vi "Beampointing_Multi_Pico.vi"() -> ()   [LabVIEW 2011]
uses:
  GUI_Template/GUI_master/tcp_new_data_event.ctl
  GUI_Template/GUI_master/tcp new data cluster.ctl
  Ctrs/beam detection.ctl
  GUI_Beampointing_single_TRA/Ctrs/move.ctl
  <vilib>/Utility/file.llb/Read From Spreadsheet File (string).vi
  <userlib>/_OpenG.lib/array/array.llb/Filter 1D Array with Scalar (String)__ogtk.vi
  <vilib>/Utility/file.llb/Write To Spreadsheet File (string).vi
  <vilib>/Analysis/NI_AALBase.lvlib
panel:
  out "millisecond timer value":u32
  out "appended path":path
  out "millisecond timer 2":u32
  in  "GUIdevice 98":string="PicoPad4"
  in  "Position.Axis 111::98":dbl=77.0 caption="Motor Axis 1" min=-20000.0 max=20000.0 format="%#_6f"
  in  "Position.Axis 112::98":dbl=77.0 caption="Motor Axis 1" min=-20000.0 max=20000.0 format="%#_6f"
  in  "Position.Axis 113::98":dbl=77.0 caption="Motor Axis 1" min=-20000.0 max=20000.0 format="%#_6f"
  in  "Position.Axis 121::98":dbl=77.0 caption="Motor Axis 1" min=-999999.0 max=999999.0 format="%#_6f"
  in  "Position.Axis 122::98":dbl=77.0 caption="Motor Axis 1" min=-999999.0 max=999999.0 format="%#_6f"
  in  "Position.Axis 123::98":dbl=77.0 caption="Motor Axis 1" min=-999999.0 max=999999.0 format="%#_6f"
  in  "Position.Axis 131::98":dbl=77.0 caption="Motor Axis 1" min=-999999.0 max=999999.0 format="%#_6f"
  in  "Position.Axis 132::98":dbl=77.0 caption="Motor Axis 1" min=-999999.0 max=999999.0 format="%#_6f"
  in  "Position.Axis 133::98":dbl=77.0 caption="Motor Axis 1" min=-999999.0 max=999999.0 format="%#_6f"
  in  "Position.Axis 141::98":dbl=77.0 caption="Motor Axis 1" min=-999999.0 max=999999.0 format="%#_6f"
  in  "Position.Axis 142::98":dbl=77.0 caption="Motor Axis 1" min=-999999.0 max=999999.0 format="%#_6f"
  in  "Position.Axis 143::98":dbl=77.0 caption="Motor Axis 1" min=-999999.0 max=999999.0 format="%#_6f"
  in  "Position.Axis 211::98":dbl=77.0 caption="Motor Axis 1" min=-999999.0 max=999999.0 format="%#_6f"
  in  "Position.Axis 212::98":dbl=77.0 caption="Motor Axis 1" min=-999999.0 max=999999.0 format="%#_6f"
  in  "Position.Axis 213::98":dbl=77.0 caption="Motor Axis 1" min=-999999.0 max=999999.0 format="%#_6f"
  in  "Position.Axis 221::98":dbl=77.0 caption="Motor Axis 1" min=-999999.0 max=999999.0 format="%#_6f"
  in  "Position.Axis 222::98":dbl=77.0 caption="Motor Axis 1" min=-999999.0 max=999999.0 format="%#_6f"
  in  "Position.Axis 223::98":dbl=77.0 caption="Motor Axis 1" min=-999999.0 max=999999.0 format="%#_6f"
  in  "Position.Axis 231::98":dbl=77.0 caption="Motor Axis 1" min=-999999.0 max=999999.0 format="%#_6f"
  in  "Position.Axis 232::98":dbl=77.0 caption="Motor Axis 1" min=-999999.0 max=999999.0 format="%#_6f"
  in  "Position.Axis 233::98":dbl=77.0 caption="Motor Axis 1" min=-999999.0 max=999999.0 format="%#_6f"
  in  "Position.Axis 241::98":dbl=77.0 caption="Motor Axis 1" min=-999999.0 max=999999.0 format="%#_6f"
  in  "Position.Axis 242::98":dbl=77.0 caption="Motor Axis 1" min=-999999.0 max=999999.0 format="%#_6f"
  in  "Position.Axis 243::98":dbl=77.0 caption="Motor Axis 1" min=-999999.0 max=999999.0 format="%#_6f"
  in  "Position.Axis 311::98":dbl=77.0 caption="Motor Axis 1" min=-999999.0 max=999999.0 format="%#_6f"
  in  "Position.Axis 312::98":dbl=77.0 caption="Motor Axis 1" min=-999999.0 max=999999.0 format="%#_6f"
  in  "Position.Axis 313::98":dbl=77.0 caption="Motor Axis 1" min=-999999.0 max=999999.0 format="%#_6f"
  in  "Position.Axis 321::98":dbl=77.0 caption="Motor Axis 1" min=-999999.0 max=999999.0 format="%#_6f"
  in  "Position.Axis 322::98":dbl=77.0 caption="Motor Axis 1" min=-999999.0 max=999999.0 format="%#_6f"
  in  "Position.Axis 323::98":dbl=77.0 caption="Motor Axis 1" min=-999999.0 max=999999.0 format="%#_6f"
  in  "Position.Axis 331::98":dbl=77.0 caption="Motor Axis 1" min=-999999.0 max=999999.0 format="%#_6f"
  in  "Position.Axis 332::98":dbl=77.0 caption="Motor Axis 1" min=-999999.0 max=999999.0 format="%#_6f"
  in  "Position.Axis 333::98":dbl=77.0 caption="Motor Axis 1" min=-999999.0 max=999999.0 format="%#_6f"
  in  "Position.Axis 341::98":dbl=77.0 caption="Motor Axis 1" min=-999999.0 max=999999.0 format="%#_6f"
  in  "Position.Axis 342::98":dbl=77.0 caption="Motor Axis 1" min=-999999.0 max=999999.0 format="%#_6f"
  in  "Position.Axis 343::98":dbl=77.0 caption="Motor Axis 1" min=-999999.0 max=999999.0 format="%#_6f"
  in  "Position.Axis 411::98":dbl=77.0 caption="Motor Axis 1" min=-999999.0 max=999999.0 format="%#_6f"
  in  "Position.Axis 412::98":dbl=77.0 caption="Motor Axis 1" min=-999999.0 max=999999.0 format="%#_6f"
  in  "Position.Axis 413::98":dbl=77.0 caption="Motor Axis 1" min=-999999.0 max=999999.0 format="%#_6f"
  in  "Position.Axis 421::98":dbl=77.0 caption="Motor Axis 1" min=-999999.0 max=999999.0 format="%#_6f"
  in  "Position.Axis 422::98":dbl=77.0 caption="Motor Axis 1" min=-999999.0 max=999999.0 format="%#_6f"
  in  "Position.Axis 423::98":dbl=77.0 caption="Motor Axis 1" min=-999999.0 max=999999.0 format="%#_6f"
  in  "Position.Axis 431::98":dbl=77.0 caption="Motor Axis 1" min=-999999.0 max=999999.0 format="%#_6f"
  in  "Position.Axis 432::98":dbl=77.0 caption="Motor Axis 1" min=-999999.0 max=999999.0 format="%#_6f"
  in  "Position.Axis 433::98":dbl=77.0 caption="Motor Axis 1" min=-999999.0 max=999999.0 format="%#_6f"
  in  "Position.Axis 441::98":dbl=77.0 caption="Motor Axis 1" min=-999999.0 max=999999.0 format="%#_6f"
  in  "Position.Axis 442::98":dbl=77.0 caption="Motor Axis 1" min=-999999.0 max=999999.0 format="%#_6f"
  in  "Position.Axis 443::98":dbl=77.0 caption="Motor Axis 1" min=-999999.0 max=999999.0 format="%#_6f"
  in  "Position.Axis 511::98":dbl=77.0 caption="Motor Axis 1" min=-999999.0 max=999999.0 format="%#_6f"
  in  "Position.Axis 512::98":dbl=77.0 caption="Motor Axis 1" min=-999999.0 max=999999.0 format="%#_6f"
  in  "Position.Axis 513::98":dbl=77.0 caption="Motor Axis 1" min=-999999.0 max=999999.0 format="%#_6f"
  in  "Position.Axis 521::98":dbl=77.0 caption="Motor Axis 1" min=-999999.0 max=999999.0 format="%#_6f"
  in  "Position.Axis 522::98":dbl=77.0 caption="Motor Axis 1" min=-999999.0 max=999999.0 format="%#_6f"
  in  "Position.Axis 523::98":dbl=77.0 caption="Motor Axis 1" min=-999999.0 max=999999.0 format="%#_6f"
  in  "Position.Axis 531::98":dbl=77.0 caption="Motor Axis 1" min=-999999.0 max=999999.0 format="%#_6f"
  in  "Position.Axis 532::98":dbl=77.0 caption="Motor Axis 1" min=-999999.0 max=999999.0 format="%#_6f"
  in  "Position.Axis 533::98":dbl=77.0 caption="Motor Axis 1" min=-999999.0 max=999999.0 format="%#_6f"
  in  "Position.Axis 541::98":dbl=77.0 caption="Motor Axis 1" min=-999999.0 max=999999.0 format="%#_6f"
  in  "Position.Axis 542::98":dbl=77.0 caption="Motor Axis 1" min=-999999.0 max=999999.0 format="%#_6f"
  in  "Position.Axis 543::98":dbl=77.0 caption="Motor Axis 1" min=-999999.0 max=999999.0 format="%#_6f"
  in  "Numeric":dbl
  out "Current State":string
  in  "output cluster 2":T4 {"detection para"."smal para"."Measurement Parameter" items=["Center of Mass X", "Center of Mass Y", "First Pixel X", "First Pixel Y", "Bounding Rect Left", "Bounding Rect Top", "Bounding Rect Right", "Bounding Rect Bottom", "Max Feret Diameter Start X", "Max Feret Diameter Start Y", "Max Feret Diameter End X", "Max Feret Diameter End Y", "Max Horiz. Segment Length Left", "Max Horiz. Segment Length Right", "Max Horiz. Segment Length Row", "-", "Bounding Rect Width", "Bounding Rect Height", "Bounding Rect Diagonal", "Perimeter", "Convex Hull Perimeter", "Holes' Perimeter", "Max Feret Diameter", "Equivalent Ellipse Major Axis", "Equivalent Ellipse Minor Axis", "Equivalent Ellipse Minor Axis (Feret)", "Equivalent Rect Long Side", "Equivalent Rect Short Side", "Equivalent Rect Diagonal", "Equivalent Rect Short Side (Feret)", "Average Horiz. Segment Length", "Average Vert. Segment Length", "Hydraulic Radius", "Waddel Disk Diameter", "-", "Area", "Holes' Area", "Particle & Holes' Area", "Convex Hull Area", "Image Area", "-", "Number of Holes", "Number of Horiz. Segments", "Number of Vert. Segments", "-", "Orientation", "Max Feret Diameter Orientation", "-", "% Area/Image Area", "% Area/(Particle & Holes' Area)", "Ratio of Equivalent Ellipse Axes", "Ratio of Equivalent Rect Sides", "-", "Elongation Factor", "Compactness Factor", "Heywood Circularity Factor", "Type Factor", "-", "Sum X", "Sum Y", "Sum XX", "Sum XY", "Sum YY", "Sum XXX", "Sum XXY", "Sum XYY", "Sum YYY", "-", "Moment of Inertia XX", "Moment of Inertia XY", "Moment of Inertia YY", "Moment of Inertia XXX", "Moment of Inertia XXY", "Moment of Inertia XYY", "Moment of Inertia YYY", "Norm. Moment of Inertia XX", "Norm. Moment of Inertia XY", "Norm. Moment of Inertia YY", "Norm. Moment of Inertia XXX", "Norm. Moment of Inertia XXY", "Norm. Moment of Inertia XYY", "Norm. Moment of Inertia YYY", "Hu Moment 1", "Hu Moment 2", "Hu Moment 3", "Hu Moment 4", "Hu Moment 5", "Hu Moment 6", "Hu Moment 7"]; "detection para"."smal para"."Range Lower Value" format="%.2f"; "detection para"."smal para"."Range Upper Value" format="%.2f"; "detection para"."detection method" items=["clustering", "entropy", "metric", "moments", "inter-class variance"]; "detection para"."Filter" items=["No Filter", "Median Filter", "Low Pass Filter"]}
  out "CCDs":string[](array[string])
  in  "GUIdevice 12":string
  in  "GUIdevice 11":string
  in  "GUIdevice 10":string
  in  "GUIdevice 9":string
  out "detected 2":string[](array[string])
  out "error out 2":errorcluster
  in  "active cams":string[](array[string])
  in  "Motor Y":dbl[][](array[numeric])
  in  "Motor X":dbl[][](array[numeric])
  out "Names":string[](array[string])
  in  "Offset X stats":dbl[][](array[numeric])
  in  "Offset Y stats":dbl[][](array[numeric])
  out "Box":T5(array[cluster])
  in  "Tab Control 2":enum32{"Config ", "Main", "History"}(tab)=enum."Main"
  out "Waveform Chart":u32(graph)
  in  "associated motors":T6
  out "Cameras":T7
  out "Status":cluster{i32, i32, "Centroid X":dbl[][]}(graph)
  in  "Exposure:12":dbl=0.095 min=0.0001 max=1.0 format="%#_6f"
  in  "Triggerdelay::12":dbl=0.003 min=0.0 max=0.09 format="%#_6f"
  in  "Exposure::11":dbl=0.095 min=0.0001 max=1.0 format="%#_6f"
  in  "Triggerdelay::11":dbl=0.003 min=0.0 max=0.09 format="%#_6f"
  in  "Exposure::10":dbl=0.095 min=0.0001 max=1.0 format="%#_6f"
  in  "Triggerdelay::10":dbl=0.003 min=0.0 max=0.09 format="%#_6f"
  in  "Exposure::9":dbl=0.095 min=0.0001 max=1.0 format="%#_6f"
  in  "Triggerdelay::9":dbl=0.003 min=0.0 max=0.09 format="%#_6f"
  in  "Trigger::9":bool
  in  "Trigger::10":bool caption="Trigger:10"
  in  "Trigger::11":bool
  in  "Trigger::12":bool
  in  "Target.Y::9":dbl=45.0 caption="T9y" min=0.0 max=2000.0 format="%#_6f"
  in  "Target.X::9":dbl=47.0 caption="Tx9" min=0.0 max=2000.0 format="%#_6f"
  in  "Target.Y::10":dbl=45.0 caption="T10y" min=0.0 max=2000.0 format="%#_6f"
  in  "Target.X::10":dbl=47.0 caption="T10x" min=0.0 max=2000.0 format="%#_6f"
  in  "Target.Y::11":dbl=45.0 caption="T11y" min=0.0 max=2000.0 format="%#_6f"
  in  "Target.X::11":dbl=47.0 caption="T11x" min=0.0 max=2000.0 format="%#_6f"
  in  "Target.Y::12":dbl=45.0 caption="T12y" min=0.0 max=2000.0 format="%#_6f"
  in  "Target.X::12":dbl=47.0 caption="T12x" min=0.0 max=2000.0 format="%#_6f"
  in  "Exposure::8":dbl=0.095 min=0.01 max=1.0 format="%#_6f"
  in  "Triggerdelay::8":dbl=0.003 min=0.0 max=0.09 format="%#_6f"
  in  "Trigger::8":bool
  in  "Target.Y::8":dbl=45.0 caption="T8y" min=0.0 max=2000.0 format="%#_6f"
  in  "Target.X::8":dbl=47.0 caption="T8x" min=0.0 max=2000.0 format="%#_6f"
  in  "Target.Y::7":dbl=45.0 caption="T7x" min=0.0 max=2000.0 format="%#_6f"
  in  "Target.X::7":dbl=47.0 caption="T7y" min=0.0 max=2000.0 format="%#_6f"
  in  "Target.Y::6":dbl=45.0 caption="T6y" min=0.0 max=2000.0 format="%#_6f"
  in  "Target.X::6":dbl=47.0 caption="T6x" min=0.0 max=2000.0 format="%#_6f"
  in  "Target.Y::5":dbl=45.0 caption="T5y" min=0.0 max=2000.0 format="%#_6f"
  in  "Target.X::5":dbl=47.0 caption="T5x" min=0.0 max=2000.0 format="%#_6f"
  in  "Target.Y::4":dbl=45.0 caption="T4y" min=0.0 max=2000.0 format="%#_6f"
  in  "Target.X::4":dbl=47.0 caption="T4x" min=0.0 max=2000.0 format="%#_6f"
  in  "Target.Y::3":dbl=163.0 caption="T3y" min=0.0 max=2000.0 format="%#_6f"
  in  "Target.X::3":dbl=152.0 caption="T3x" min=0.0 max=2000.0 format="%#_6f"
  in  "Target.Y::2":dbl=74.0 caption="T2y" min=1.0 max=600.0 format="%#_6f"
  in  "Target.X::2":dbl=75.0 caption="T2x" min=1.0 max=800.0 format="%#_6f"
  in  "Target.Y::1":dbl=61.0 caption="T1y" min=1.0 max=600.0 format="%#_6f"
  in  "Target.X::1":dbl=77.0 caption="T1x" min=1.0 max=800.0 format="%#_6f"
  in  "Exposure::7":dbl=0.095 min=0.0001 max=1.0 format="%#_6f"
  in  "Triggerdelay::7":dbl=0.003 min=0.0 max=0.09 format="%#_6f"
  in  "Trigger::7":bool
  in  "Exposure::6":dbl=0.095 min=0.0001 max=1.0 format="%#_6f"
  in  "Triggerdelay::6":dbl=0.003 min=0.0 max=0.09 format="%#_6f"
  in  "Trigger::6":bool
  in  "Exposure::5":dbl=0.095 min=0.0001 max=1.0 format="%#_6f"
  in  "Triggerdelay::5":dbl=0.003 min=0.0 max=0.09 format="%#_6f"
  in  "Trigger::5":bool
  in  "Exposure::4":dbl=0.095 min=0.0001 max=1.0 format="%#_6f"
  in  "Triggerdelay::4":dbl=0.003 min=0.0 max=0.09 format="%#_6f"
  in  "Trigger::4":bool
  in  "Exposure::3":dbl=0.095 min=0.0001 max=1.0 format="%#_6f"
  in  "Triggerdelay::3":dbl=0.003 min=0.0 max=0.09 format="%#_6f"
  in  "Trigger::3":bool
  in  "Exposure::2":dbl=0.095 min=0.0001 max=1.0 format="%#_6f"
  in  "Triggerdelay::2":dbl=0.003 min=0.0 max=0.09 format="%#_6f"
  in  "Trigger::2":bool
  out "image::1":T8(plugin-control) caption="PA2_Input1"
  out "image::2":T8(plugin-control) caption="PA2_Input2"
  out "image::3":T8(plugin-control) caption="L1_TelInpNear"
  out "image::4":T8(plugin-control) caption="L2_TelInpFar"
  out "image::5":T8(plugin-control) caption="L4_TREXpass1"
  out "image::6":T8(plugin-control) caption="L5_TREXPass2"
  out "image::7":T8(plugin-control) caption="L6_TREXpass3"
  out "image::8":T8(plugin-control) caption="L7_TREXPass4"
  in  "Exposure::1":dbl=0.095 min=0.0001 max=1.0 format="%#_6f"
  in  "Triggerdelay::1":dbl=0.003 min=0.0 max=0.09 format="%#_6f"
  in  "Trigger::1":bool
  in  "UDP error message":string
  out "required Y":bool[](array[boolean])
  out "required X":bool[](array[boolean])
  out "detected":bool[](array[boolean])
  out "name array":string[](array[string])
  out "image::9":T8(plugin-control) caption="L8_M10Leak"
  out "image::10":T8(plugin-control) caption="B1_TelInput"
  out "image::11":T8(plugin-control) caption="B2_TelLens1"
  out "image::12":T8(plugin-control) caption="B5_CompressorOut"
  out "CCD 9":cluster{timestamp[], dbl[]}[](graph)
  out "CCD 10":cluster{timestamp[], dbl[]}[](graph)
  out "CCD 11":cluster{timestamp[], dbl[]}[](graph)
  out "CCD 12":cluster{timestamp[], dbl[]}[](graph)
  out "CCD 5":cluster{timestamp[], dbl[]}[](graph)
  out "CCD 6":cluster{timestamp[], dbl[]}[](graph)
  out "CCD 7":cluster{timestamp[], dbl[]}[](graph)
  out "CCD 8":cluster{timestamp[], dbl[]}[](graph)
  out "CCD 2":cluster{timestamp[], dbl[]}[](graph)
  out "CCD 1":cluster{timestamp[], dbl[]}[](graph)
  out "CCD 3":cluster{timestamp[], dbl[]}[](graph)
  out "CCD 4":cluster{timestamp[], dbl[]}[](graph)
  out "History index":i32
  in  "History Size":i32=500
  out "Particle Reports (Pixels)":T9(array[cluster])
  in  "Feedback Global":bool
  in  "detection para":T2[](array[typedef])=[{"Filter"=1, "Filter Para"={"X Size"=5, "Y Size"=5, "% Tolerance"=1}, "detection method"=4, "smal para"=[{"Measurement Parameter"=35, "Range Lower Value"=0.0, "Range Upper Value"=0.0, "Range"=TRUE, "Measurement Type"=FALSE}], "Remove small Objects"=TRUE, "Restrict to round Objects"=FALSE}, {"Filter"=1, "Filter Para"={"X Size"=5, "Y Size"=5, "% Tolerance"=1}, "detection method"=4, "smal para"=[{"Measurement Parameter"=35, "Range Lower Value"=0.0, "Range Upper Value"=500.0, "Range"=FALSE, "Measurement Type"=FALSE}], "Remove small Objects"=TRUE, "Restrict to round Objects"=FALSE}, {"Filter"=1, "Filter Para"={"X Size"=5, "Y Size"=5, "% Tolerance"=1}, "detection method"=4, "smal para"=[{"Measurement Parameter"=35, "Range Lower Value"=0.0, "Range Upper Value"=500.0, "Range"=TRUE, "Measurement Type"=FALSE}], "Remove small Objects"=TRUE, "Restrict to round Objects"=FALSE}, {"Filter"=1, "Filter Para"={"X Size"=5, "Y Size"=5, "% Tolerance"=1}, "detection method"=4, "smal para"=[{"Measurement Parameter"=35, "Range Lower Value"=0.0, "Range Upper Value"=500.0, "Range"=TRUE, "Measurement Type"=FALSE}], "Remove small Objects"=TRUE, "Restrict to round Objects"=FALSE}, {"Filter"=1, "Filter Para"={"X Size"=5, "Y Size"=5, "% Tolerance"=1}, "detection method"=4, "smal para"=[{"Measurement Parameter"=35, "Range Lower Value"=0.0, "Range Upper Value"=500.0, "Range"=TRUE, "Measurement Type"=FALSE}], "Remove small Objects"=TRUE, "Restrict to round Objects"=FALSE}, {"Filter"=1, "Filter Para"={"X Size"=5, "Y Size"=5, "% Tolerance"=1}, "detection method"=4, "smal para"=[{"Measurement Parameter"=35, "Range Lower Value"=0.0, "Range Upper Value"=500.0, "Range"=TRUE, "Measurement Type"=FALSE}], "Remove small Objects"=TRUE, "Restrict to round Objects"=FALSE}, {"Filter"=1, "Filter Para"={"X Size"=5, "Y Size"=5, "% Tolerance"=1}, "detection method"=4, "smal para"=[{"Measurement Parameter"=35, "Range Lower Value"=0.0, "Range Upper Value"=500.0, "Range"=TRUE, "Measurement Type"=FALSE}], "Remove small Objects"=TRUE, "Restrict to round Objects"=FALSE}, {"Filter"=1, "Filter Para"={"X Size"=5, "Y Size"=5, "% Tolerance"=1}, "detection method"=3, "smal para"=[{"Measurement Parameter"=35, "Range Lower Value"=0.0, "Range Upper Value"=0.0, "Range"=FALSE, "Measurement Type"=FALSE}], "Remove small Objects"=TRUE, "Restrict to round Objects"=FALSE}, {"Filter"=1, "Filter Para"={"X Size"=5, "Y Size"=5, "% Tolerance"=1}, "detection method"=4, "smal para"=[{"Measurement Parameter"=35, "Range Lower Value"=0.0, "Range Upper Value"=0.0, "Range"=FALSE, "Measurement Type"=FALSE}], "Remove small Objects"=TRUE, "Restrict to round Objects"=FALSE}, {"Filter"=1, "Filter Para"={"X Size"=5, "Y Size"=5, "% Tolerance"=1}, "detection method"=4, "smal para"=[{"Measurement Parameter"=35, "Range Lower Value"=0.0, "Range Upper Value"=500.0, "Range"=TRUE, "Measurement Type"=FALSE}], "Remove small Objects"=TRUE, "Restrict to round Objects"=FALSE}, {"Filter"=1, "Filter Para"={"X Size"=5, "Y Size"=5, "% Tolerance"=1}, "detection method"=4, "smal para"=[{"Measurement Parameter"=35, "Range Lower Value"=0.0, "Range Upper Value"=500.0, "Range"=TRUE, "Measurement Type"=FALSE}], "Remove small Objects"=TRUE, "Restrict to round Objects"=FALSE}, {"Filter"=1, "Filter Para"={"X Size"=5, "Y Size"=5, "% Tolerance"=1}, "detection method"=4, "smal para"=[{"Measurement Parameter"=35, "Range Lower Value"=0.0, "Range Upper Value"=500.0, "Range"=TRUE, "Measurement Type"=FALSE}], "Remove small Objects"=TRUE, "Restrict to round Objects"=FALSE}] {"smal para"."Measurement Parameter" items=["Center of Mass X", "Center of Mass Y", "First Pixel X", "First Pixel Y", "Bounding Rect Left", "Bounding Rect Top", "Bounding Rect Right", "Bounding Rect Bottom", "Max Feret Diameter Start X", "Max Feret Diameter Start Y", "Max Feret Diameter End X", "Max Feret Diameter End Y", "Max Horiz. Segment Length Left", "Max Horiz. Segment Length Right", "Max Horiz. Segment Length Row", "-", "Bounding Rect Width", "Bounding Rect Height", "Bounding Rect Diagonal", "Perimeter", "Convex Hull Perimeter", "Holes' Perimeter", "Max Feret Diameter", "Equivalent Ellipse Major Axis", "Equivalent Ellipse Minor Axis", "Equivalent Ellipse Minor Axis (Feret)", "Equivalent Rect Long Side", "Equivalent Rect Short Side", "Equivalent Rect Diagonal", "Equivalent Rect Short Side (Feret)", "Average Horiz. Segment Length", "Average Vert. Segment Length", "Hydraulic Radius", "Waddel Disk Diameter", "-", "Area", "Holes' Area", "Particle & Holes' Area", "Convex Hull Area", "Image Area", "-", "Number of Holes", "Number of Horiz. Segments", "Number of Vert. Segments", "-", "Orientation", "Max Feret Diameter Orientation", "-", "% Area/Image Area", "% Area/(Particle & Holes' Area)", "Ratio of Equivalent Ellipse Axes", "Ratio of Equivalent Rect Sides", "-", "Elongation Factor", "Compactness Factor", "Heywood Circularity Factor", "Type Factor", "-", "Sum X", "Sum Y", "Sum XX", "Sum XY", "Sum YY", "Sum XXX", "Sum XXY", "Sum XYY", "Sum YYY", "-", "Moment of Inertia XX", "Moment of Inertia XY", "Moment of Inertia YY", "Moment of Inertia XXX", "Moment of Inertia XXY", "Moment of Inertia XYY", "Moment of Inertia YYY", "Norm. Moment of Inertia XX", "Norm. Moment of Inertia XY", "Norm. Moment of Inertia YY", "Norm. Moment of Inertia XXX", "Norm. Moment of Inertia XXY", "Norm. Moment of Inertia XYY", "Norm. Moment of Inertia YYY", "Hu Moment 1", "Hu Moment 2", "Hu Moment 3", "Hu Moment 4", "Hu Moment 5", "Hu Moment 6", "Hu Moment 7"]; "smal para"."Range Lower Value" format="%.2f"; "smal para"."Range Upper Value" format="%.2f"; "detection method" items=["clustering", "entropy", "metric", "moments", "inter-class variance"]; "Filter" items=["No Filter", "Median Filter", "Low Pass Filter"]}
  in  "GUIdevice 8":string="B5_CompressorOut"
  in  "Tab Control":T10(tab)=enum."Detection"
  in  "Center":bool
  in  "Save Stats":bool
  in  "Save Config":bool
  in  "Load Config":bool
  in  "update speed [ms]":i32=200
  in  "img to avg":i32=20
  in  "Reset History":bool
  in  "save path":path=path "W:/BP_DATA"
  in  "autodetect":bool
  in  "Detection Rate":dbl=0.9 min=0.001 max=1.0
  in  "new tdms":bool
  in  "beam detection para":T2={"Filter"=1, "Filter Para"={"X Size"=5, "Y Size"=5, "% Tolerance"=1}, "detection method"=4, "smal para"=[{"Measurement Parameter"=35, "Range Lower Value"=0.0, "Range Upper Value"=500.0, "Range"=FALSE, "Measurement Type"=FALSE}], "Remove small Objects"=TRUE, "Restrict to round Objects"=FALSE} {"smal para"."Measurement Parameter" items=["Center of Mass X", "Center of Mass Y", "First Pixel X", "First Pixel Y", "Bounding Rect Left", "Bounding Rect Top", "Bounding Rect Right", "Bounding Rect Bottom", "Max Feret Diameter Start X", "Max Feret Diameter Start Y", "Max Feret Diameter End X", "Max Feret Diameter End Y", "Max Horiz. Segment Length Left", "Max Horiz. Segment Length Right", "Max Horiz. Segment Length Row", "-", "Bounding Rect Width", "Bounding Rect Height", "Bounding Rect Diagonal", "Perimeter", "Convex Hull Perimeter", "Holes' Perimeter", "Max Feret Diameter", "Equivalent Ellipse Major Axis", "Equivalent Ellipse Minor Axis", "Equivalent Ellipse Minor Axis (Feret)", "Equivalent Rect Long Side", "Equivalent Rect Short Side", "Equivalent Rect Diagonal", "Equivalent Rect Short Side (Feret)", "Average Horiz. Segment Length", "Average Vert. Segment Length", "Hydraulic Radius", "Waddel Disk Diameter", "-", "Area", "Holes' Area", "Particle & Holes' Area", "Convex Hull Area", "Image Area", "-", "Number of Holes", "Number of Horiz. Segments", "Number of Vert. Segments", "-", "Orientation", "Max Feret Diameter Orientation", "-", "% Area/Image Area", "% Area/(Particle & Holes' Area)", "Ratio of Equivalent Ellipse Axes", "Ratio of Equivalent Rect Sides", "-", "Elongation Factor", "Compactness Factor", "Heywood Circularity Factor", "Type Factor", "-", "Sum X", "Sum Y", "Sum XX", "Sum XY", "Sum YY", "Sum XXX", "Sum XXY", "Sum XYY", "Sum YYY", "-", "Moment of Inertia XX", "Moment of Inertia XY", "Moment of Inertia YY", "Moment of Inertia XXX", "Moment of Inertia XXY", "Moment of Inertia XYY", "Moment of Inertia YYY", "Norm. Moment of Inertia XX", "Norm. Moment of Inertia XY", "Norm. Moment of Inertia YY", "Norm. Moment of Inertia XXX", "Norm. Moment of Inertia XXY", "Norm. Moment of Inertia XYY", "Norm. Moment of Inertia YYY", "Hu Moment 1", "Hu Moment 2", "Hu Moment 3", "Hu Moment 4", "Hu Moment 5", "Hu Moment 6", "Hu Moment 7"]; "smal para"."Range Lower Value" format="%.2f"; "smal para"."Range Upper Value" format="%.2f"; "detection method" items=["clustering", "entropy", "metric", "moments", "inter-class variance"]; "Filter" items=["No Filter", "Median Filter", "Low Pass Filter"]}
  in  "move config":T1={"Tolerance [%]"=0.1, "Stepsize"=0.0001, "Invert Axis"=TRUE, "Invert Direction X"=FALSE, "Invert Direction Y"=TRUE, "enable feedback"=FALSE, "Set Centriod Target"=FALSE}
  out "Moving X":string
  out "Moving Y":string
  in  "ActiveMotor":u16(ring)=7 items=["PA2_Input1", "PA2_Input2", "L2_TelInpFar", "L1_TelInpNear", "L4_TREXPASS1", "L5_TREXPass2", "L6_TREXPass3", "L7_TREXPass4", "L8_M10Leak", "B1_TelInput", "B2_TelLens1", "NoName", "NoName", "NoName", "MBeamSplitterL", "Mdiode", "NoName", "NoName", "NoName", "NoName"]
  in  "ActiveMotorName::99":string
  in  "RelativeMove.Axis 1.CCW::99":bool caption="RelativeMove.Axis 1.CCW::1"
  in  "RelativeMove.Axis 1.CW::99":bool caption="RelativeMove.Axis 1.CW::1"
  in  "RelativeMove.Axis 2.CCW::99":bool caption="RelativeMove.Axis. 2.CCW::1"
  in  "RelativeMove.Axis 2.CW::99":bool caption="RelativeMove.Axis 2.CW::1"
  in  "RelativeSettings.Axis 1.Position::99":dbl caption="Axis 1 Position" min=-999999.0 max=999999.0 format="%_4p"
  in  "RelativeSettings.Axis 2.Position::99":dbl caption="Axis 2 Position" min=-999999.0 max=999999.0 format="%_4p"
  in  "RelativeSettings.Axis 2.StepSize::99":dbl=50.0 caption="Axis 2 StepSize" min=0.0 max=999999.0 format="%_4p"
  in  "RelativeSettings.Axis 1.StepSize::99":dbl=50.0 caption="Axis 1 Stepsize" min=0.0 max=999999.0 format="%_4p"
  in  "RelativeSettings.Axis 1.StepSize::98":dbl=50.0 caption="Axis 1 Stepsize" min=0.0 max=999999.0 format="%_4p"
  in  "RelativeSettings.Axis 2.StepSize::98":dbl=50.0 caption="Axis 2 StepSize" min=0.0 max=999999.0 format="%_4p"
  in  "RelativeSettings.Axis 2.Position::98":dbl caption="Axis 2 Position" min=-999999.0 max=999999.0 format="%_4p"
  in  "RelativeSettings.Axis 1.Position::98":dbl caption="Axis 1 Position" min=-999999.0 max=999999.0 format="%_4p"
  in  "RelativeMove.Axis 2.CW::98":bool caption="RelativeMove.Axis 2.CW::1"
  in  "RelativeMove.Axis 2.CCW::98":bool caption="RelativeMove.Axis. 2.CCW::1"
  in  "RelativeMove.Axis 1.CW::98":bool caption="RelativeMove.Axis 1.CW::1"
  in  "RelativeMove.Axis 1.CCW::98":bool caption="RelativeMove.Axis 1.CCW::1"
  in  "ActiveMotorName::98":string
  in  "ActiveMotor 2":u16(ring)=7
  out "Arguments Y":string
  in  "active axis refs 2":T11(array[cluster])
  in  "active Axis ref":cluster{"Ref X":refnum<vi>, "Ref Y":refnum<vi>}
  in  "CCDs":u16(ring) items=["PA2_Input1", "PA2_Input2", "L1_TelInpNear", "L2_TelInpFar", "L4_TREXpass1", "L5_TREXPass2", "L6_TREXpass3", "L7_TREXPass4", "L8_M10Leak", "B1_TelInput", "B2_TelLens1", "B5_CompressorOut"]
  out "motor refs":refnum<vi>[](array[refnum])
  in  "Position.Axis 511::99":dbl=77.0 caption="Motor Axis 1" min=-20000.0 max=20000.0 format="%#_6f"
  in  "Position.Axis 512::99":dbl=77.0 caption="Motor Axis 1" min=-20000.0 max=20000.0 format="%#_6f"
  in  "Position.Axis 513::99":dbl=77.0 caption="Motor Axis 1" min=-20000.0 max=20000.0 format="%#_6f"
  in  "Position.Axis 521::99":dbl=77.0 caption="Motor Axis 1" min=-20000.0 max=20000.0 format="%#_6f"
  in  "Position.Axis 522::99":dbl=77.0 caption="Motor Axis 1" min=-20000.0 max=20000.0 format="%#_6f"
  in  "Position.Axis 523::99":dbl=77.0 caption="Motor Axis 1" min=-20000.0 max=20000.0 format="%#_6f"
  in  "Position.Axis 531::99":dbl=77.0 caption="Motor Axis 1" min=-20000.0 max=20000.0 format="%#_6f"
  in  "Position.Axis 532::99":dbl=77.0 caption="Motor Axis 1" min=-20000.0 max=20000.0 format="%#_6f"
  in  "Position.Axis 533::99":dbl=77.0 caption="Motor Axis 1" min=-20000.0 max=20000.0 format="%#_6f"
  in  "Position.Axis 541::99":dbl=77.0 caption="Motor Axis 1" min=-20000.0 max=20000.0 format="%#_6f"
  in  "Position.Axis 542::99":dbl=77.0 caption="Motor Axis 1" min=-20000.0 max=20000.0 format="%#_6f"
  in  "Position.Axis 543::99":dbl=77.0 caption="Motor Axis 1" min=-20000.0 max=20000.0 format="%#_6f"
  in  "Position.Axis 411::99":dbl=77.0 caption="Motor Axis 1" min=-20000.0 max=20000.0 format="%#_6f"
  in  "Position.Axis 412::99":dbl=77.0 caption="Motor Axis 1" min=-20000.0 max=20000.0 format="%#_6f"
  in  "Position.Axis 413::99":dbl=77.0 caption="Motor Axis 1" min=-20000.0 max=20000.0 format="%#_6f"
  in  "Position.Axis 421::99":dbl=77.0 caption="Motor Axis 1" min=-20000.0 max=20000.0 format="%#_6f"
  in  "Position.Axis 422::99":dbl=77.0 caption="Motor Axis 1" min=-20000.0 max=20000.0 format="%#_6f"
  in  "Position.Axis 423::99":dbl=77.0 caption="Motor Axis 1" min=-20000.0 max=20000.0 format="%#_6f"
  in  "Position.Axis 431::99":dbl=77.0 caption="Motor Axis 1" min=-20000.0 max=20000.0 format="%#_6f"
  in  "Position.Axis 432::99":dbl=77.0 caption="Motor Axis 1" min=-20000.0 max=20000.0 format="%#_6f"
  in  "Position.Axis 433::99":dbl=77.0 caption="Motor Axis 1" min=-20000.0 max=20000.0 format="%#_6f"
  in  "Position.Axis 441::99":dbl=77.0 caption="Motor Axis 1" min=-20000.0 max=20000.0 format="%#_6f"
  in  "Position.Axis 442::99":dbl=77.0 caption="Motor Axis 1" min=-20000.0 max=20000.0 format="%#_6f"
  in  "Position.Axis 443::99":dbl=77.0 caption="Motor Axis 1" min=-20000.0 max=20000.0 format="%#_6f"
  in  "Position.Axis 311::99":dbl=77.0 caption="Motor Axis 1" min=-20000.0 max=20000.0 format="%#_6f"
  in  "Position.Axis 312::99":dbl=77.0 caption="Motor Axis 1" min=-20000.0 max=20000.0 format="%#_6f"
  in  "Position.Axis 313::99":dbl=77.0 caption="Motor Axis 1" min=-999999.0 max=999999.0 format="%#_6f"
  in  "Position.Axis 321::99":dbl=77.0 caption="Motor Axis 1" min=-20000.0 max=20000.0 format="%#_6f"
  in  "Position.Axis 322::99":dbl=77.0 caption="Motor Axis 1" min=-20000.0 max=20000.0 format="%#_6f"
  in  "Position.Axis 323::99":dbl=77.0 caption="Motor Axis 1" min=-20000.0 max=20000.0 format="%#_6f"
  in  "Position.Axis 331::99":dbl=77.0 caption="Motor Axis 1" min=-20000.0 max=20000.0 format="%#_6f"
  in  "Position.Axis 332::99":dbl=77.0 caption="Motor Axis 1" min=-20000.0 max=20000.0 format="%#_6f"
  in  "Position.Axis 333::99":dbl=77.0 caption="Motor Axis 1" min=-20000.0 max=20000.0 format="%#_6f"
  in  "Position.Axis 341::99":dbl=77.0 caption="Motor Axis 1" min=-20000.0 max=20000.0 format="%#_6f"
  in  "Position.Axis 342::99":dbl=77.0 caption="Motor Axis 1" min=-20000.0 max=20000.0 format="%#_6f"
  in  "Position.Axis 343::99":dbl=77.0 caption="Motor Axis 1" min=-20000.0 max=20000.0 format="%#_6f"
  in  "Position.Axis 241::99":dbl=77.0 caption="Motor Axis 1" min=-20000.0 max=20000.0 format="%#_6f"
  in  "Position.Axis 242::99":dbl=77.0 caption="Motor Axis 1" min=-20000.0 max=20000.0 format="%#_6f"
  in  "Position.Axis 243::99":dbl=77.0 caption="Motor Axis 1" min=-20000.0 max=20000.0 format="%#_6f"
  in  "Position.Axis 231::99":dbl=77.0 caption="Motor Axis 1" min=-20000.0 max=20000.0 format="%#_6f"
  in  "Position.Axis 232::99":dbl=77.0 caption="Motor Axis 1" min=-20000.0 max=20000.0 format="%#_6f"
  in  "Position.Axis 233::99":dbl=77.0 caption="Motor Axis 1" min=-20000.0 max=20000.0 format="%#_6f"
  in  "Position.Axis 221::99":dbl=77.0 caption="Motor Axis 1" min=-20000.0 max=20000.0 format="%#_6f"
  in  "Position.Axis 222::99":dbl=77.0 caption="Motor Axis 1" min=-20000.0 max=200000.0 format="%#_6f"
  in  "Position.Axis 223::99":dbl=77.0 caption="Motor Axis 1" min=-20000.0 max=20000.0 format="%#_6f"
  in  "Position.Axis 211::99":dbl=77.0 caption="Motor Axis 1" min=-20000.0 max=200000.0 format="%#_6f"
  in  "Position.Axis 212::99":dbl=77.0 caption="Motor Axis 1" min=-20000.0 max=20000.0 format="%#_6f"
  in  "Position.Axis 213::99":dbl=77.0 caption="Motor Axis 1" min=-20000.0 max=20000.0 format="%#_6f"
  in  "Position.Axis 141::99":dbl=77.0 caption="Motor Axis 1" min=-20000.0 max=20000.0 format="%#_6f"
  in  "Position.Axis 142::99":dbl=77.0 caption="Motor Axis 1" min=-20000.0 max=20000.0 format="%#_6f"
  in  "Position.Axis 143::99":dbl=77.0 caption="Motor Axis 1" min=-20000.0 max=20000.0 format="%#_6f"
  in  "Position.Axis 131::99":dbl=77.0 caption="Motor Axis 1" min=-20000.0 max=20000.0 format="%#_6f"
  in  "Position.Axis 132::99":dbl=77.0 caption="Motor Axis 1" min=-20000.0 max=20000.0 format="%#_6f"
  in  "Position.Axis 133::99":dbl=77.0 caption="Motor Axis 1" min=-20000.0 max=20000.0 format="%#_6f"
  in  "Position.Axis 121::99":dbl=77.0 caption="Motor Axis 1" min=-20000.0 max=20000.0 format="%#_6f"
  in  "Position.Axis 122::99":dbl=77.0 caption="Motor Axis 1" min=-20000.0 max=20000.0 format="%#_6f"
  in  "Position.Axis 123::99":dbl=77.0 caption="Motor Axis 1" min=-20000.0 max=20000.0 format="%#_6f"
  in  "Position.Axis 113::99":dbl=77.0 caption="Motor Axis 1" min=-20000.0 max=20000.0 format="%#_6f"
  in  "Position.Axis 112::99":dbl=77.0 caption="Motor Axis 1" min=-20000.0 max=20000.0 format="%#_6f"
  in  "Position.Axis 111::99":dbl=77.0 caption="Motor Axis 1" min=-20000.0 max=20000.0 format="%#_6f"
  out "Arguments X":string
  in  "GUIdevice 99":string="PicoPad3"
  in  "move properties":T1[](array[typedef])=[{"Tolerance [%]"=0.1, "Stepsize"=0.0001, "Invert Axis"=TRUE, "Invert Direction X"=FALSE, "Invert Direction Y"=TRUE, "enable feedback"=FALSE, "Set Centriod Target"=FALSE}, {"Tolerance [%]"=0.1, "Stepsize"=0.0001, "Invert Axis"=TRUE, "Invert Direction X"=FALSE, "Invert Direction Y"=TRUE, "enable feedback"=FALSE, "Set Centriod Target"=FALSE}, {"Tolerance [%]"=0.1, "Stepsize"=0.0001, "Invert Axis"=TRUE, "Invert Direction X"=FALSE, "Invert Direction Y"=TRUE, "enable feedback"=FALSE, "Set Centriod Target"=FALSE}, {"Tolerance [%]"=0.1, "Stepsize"=0.0001, "Invert Axis"=TRUE, "Invert Direction X"=FALSE, "Invert Direction Y"=TRUE, "enable feedback"=FALSE, "Set Centriod Target"=FALSE}, {"Tolerance [%]"=0.1, "Stepsize"=0.0001, "Invert Axis"=TRUE, "Invert Direction X"=FALSE, "Invert Direction Y"=TRUE, "enable feedback"=FALSE, "Set Centriod Target"=FALSE}, {"Tolerance [%]"=0.1, "Stepsize"=0.0001, "Invert Axis"=TRUE, "Invert Direction X"=FALSE, "Invert Direction Y"=TRUE, "enable feedback"=FALSE, "Set Centriod Target"=FALSE}, {"Tolerance [%]"=0.1, "Stepsize"=0.0001, "Invert Axis"=TRUE, "Invert Direction X"=FALSE, "Invert Direction Y"=TRUE, "enable feedback"=FALSE, "Set Centriod Target"=FALSE}, {"Tolerance [%]"=0.1, "Stepsize"=0.0001, "Invert Axis"=TRUE, "Invert Direction X"=FALSE, "Invert Direction Y"=TRUE, "enable feedback"=FALSE, "Set Centriod Target"=FALSE}, {"Tolerance [%]"=0.1, "Stepsize"=0.0001, "Invert Axis"=TRUE, "Invert Direction X"=FALSE, "Invert Direction Y"=TRUE, "enable feedback"=FALSE, "Set Centriod Target"=FALSE}, {"Tolerance [%]"=0.1, "Stepsize"=0.0001, "Invert Axis"=TRUE, "Invert Direction X"=FALSE, "Invert Direction Y"=TRUE, "enable feedback"=FALSE, "Set Centriod Target"=FALSE}, {"Tolerance [%]"=0.1, "Stepsize"=0.0001, "Invert Axis"=TRUE, "Invert Direction X"=FALSE, "Invert Direction Y"=TRUE, "enable feedback"=FALSE, "Set Centriod Target"=FALSE}, {"Tolerance [%]"=0.1, "Stepsize"=0.0001, "Invert Axis"=TRUE, "Invert Direction X"=FALSE, "Invert Direction Y"=TRUE, "enable feedback"=FALSE, "Set Centriod Target"=FALSE}, {"Tolerance [%]"=0.1, "Stepsize"=0.0001, "Invert Axis"=TRUE, "Invert Direction X"=FALSE, "Invert Direction Y"=TRUE, "enable feedback"=FALSE, "Set Centriod Target"=FALSE}]
  in  "Time":timestamp[][](array[timestamp])
  in  "Mean Size":dbl[][](array[numeric])
  in  "Size":dbl[][](array[numeric])
  in  "active CCDs":i32(listbox)=1
  in  "Offset Y":dbl[][](array[numeric])
  in  "Offset X":dbl[][](array[numeric])
  in  "Mean Centroid X":dbl[][](array[numeric])
  in  "Mean Centroid Y":dbl[][](array[numeric])
  in  "Centroid Y":dbl[][](array[numeric])
  in  "Centroid X":dbl[][](array[numeric])
  in  "GUIdevice 7":string="B2_TelLens1"
  in  "GUIdevice 6":string="B1_TelInput"
  in  "GUIdevice 5":string="L8_M10Leak"
  in  "GUIdevice 4":string="L7_TREXPass4"
  in  "GUIdevice 3":string="L6_TREXpass3"
  in  "GUIdevice 2":string="L5_TREXPass2"
  in  "insert tag":bool=TRUE
  in  "stop":bool
  in  "GUIdevice 1":string="L4_TREXpass1"
  out "tcp data event":T12
  out "error IO 2":errorcluster
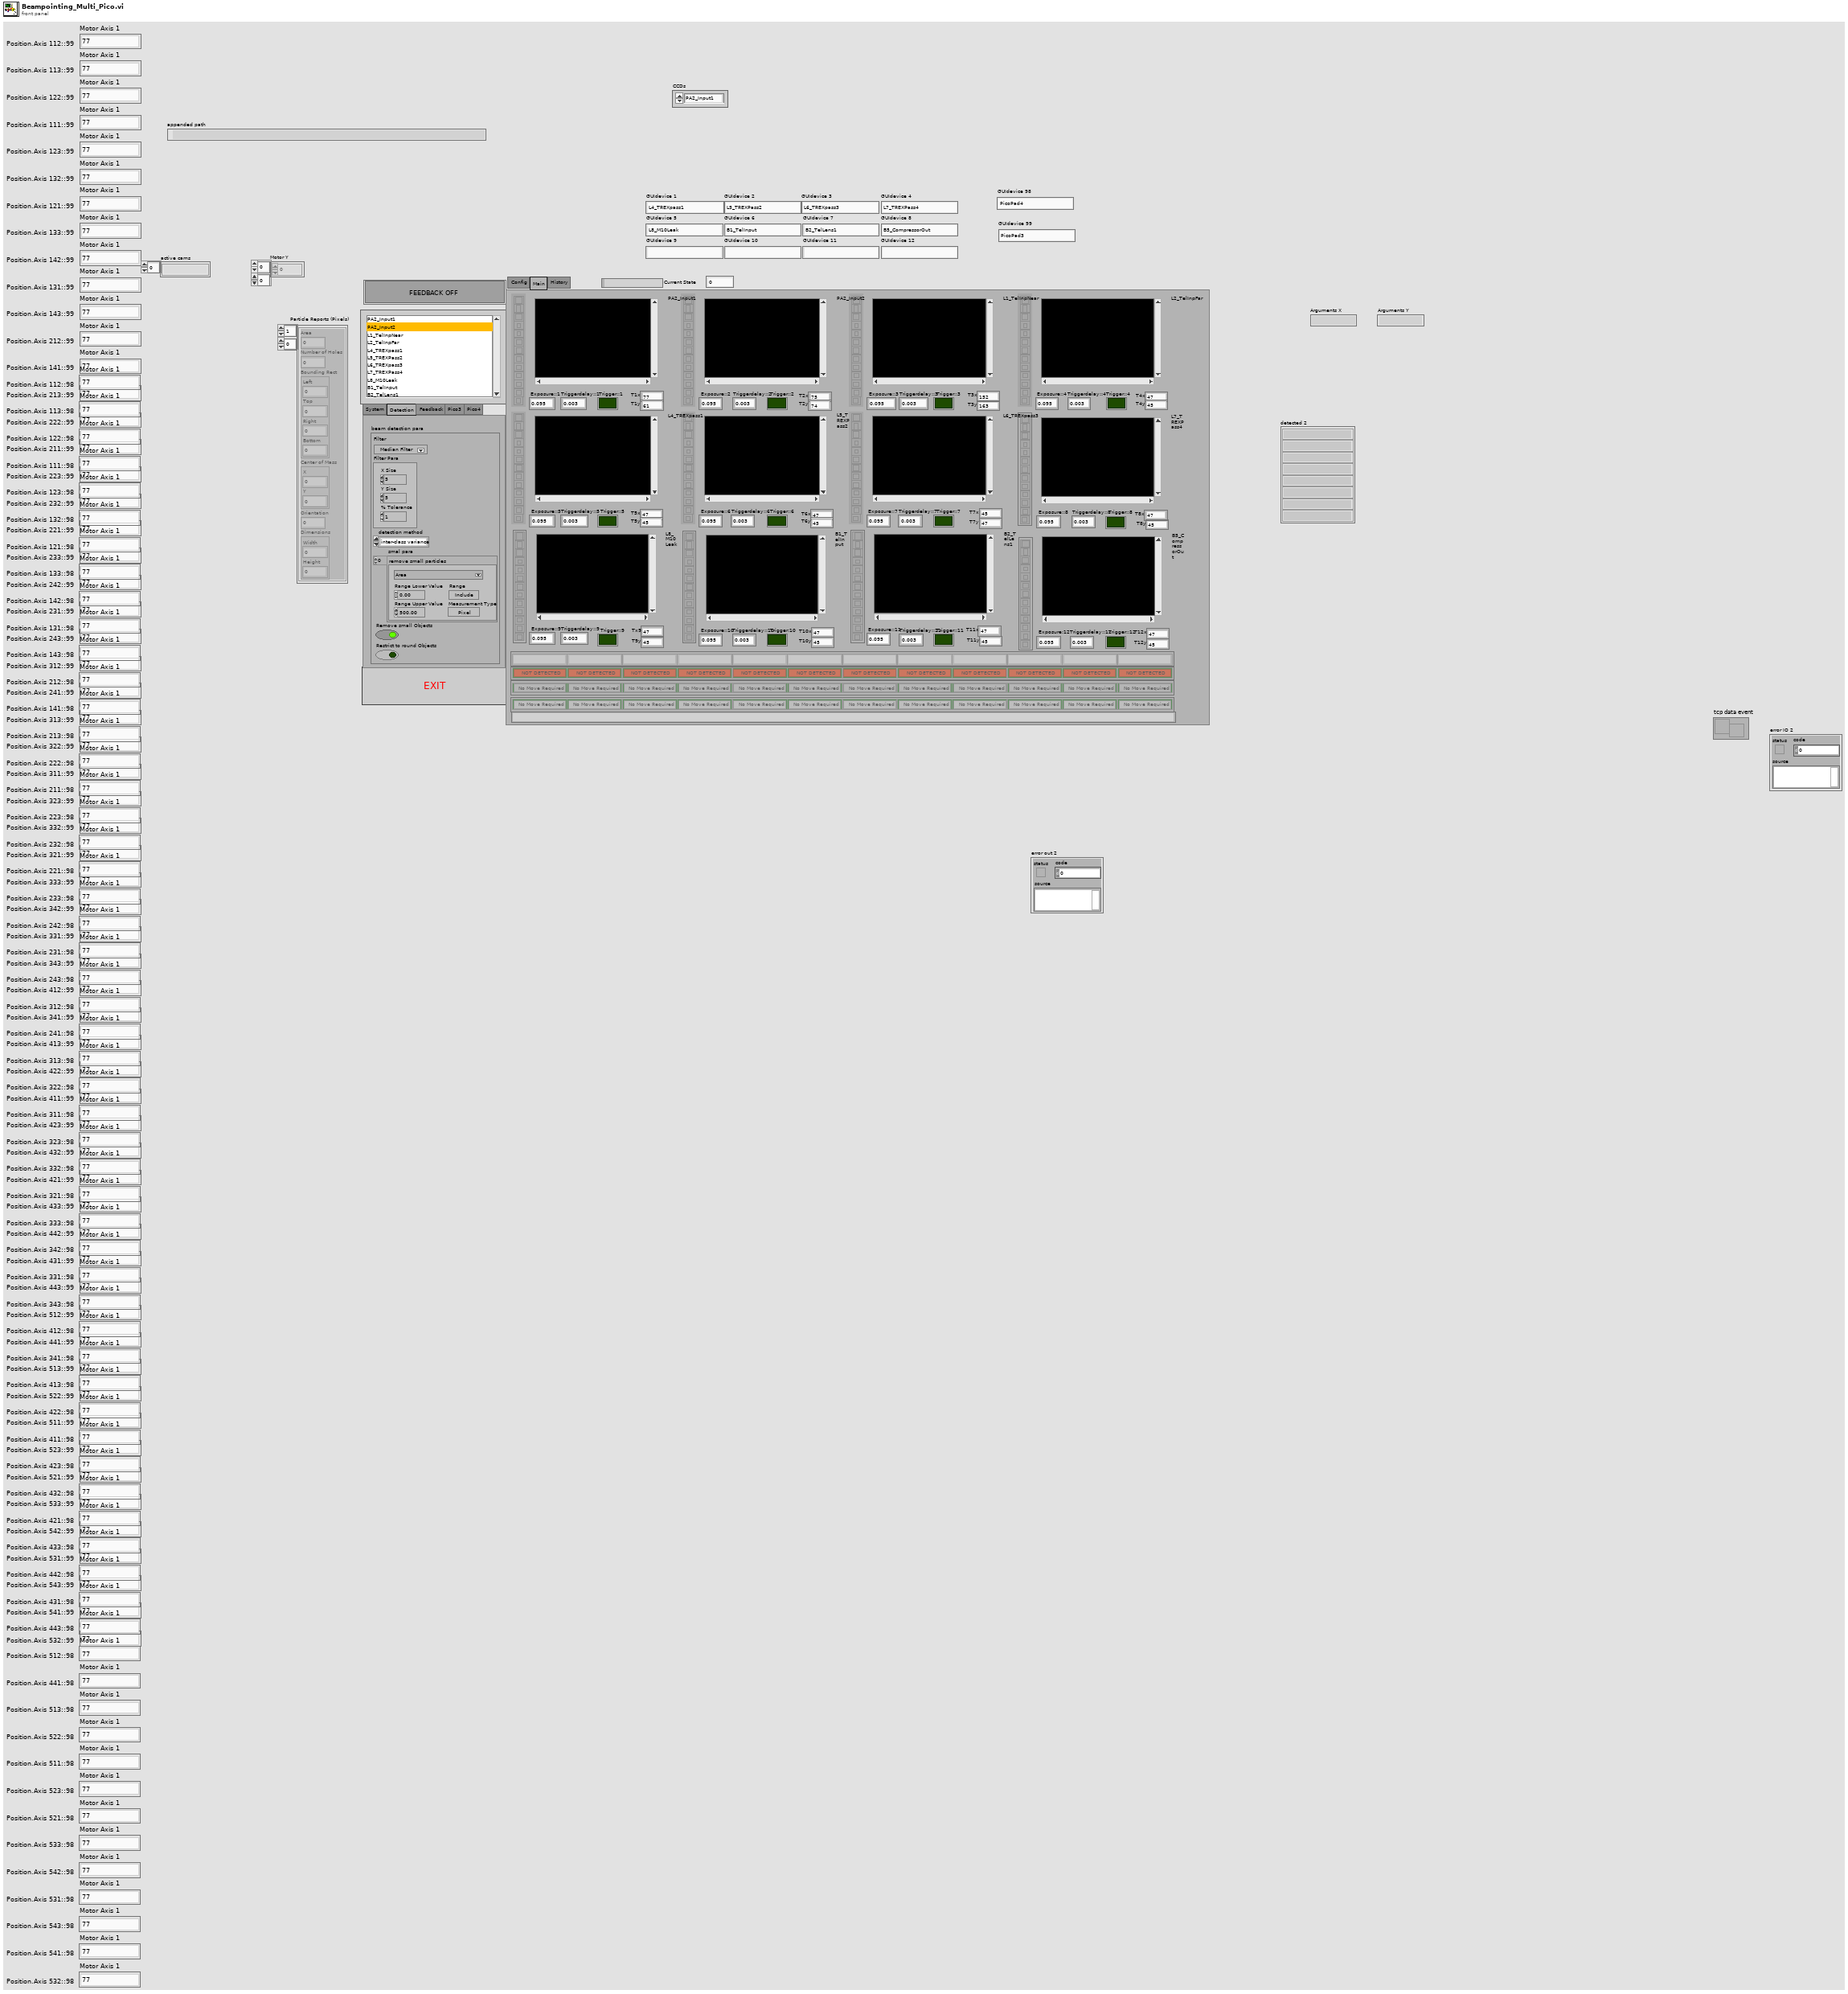
[diagram p1: front panel]
types:
  T1 = typedef "move.ctl" = cluster{"Tolerance [%]":dbl, "Stepsize":dbl, "Invert Axis":bool, "Invert Direction X":bool, "Invert Direction Y":bool, "enable feedback":bool, "Set Centriod Target":bool}
  T2 = typedef "beam detection.ctl" = cluster{"Filter":u16, "Filter Para":cluster{"X Size":i32, "Y Size":i32, "% Tolerance":i32}, "detection method":i32, "smal para":cluster{"Measurement Parameter":T3, "Range Lower Value":dbl, "Range Upper Value":dbl, "Range":bool, "Measurement Type":bool}[], "Remove small Objects":bool, "Restrict to round Objects":bool}
  T3 = typedef "Particle Parameters" = i32
  T4 = cluster{"CCDs":string[], "move properties":T1[], "detection para":T2[], "thresholds":cluster{"Lower value":sgl, "Upper value":sgl}[], "Value":cluster{"Motor CCD 1":u16, "Motor CCD 2":u16, "Motor CCD 3":u16, "Motor CCD 4":u16, "Motor CCD 5":u16, "Motor CCD 6":u16, "Motor CCD 7":u16, "Motor CCD 8":u16, "Motor CCD 9":u16, "Motor CCD 10":u16, "Motor CCD 11":u16, "Motor CCD 12":u16}}
  T5 = cluster{"Left":dbl, "Top":dbl, "Right":dbl, "Bottom":dbl}[]
  T6 = cluster{"Motor CCD 1":u16, "Motor CCD 2":u16, "Motor CCD 3":u16, "Motor CCD 4":u16, "Motor CCD 5":u16, "Motor CCD 6":u16, "Motor CCD 7":u16, "Motor CCD 8":u16, "Motor CCD 9":u16, "Motor CCD 10":u16, "Motor CCD 11":u16, "Motor CCD 12":u16}
  T7 = cluster{"[0]":string, "[1]":string, "[2]":string, "[3]":string, "[4]":string, "[5]":string, "[6]":string, "[7]":string, "[8]":string, "[8] 2":string, "[8] 3":string, "[8] 4":string}
  T8 = typedef "IMAQ Image.ctl" = refnum<image>
  T9 = cluster{"Area":dbl, "Number of Holes":dbl, "Bounding Rect":cluster{"Left":dbl, "Top":dbl, "Right":dbl, "Bottom":dbl}, "Center of Mass":cluster{"X":dbl, "Y":dbl}, "Orientation":dbl, "Dimensions":cluster{"Width":dbl, "Height":dbl}}[][]
  T10 = enum32{"System", "Detection", "Feedback", "Pico3", "Pico4"}
  T11 = cluster{"Ref X":refnum<vi>, "Ref Y":refnum<vi>}[]
  T12 = typedef "tcp_new_data_event.ctl" = refnum<user-event>
  T13 = typedef "tcp new data cluster.ctl" = cluster{"EventEnum":enum16{"new data", "connection status update"}, "Device name":string}
  T14 = cluster{"Left":i32, "Top":i32, "Right":i32, "Bottom":i32}
  T15 = enum32{"invalid app kind", "Development System", "Run Time System", "Student Edition", "Embedded LabVIEW", "Evaluation", "Custom"}
  T16 = enum16{"open", "open or create", "create or replace", "create", "open (read-only)"}
  T17 = enum32{"Invalid", "Standard", "Closed", "Hidden", "Minimized", "Maximized"}
  T18 = enum16{"open", "replace", "create", "open or create", "replace or create", "replace or create with confirmation"}
  T19 = typedef "Image Type" = u32
  T20 = cluster{"[0]":string, "[1]":string, "[2]":string, "[3]":string, "[4]":string, "[5]":string, "[6]":string, "[7]":string, "[8]":string, "[9]":string, "[10]":string, "[11]":string}
  T21 = cluster{"Target.X::1":refnum<vi>, "Target.Y::1":refnum<vi>}
  T22 = cluster{"Target.X::2":refnum<vi>, "Target.Y::2":refnum<vi>}
  T23 = cluster{"Target.X::3":refnum<vi>, "Target.Y::3":refnum<vi>}
  T24 = cluster{"Target.X::4":refnum<vi>, "Target.Y::4":refnum<vi>}
  T25 = cluster{"Target.X::5":refnum<vi>, "Target.Y::5":refnum<vi>}
  T26 = cluster{"Target.X::6":refnum<vi>, "Target.Y::6":refnum<vi>}
  T27 = cluster{"Target.X::7":refnum<vi>, "Target.Y::7":refnum<vi>}
  T28 = cluster{"Target.X::8":refnum<vi>, "Target.Y::8":refnum<vi>}
  T29 = cluster{"Target.X::12":refnum<vi>, "Target.Y::12":refnum<vi>}
  T30 = cluster{"Target.X::9":refnum<vi>, "Target.Y::9":refnum<vi>}
  T31 = cluster{"Target.X::10":refnum<vi>, "Target.Y::10":refnum<vi>}
  T32 = cluster{"Target.X::11":refnum<vi>, "Target.Y::11":refnum<vi>}
  T33 = cluster{"Target.X::12":refnum<vi>, "Target.Y::12":refnum<vi>}[]
  T34 = cluster{"Left":dbl, "Top":dbl, "Right":dbl, "Bottom":dbl}
  T35 = cluster{"Area":dbl, "Number of Holes":dbl, "Bounding Rect":cluster{"Left":dbl, "Top":dbl, "Right":dbl, "Bottom":dbl}, "Center of Mass":cluster{"X":dbl, "Y":dbl}, "Orientation":dbl, "Dimensions":cluster{"Width":dbl, "Height":dbl}}[]
  T36 = cluster{"Core":cluster{"Current VI Reference":refnum<vi>, "Close Panel on Exit?":bool}, "detection para":T2[], "thresholds":cluster{"Lower value":sgl, "Upper value":sgl}[], "Centroid X":dbl[][], "Centroid Y":dbl[][], "img to avg":i32, "Mean Centroid X":dbl[][], "Mean Centroid Y":dbl[][], "Offset X":dbl[][], "Offset Y":dbl[][], "Offset X stats ":dbl[][], "Offset Y stats ":dbl[][], "Size":dbl[][], "Mean Size":dbl[][], "Time":timestamp[][], "move properties":T1[], "active axis refs 2":cluster{"Ref X":refnum<vi>, "Ref Y":refnum<vi>}[], "active ccd":i32, "Feedback global":bool, "Motor X":dbl[][], "Motor Y":dbl[][], "active cams":string[], "tdms file out":refnum<k34>}
  T37 = cluster{"Current VI Reference":refnum<vi>, "Close Panel on Exit?":bool}
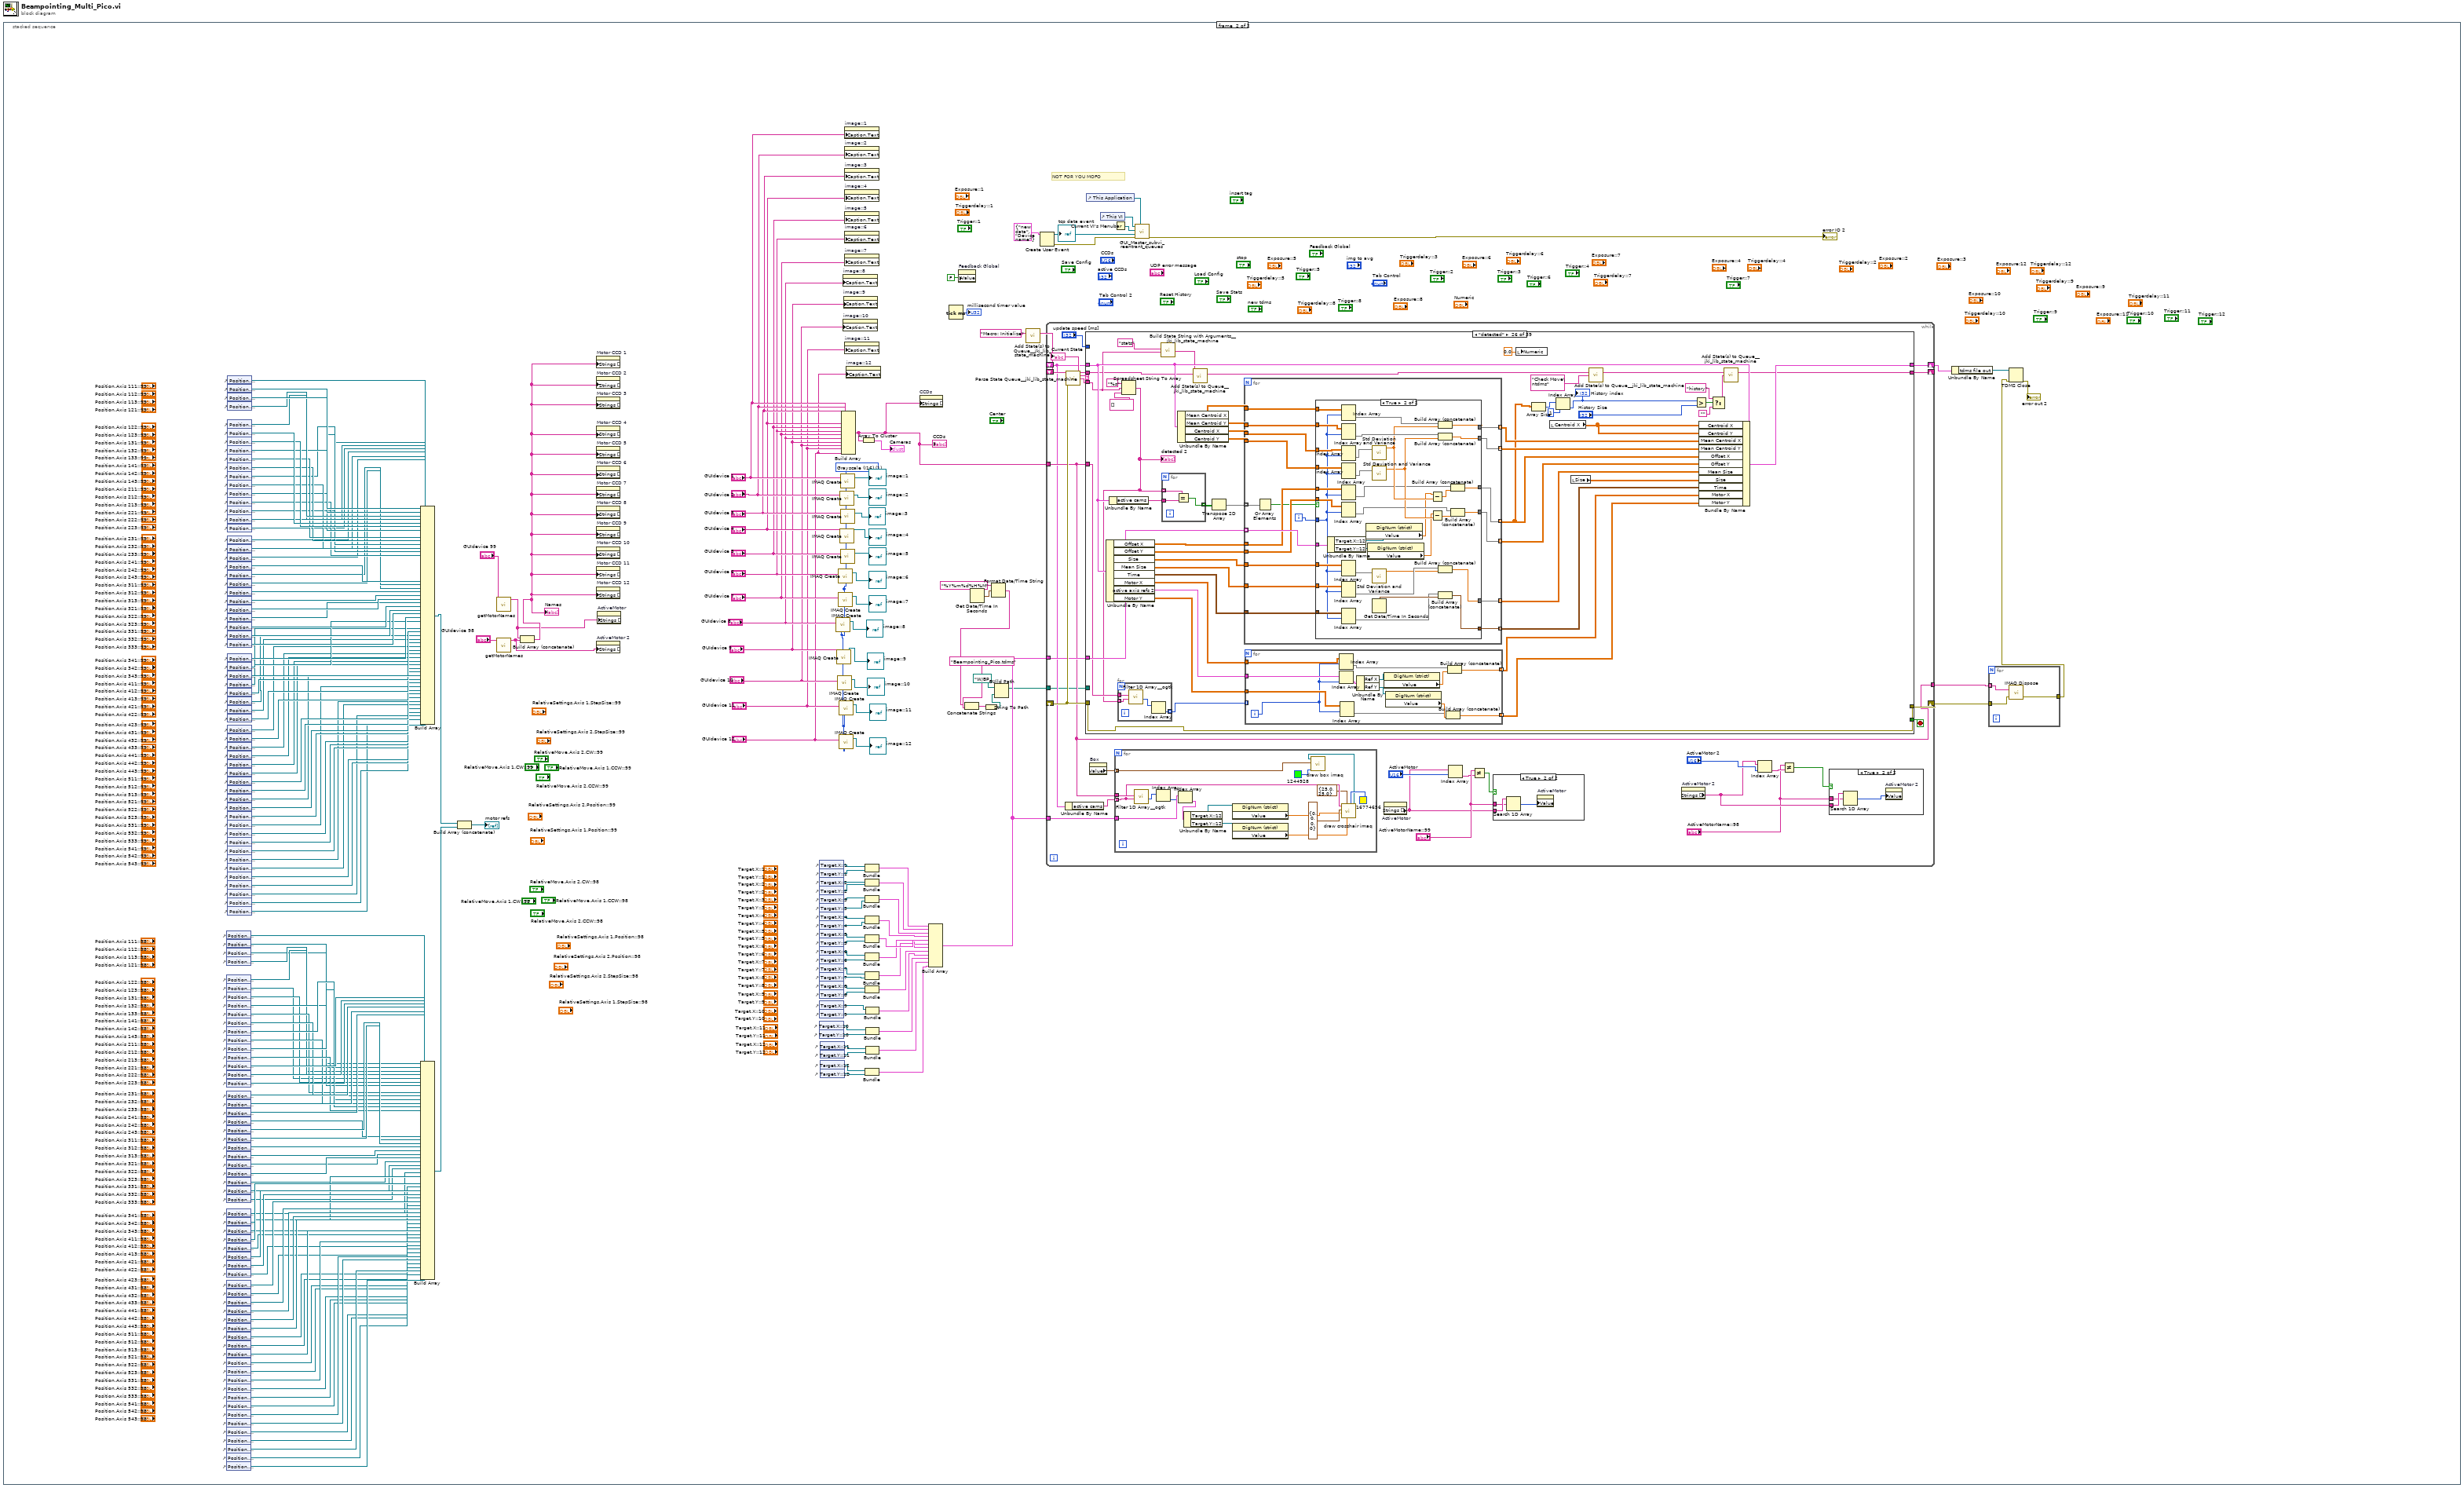
[diagram p0: block diagram]
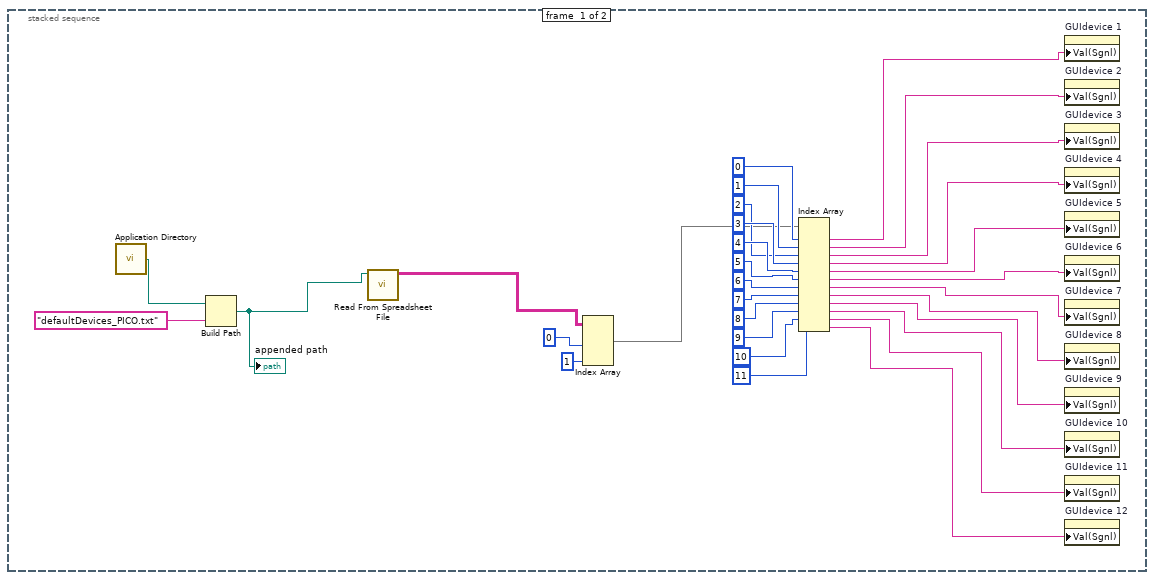
[diagram p2: hidden frame]
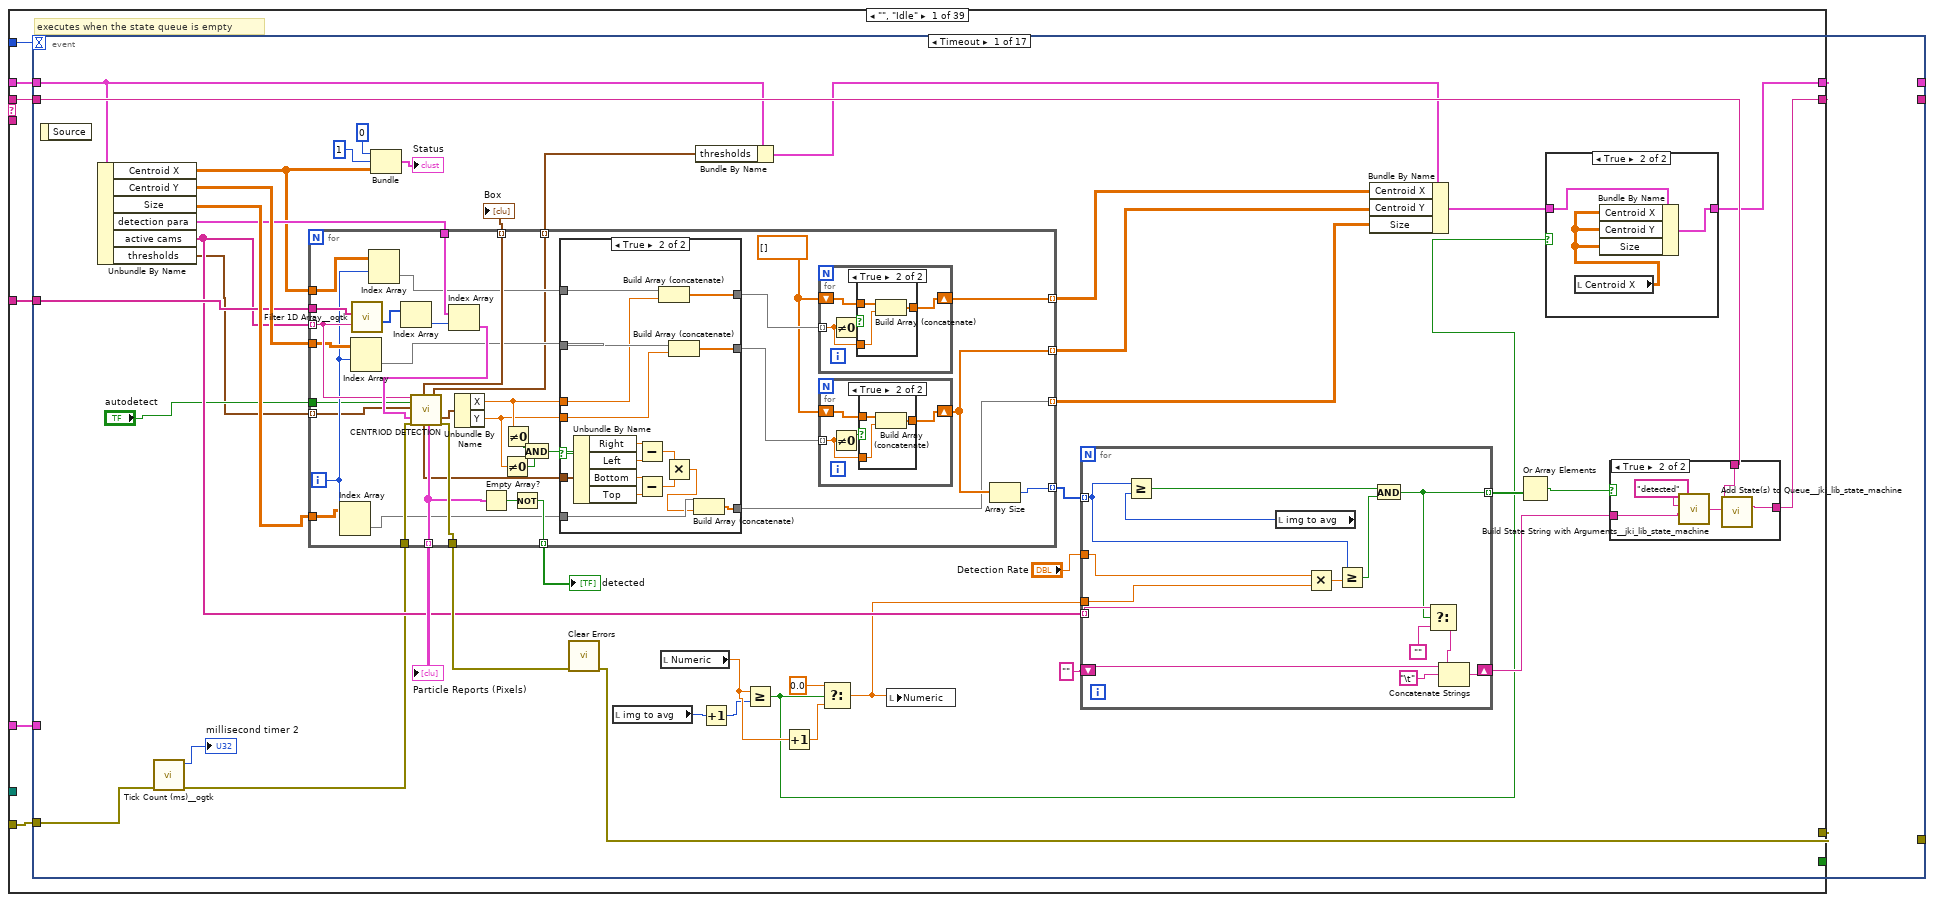
[diagram p5: hidden frame]
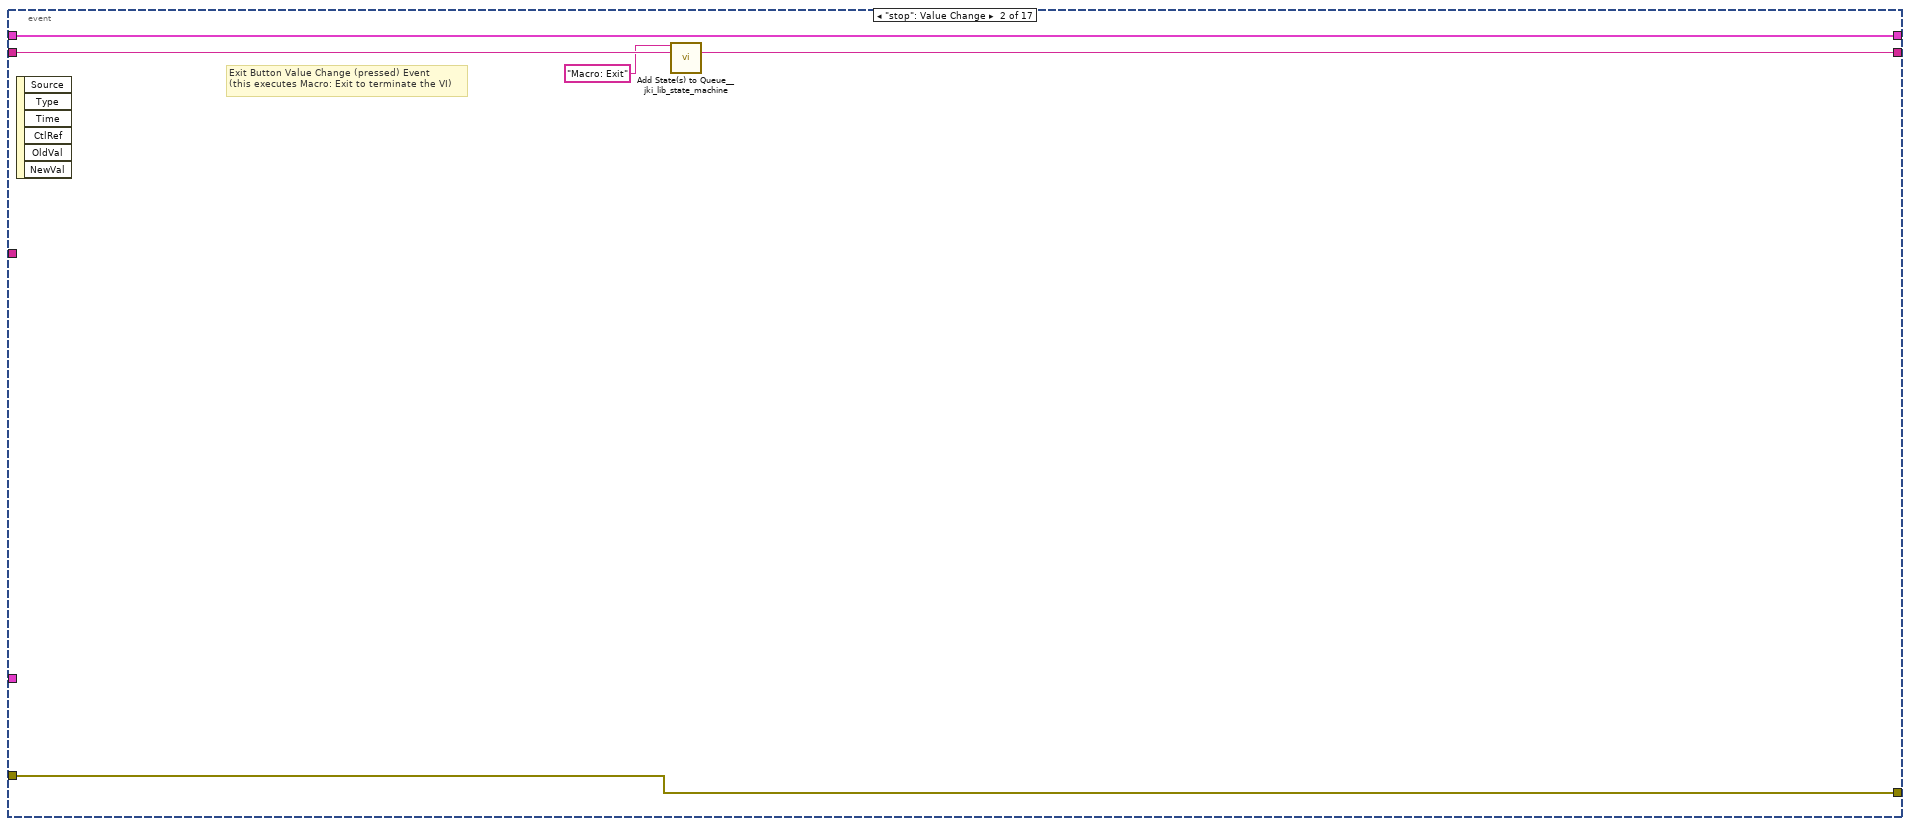
[diagram p11: hidden frame]
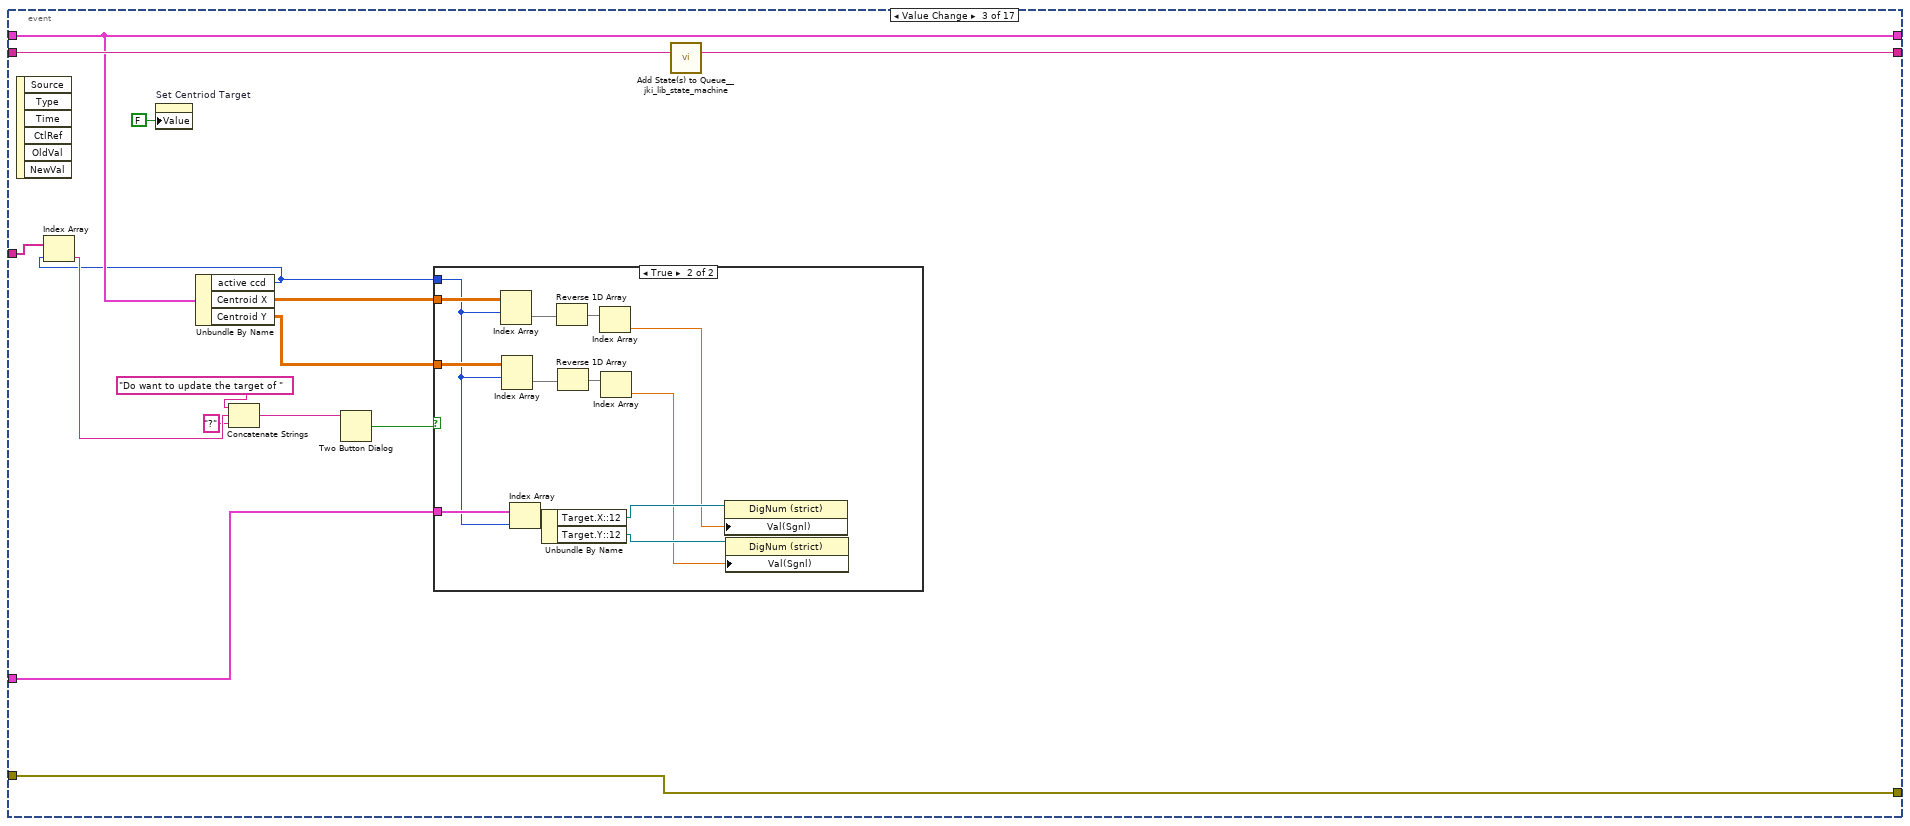
[diagram p12: hidden frame]
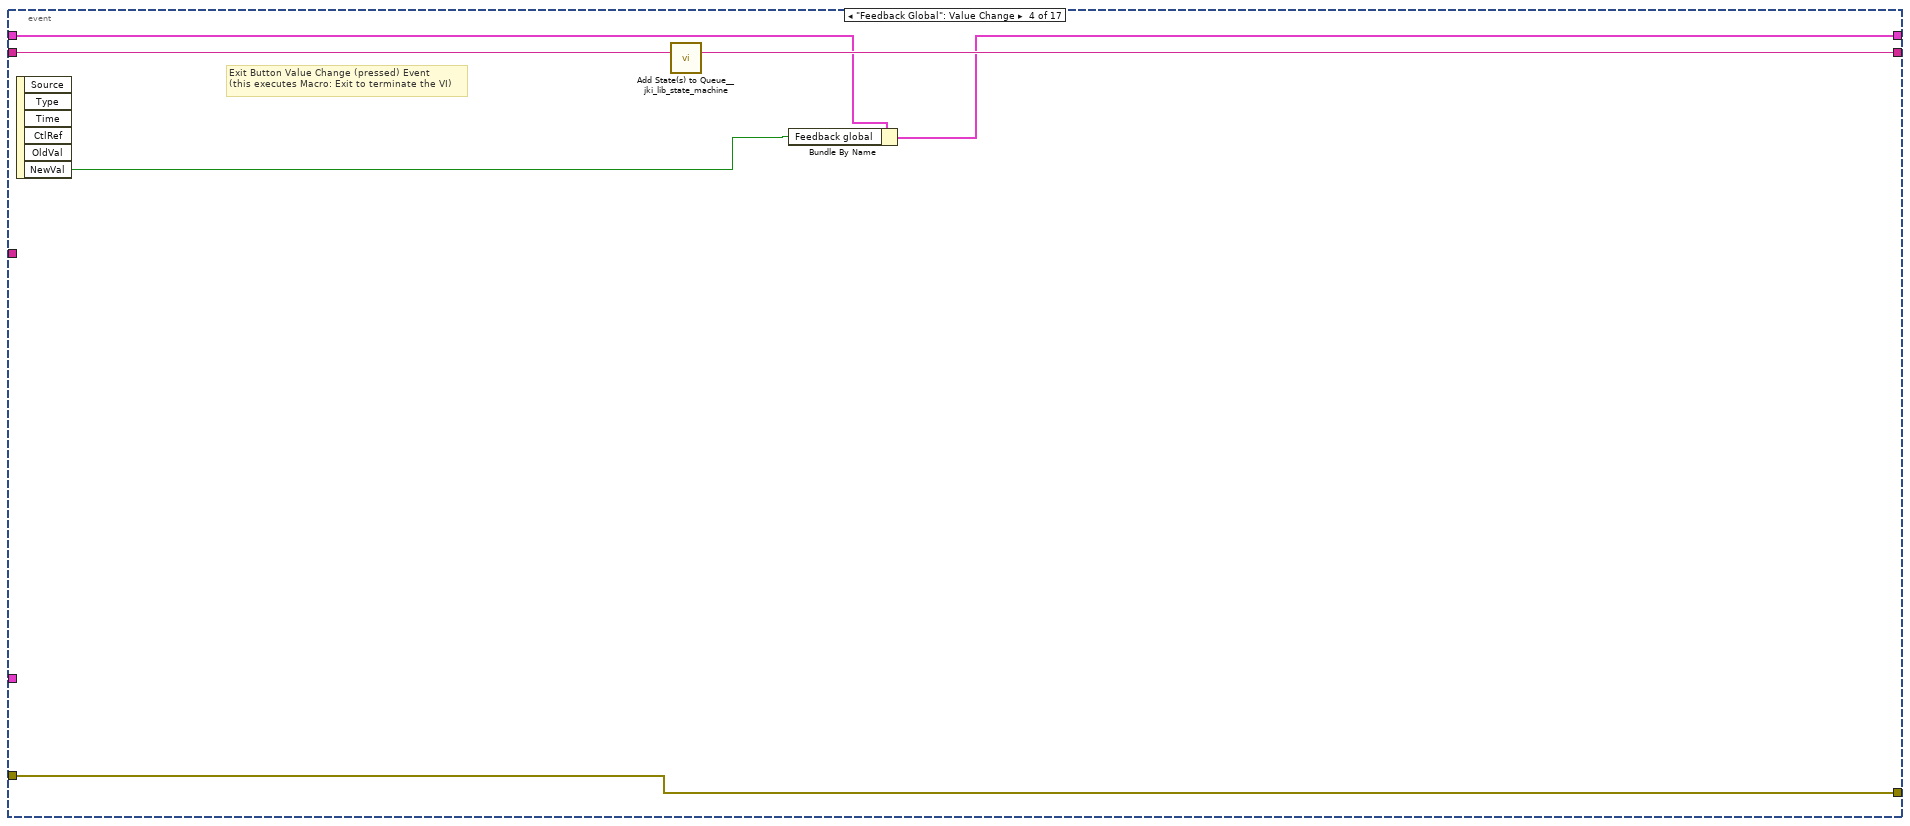
[diagram p14: hidden frame]
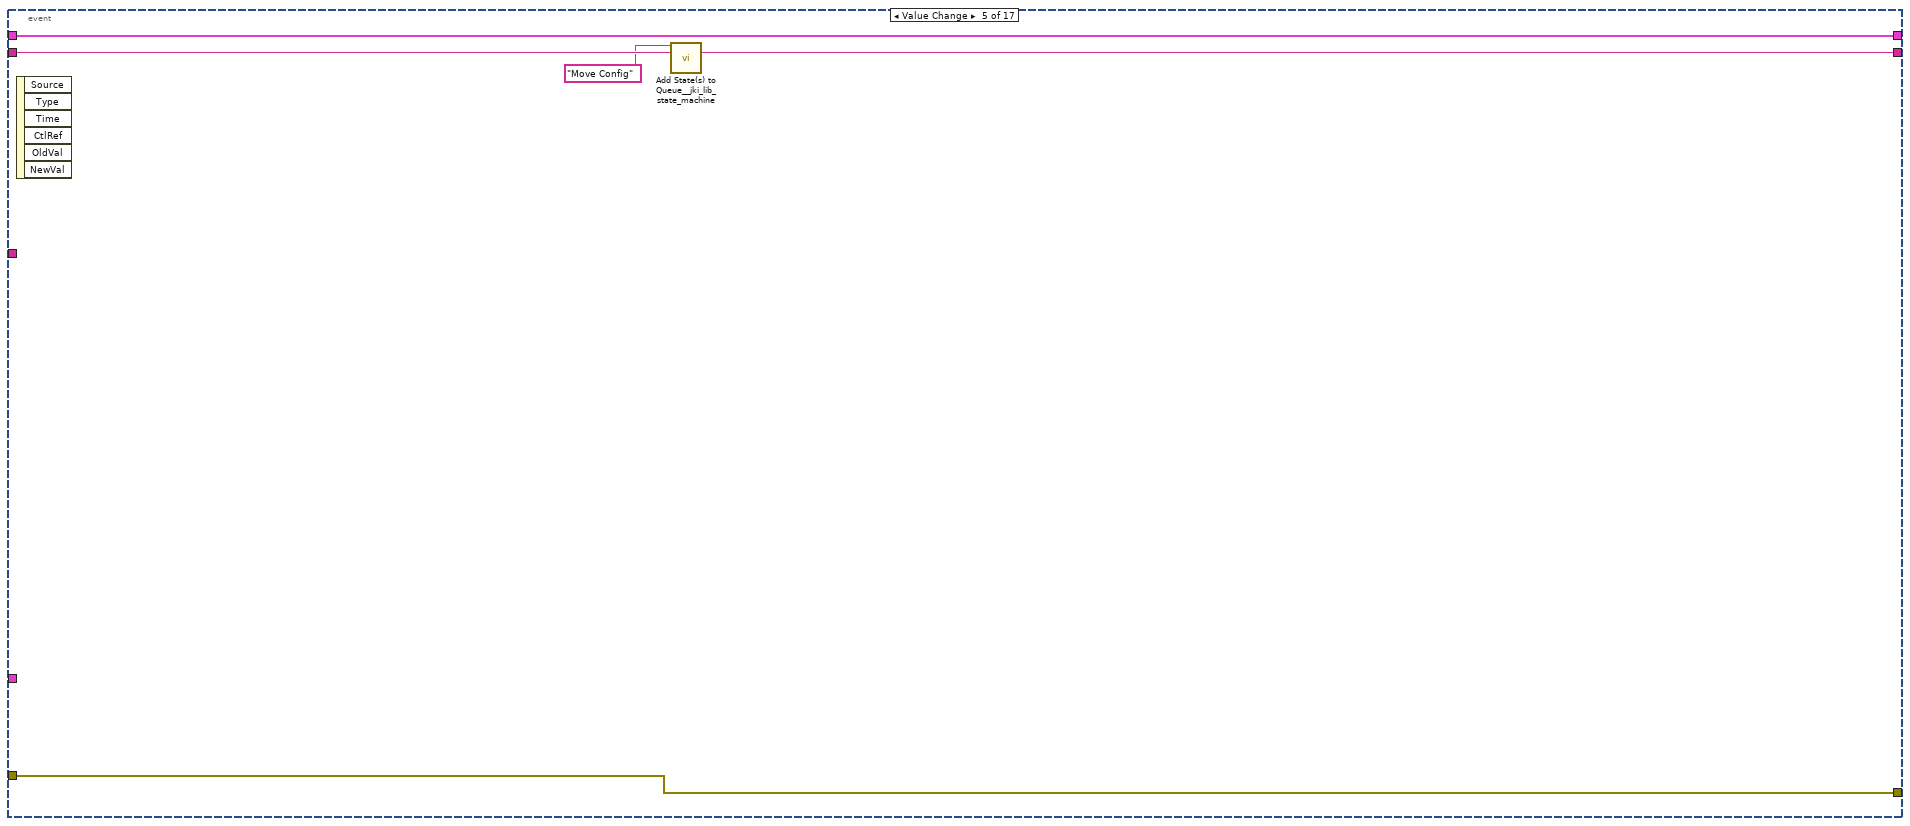
[diagram p15: hidden frame]
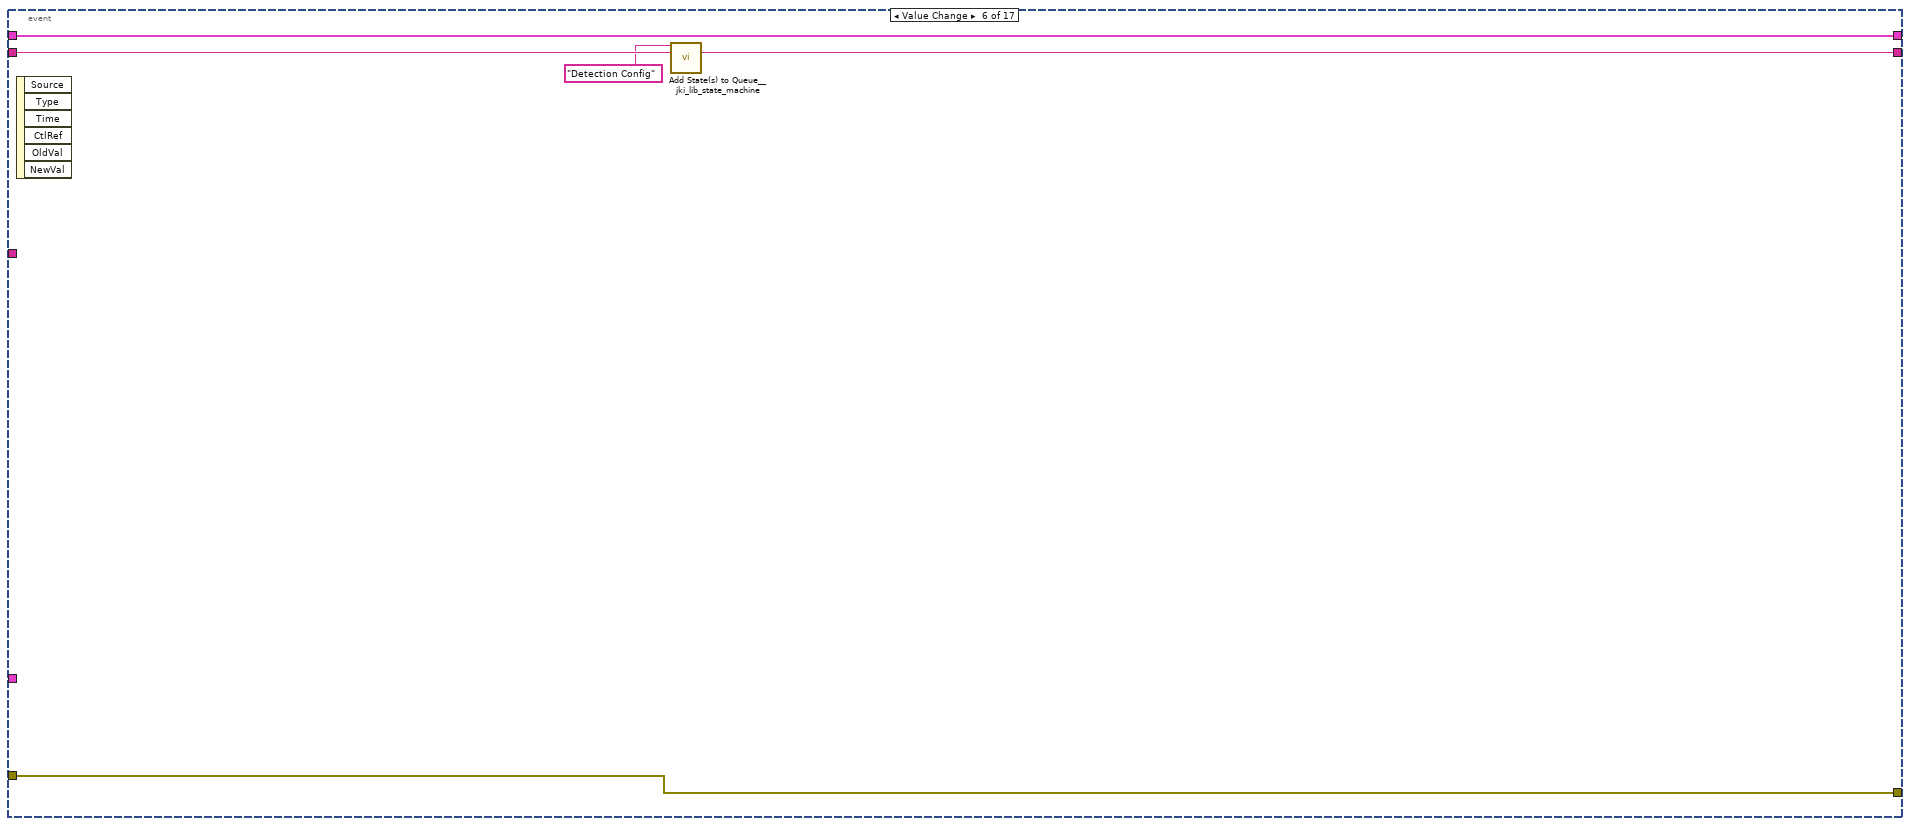
[diagram p16: hidden frame]
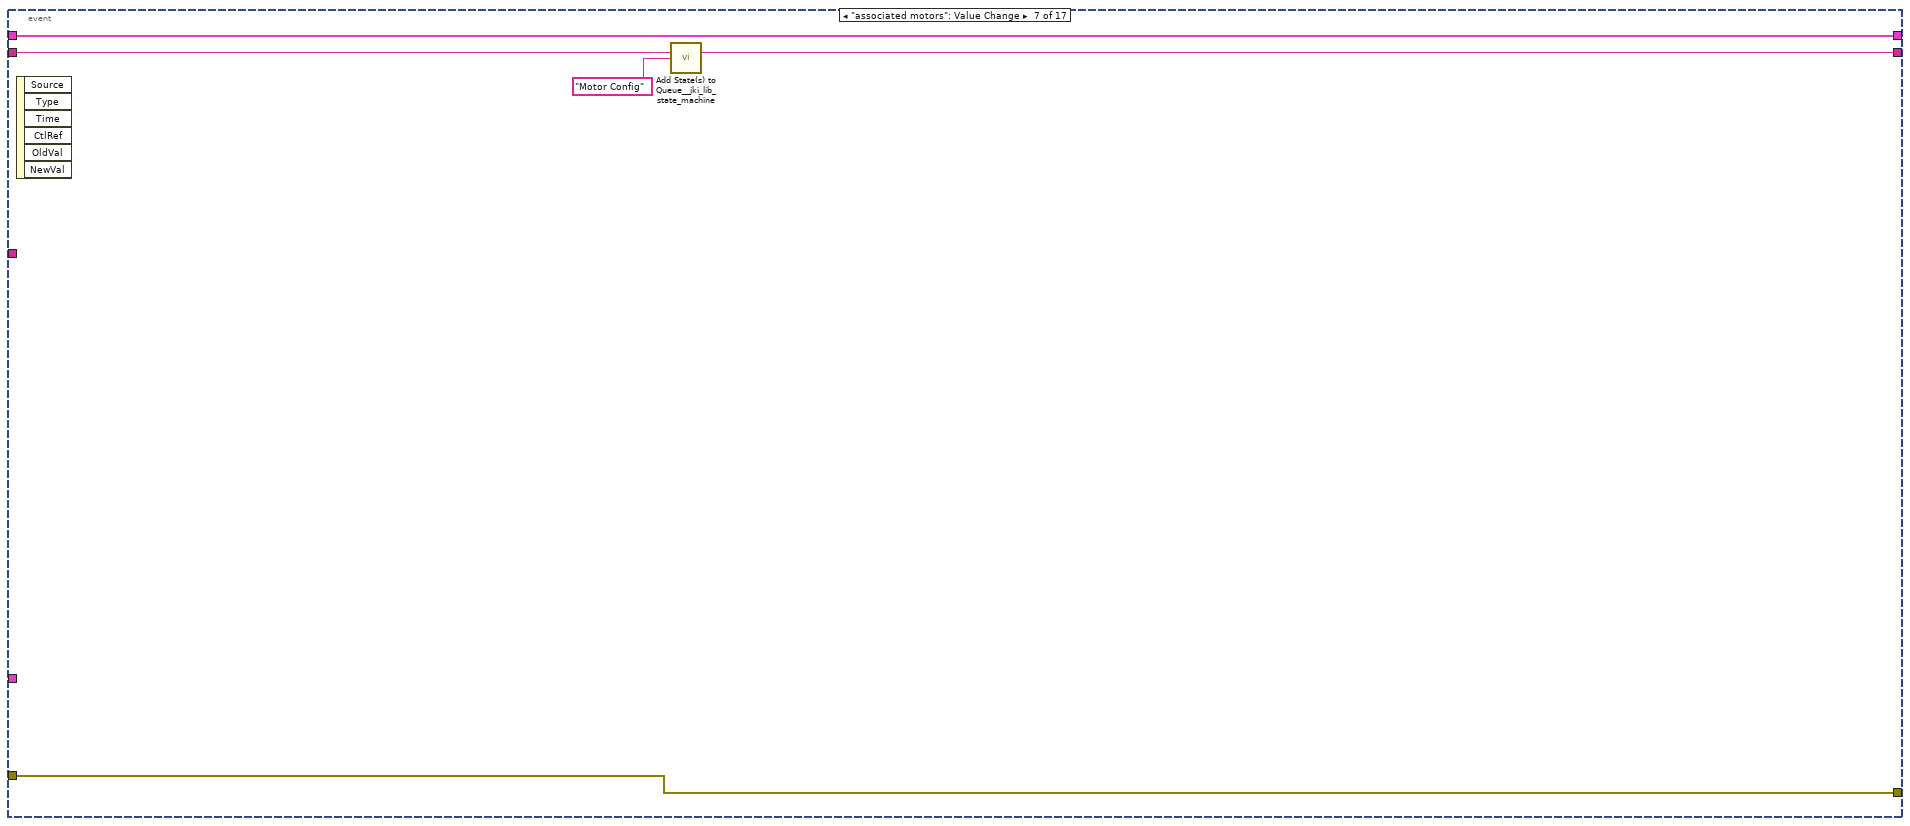
[diagram p17: hidden frame]
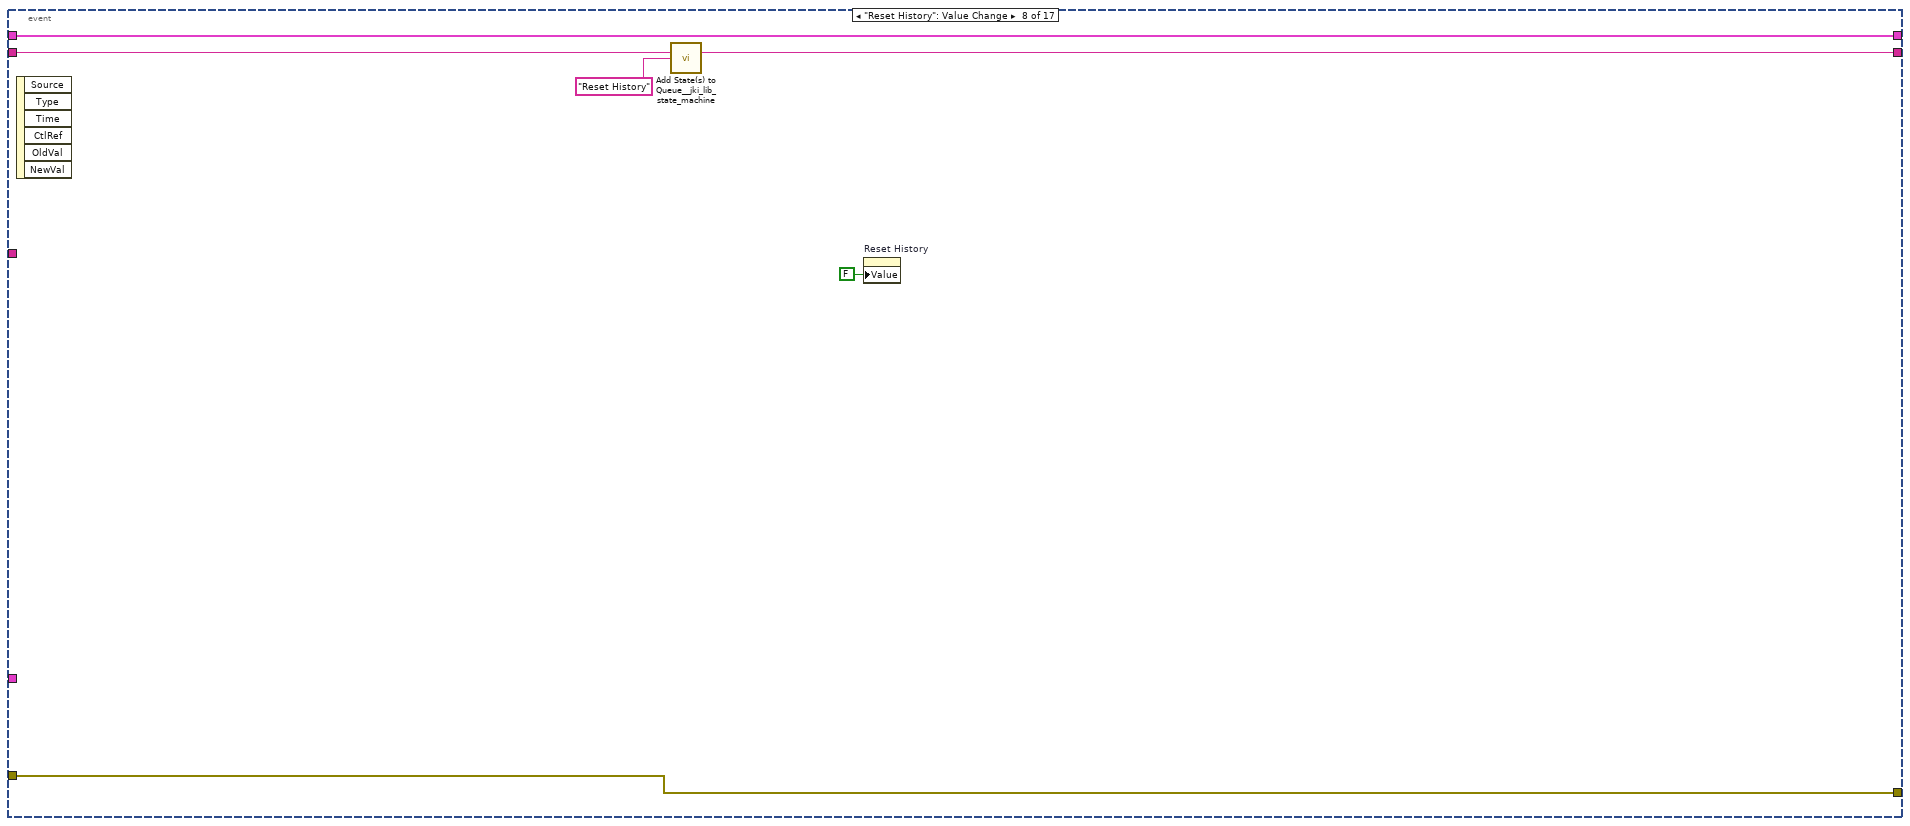
[diagram p18: hidden frame]
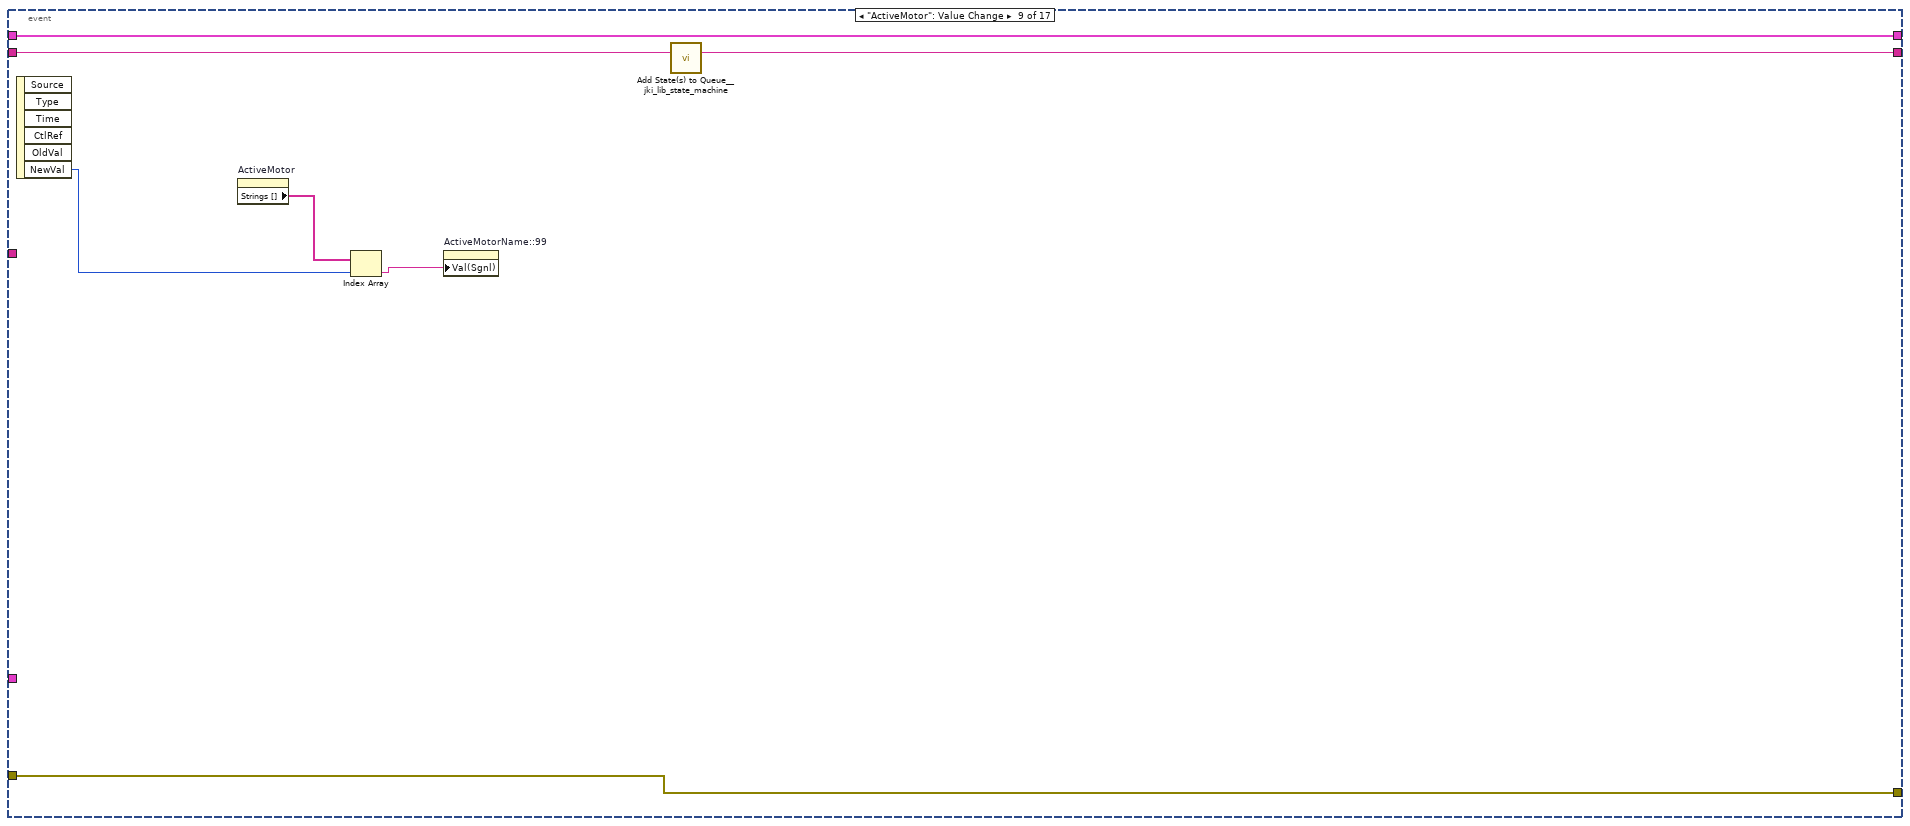
[diagram p19: hidden frame]
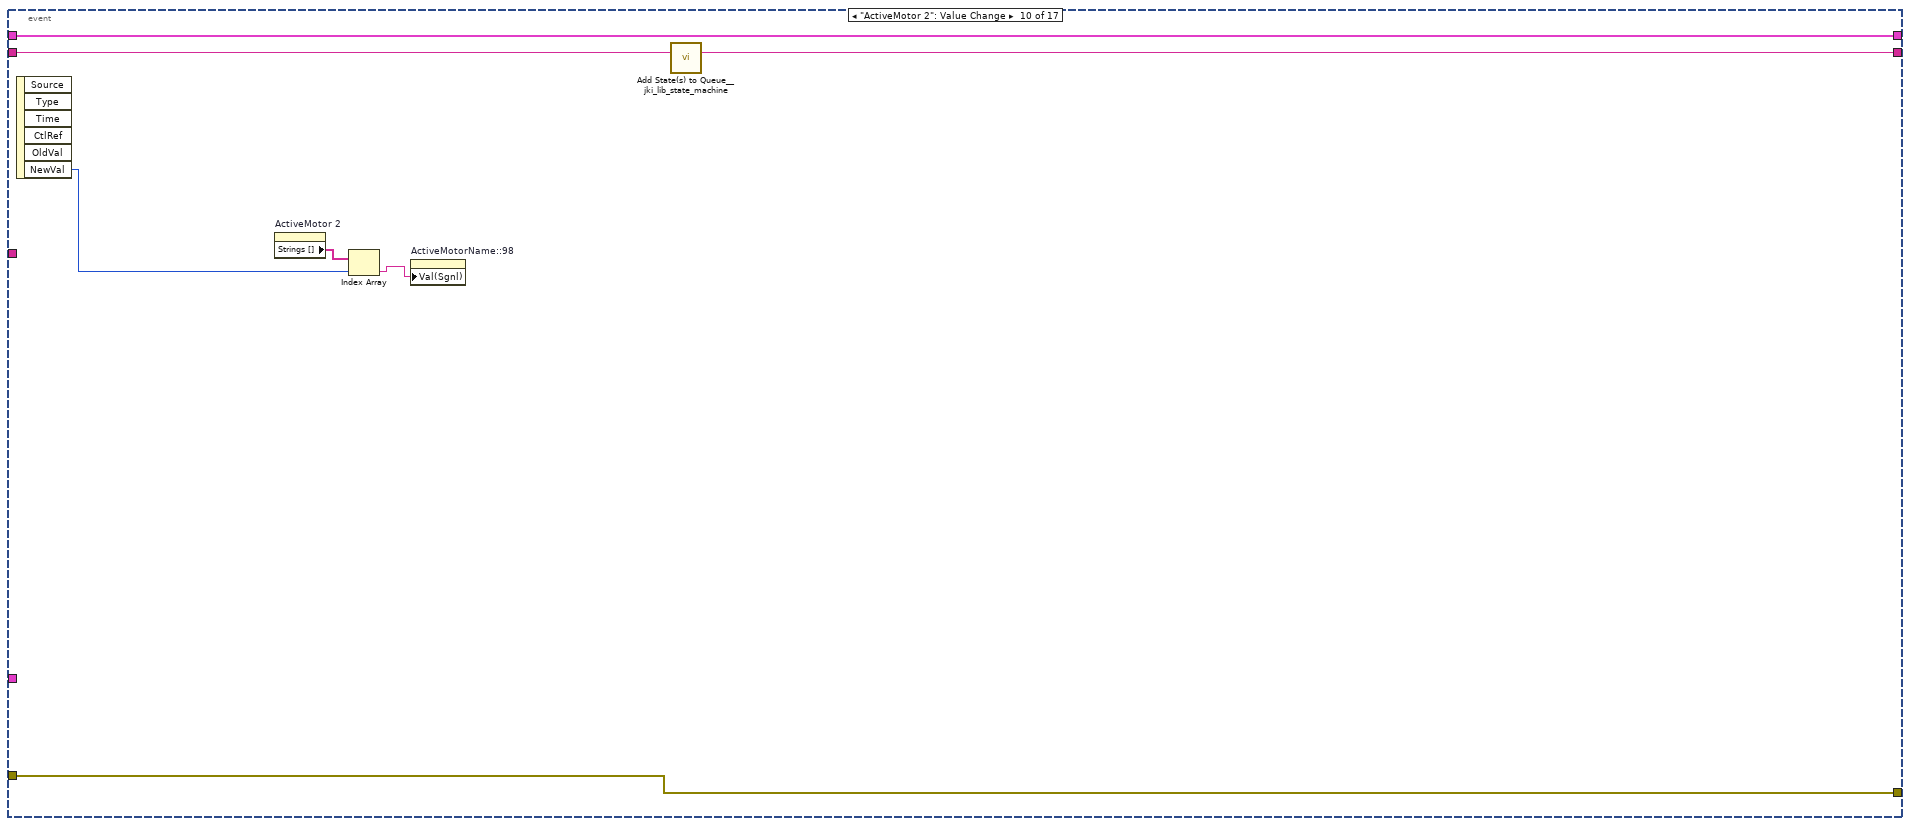
[diagram p20: hidden frame]
diagram:
  n1 = stacked-sequence {
    frame #0 {
      n2 = call <vilib>:"Application Directory.vi"() -> ("Application Directory"=w13:path)
      n3 = Build Path(base path=w13, name or relative path="defaultDevices_PICO.txt") -> (appended path=w15:path)
      "appended path" <- w15
      n4 = call-poly <vilib>:"Read From Spreadsheet File.vi"("file path (dialog if empty)"=w15) -> ("all rows"=w16:string[][])  [unwired: 6 in, 4 out]
      n5 = Index Array(array=w16, index (col) #1=0 ("disabled index (col)"), index (col) #2=1 ("index (col)")) -> (element #1=w19:string[])  [unwired: 2 in, 1 out]
      n6 = Index Array(array=w19, index #1=0 ("index"), index #2=1 ("index"), index #3=2 ("index"), index #4=3 ("index"), index #5=4 ("index"), index #6=5 ("index"), index #7=6 ("index"), index #8=7 ("index"), index #9=8 ("index"), index #10=9 ("index"), index #11=10 ("index"), index #12=11 ("index")) -> (element #1=w12:string, element #2=w11:string, element #3=w10:string, element #4=w9:string, element #5=w8:string, element #6=w7:string, element #7=w6:string, element #8=w5:string, element #9=w4:string, element #10=w3:string, element #11=w2:string, element #12=w1:string)
      n7 = property on="GUIdevice 1" class="Str"("Val(Sgnl)"=w12) -> ()  [unwired: 2 in, 2 out]
      n8 = property on="GUIdevice 2" class="Str"("Val(Sgnl)"=w11) -> ()  [unwired: 2 in, 2 out]
      n9 = property on="GUIdevice 3" class="Str"("Val(Sgnl)"=w10) -> ()  [unwired: 2 in, 2 out]
      n10 = property on="GUIdevice 4" class="Str"("Val(Sgnl)"=w9) -> ()  [unwired: 2 in, 2 out]
      n11 = property on="GUIdevice 5" class="Str"("Val(Sgnl)"=w8) -> ()  [unwired: 2 in, 2 out]
      n12 = property on="GUIdevice 6" class="Str"("Val(Sgnl)"=w7) -> ()  [unwired: 2 in, 2 out]
      n13 = property on="GUIdevice 7" class="Str"("Val(Sgnl)"=w6) -> ()  [unwired: 2 in, 2 out]
      n14 = property on="GUIdevice 8" class="Str"("Val(Sgnl)"=w5) -> ()  [unwired: 2 in, 2 out]
      n15 = property on="GUIdevice 9" class="Str"("Val(Sgnl)"=w4) -> ()  [unwired: 2 in, 2 out]
      n16 = property on="GUIdevice 10" class="Str"("Val(Sgnl)"=w3) -> ()  [unwired: 2 in, 2 out]
      n17 = property on="GUIdevice 11" class="Str"("Val(Sgnl)"=w2) -> ()  [unwired: 2 in, 2 out]
      n18 = property on="GUIdevice 12" class="Str"("Val(Sgnl)"=w1) -> ()  [unwired: 2 in, 2 out]
    }
    frame #1 {
      w104 = T19 1 items=["Grayscale (U8)", "Grayscale (I16)", "Grayscale (SGL)", "Complex (CSG)", "RGB (U32)", "HSL (U32)", "RGB (U64)", "Grayscale (U16)"] ("Image Type")
      # "NOT FOR YOU MOFO"
      n19 = control-ref of="Position.Axis 111::98"() -> (w41:refnum<vi>)
      n20 = control-ref of="Position.Axis 112::98"() -> (w42:refnum<vi>)
      n21 = control-ref of="Position.Axis 113::98"() -> (w43:refnum<vi>)
      n22 = control-ref of="Position.Axis 121::98"() -> (w44:refnum<vi>)
      n23 = control-ref of="Position.Axis 122::98"() -> (w45:refnum<vi>)
      n24 = control-ref of="Position.Axis 123::98"() -> (w46:refnum<vi>)
      n25 = control-ref of="Position.Axis 131::98"() -> (w47:refnum<vi>)
      n26 = control-ref of="Position.Axis 132::98"() -> (w48:refnum<vi>)
      n27 = control-ref of="Position.Axis 133::98"() -> (w49:refnum<vi>)
      n28 = control-ref of="Position.Axis 141::98"() -> (w50:refnum<vi>)
      n29 = control-ref of="Position.Axis 142::98"() -> (w51:refnum<vi>)
      n30 = control-ref of="Position.Axis 143::98"() -> (w52:refnum<vi>)
      n31 = control-ref of="Position.Axis 211::98"() -> (w53:refnum<vi>)
      n32 = control-ref of="Position.Axis 212::98"() -> (w54:refnum<vi>)
      n33 = control-ref of="Position.Axis 213::98"() -> (w55:refnum<vi>)
      n34 = control-ref of="Position.Axis 221::98"() -> (w56:refnum<vi>)
      n35 = control-ref of="Position.Axis 222::98"() -> (w57:refnum<vi>)
      n36 = control-ref of="Position.Axis 223::98"() -> (w58:refnum<vi>)
      n37 = control-ref of="Position.Axis 231::98"() -> (w59:refnum<vi>)
      n38 = control-ref of="Position.Axis 232::98"() -> (w60:refnum<vi>)
      n39 = control-ref of="Position.Axis 233::98"() -> (w61:refnum<vi>)
      n40 = control-ref of="Position.Axis 241::98"() -> (w62:refnum<vi>)
      n41 = control-ref of="Position.Axis 242::98"() -> (w63:refnum<vi>)
      n42 = control-ref of="Position.Axis 243::98"() -> (w64:refnum<vi>)
      n43 = control-ref of="Position.Axis 311::98"() -> (w65:refnum<vi>)
      n44 = control-ref of="Position.Axis 312::98"() -> (w66:refnum<vi>)
      n45 = control-ref of="Position.Axis 313::98"() -> (w67:refnum<vi>)
      n46 = control-ref of="Position.Axis 321::98"() -> (w68:refnum<vi>)
      n47 = control-ref of="Position.Axis 322::98"() -> (w69:refnum<vi>)
      n48 = control-ref of="Position.Axis 323::98"() -> (w70:refnum<vi>)
      n49 = control-ref of="Position.Axis 331::98"() -> (w71:refnum<vi>)
      n50 = control-ref of="Position.Axis 332::98"() -> (w72:refnum<vi>)
      n51 = control-ref of="Position.Axis 333::98"() -> (w73:refnum<vi>)
      n52 = control-ref of="Position.Axis 341::98"() -> (w74:refnum<vi>)
      n53 = control-ref of="Position.Axis 342::98"() -> (w75:refnum<vi>)
      n54 = control-ref of="Position.Axis 343::98"() -> (w76:refnum<vi>)
      n55 = control-ref of="Position.Axis 411::98"() -> (w77:refnum<vi>)
      n56 = control-ref of="Position.Axis 412::98"() -> (w78:refnum<vi>)
      n57 = control-ref of="Position.Axis 413::98"() -> (w79:refnum<vi>)
      n58 = control-ref of="Position.Axis 421::98"() -> (w80:refnum<vi>)
      n59 = control-ref of="Position.Axis 422::98"() -> (w81:refnum<vi>)
      n60 = control-ref of="Position.Axis 423::98"() -> (w82:refnum<vi>)
      n61 = control-ref of="Position.Axis 431::98"() -> (w83:refnum<vi>)
      n62 = control-ref of="Position.Axis 432::98"() -> (w84:refnum<vi>)
      n63 = control-ref of="Position.Axis 433::98"() -> (w85:refnum<vi>)
      n64 = control-ref of="Position.Axis 441::98"() -> (w86:refnum<vi>)
      n65 = control-ref of="Position.Axis 442::98"() -> (w87:refnum<vi>)
      n66 = control-ref of="Position.Axis 443::98"() -> (w88:refnum<vi>)
      n67 = control-ref of="Position.Axis 511::98"() -> (w89:refnum<vi>)
      n68 = control-ref of="Position.Axis 512::98"() -> (w90:refnum<vi>)
      n69 = control-ref of="Position.Axis 513::98"() -> (w91:refnum<vi>)
      n70 = control-ref of="Position.Axis 521::98"() -> (w92:refnum<vi>)
      n71 = control-ref of="Position.Axis 522::98"() -> (w93:refnum<vi>)
      n72 = control-ref of="Position.Axis 523::98"() -> (w94:refnum<vi>)
      n73 = control-ref of="Position.Axis 531::98"() -> (w95:refnum<vi>)
      n74 = control-ref of="Position.Axis 532::98"() -> (w96:refnum<vi>)
      n75 = control-ref of="Position.Axis 533::98"() -> (w97:refnum<vi>)
      n76 = control-ref of="Position.Axis 541::98"() -> (w98:refnum<vi>)
      n77 = control-ref of="Position.Axis 542::98"() -> (w99:refnum<vi>)
      n78 = control-ref of="Position.Axis 543::98"() -> (w100:refnum<vi>)
      n79 = control-ref of="Position.Axis 111::99"() -> (w232:refnum<vi>)
      n80 = control-ref of="Position.Axis 112::99"() -> (w231:refnum<vi>)
      n81 = control-ref of="Position.Axis 113::99"() -> (w230:refnum<vi>)
      n82 = control-ref of="Position.Axis 121::99"() -> (w229:refnum<vi>)
      n83 = control-ref of="Position.Axis 122::99"() -> (w228:refnum<vi>)
      n84 = control-ref of="Position.Axis 123::99"() -> (w227:refnum<vi>)
      n85 = control-ref of="Position.Axis 131::99"() -> (w226:refnum<vi>)
      n86 = control-ref of="Position.Axis 132::99"() -> (w225:refnum<vi>)
      n87 = control-ref of="Position.Axis 133::99"() -> (w224:refnum<vi>)
      n88 = control-ref of="Position.Axis 141::99"() -> (w223:refnum<vi>)
      n89 = control-ref of="Position.Axis 142::99"() -> (w222:refnum<vi>)
      n90 = control-ref of="Position.Axis 143::99"() -> (w221:refnum<vi>)
      n91 = control-ref of="Position.Axis 211::99"() -> (w220:refnum<vi>)
      n92 = control-ref of="Position.Axis 212::99"() -> (w219:refnum<vi>)
      n93 = control-ref of="Position.Axis 213::99"() -> (w218:refnum<vi>)
      n94 = control-ref of="Position.Axis 221::99"() -> (w217:refnum<vi>)
      n95 = control-ref of="Position.Axis 222::99"() -> (w216:refnum<vi>)
      n96 = control-ref of="Position.Axis 223::99"() -> (w215:refnum<vi>)
      n97 = control-ref of="Position.Axis 231::99"() -> (w214:refnum<vi>)
      n98 = control-ref of="Position.Axis 232::99"() -> (w213:refnum<vi>)
      n99 = control-ref of="Position.Axis 233::99"() -> (w212:refnum<vi>)
      n100 = control-ref of="Position.Axis 241::99"() -> (w211:refnum<vi>)
      n101 = control-ref of="Position.Axis 242::99"() -> (w210:refnum<vi>)
      n102 = control-ref of="Position.Axis 243::99"() -> (w209:refnum<vi>)
      n103 = control-ref of="Position.Axis 311::99"() -> (w208:refnum<vi>)
      n104 = control-ref of="Position.Axis 312::99"() -> (w207:refnum<vi>)
      n105 = control-ref of="Position.Axis 313::99"() -> (w206:refnum<vi>)
      n106 = control-ref of="Position.Axis 321::99"() -> (w205:refnum<vi>)
      n107 = control-ref of="Position.Axis 322::99"() -> (w204:refnum<vi>)
      n108 = control-ref of="Position.Axis 323::99"() -> (w203:refnum<vi>)
      n109 = control-ref of="Position.Axis 331::99"() -> (w202:refnum<vi>)
      n110 = control-ref of="Position.Axis 332::99"() -> (w201:refnum<vi>)
      n111 = control-ref of="Position.Axis 333::99"() -> (w200:refnum<vi>)
      n112 = control-ref of="Position.Axis 341::99"() -> (w199:refnum<vi>)
      n113 = control-ref of="Position.Axis 342::99"() -> (w198:refnum<vi>)
      n114 = control-ref of="Position.Axis 343::99"() -> (w197:refnum<vi>)
      n115 = control-ref of="Position.Axis 411::99"() -> (w196:refnum<vi>)
      n116 = control-ref of="Position.Axis 412::99"() -> (w195:refnum<vi>)
      n117 = control-ref of="Position.Axis 413::99"() -> (w194:refnum<vi>)
      n118 = control-ref of="Position.Axis 421::99"() -> (w193:refnum<vi>)
      n119 = control-ref of="Position.Axis 422::99"() -> (w192:refnum<vi>)
      n120 = control-ref of="Position.Axis 423::99"() -> (w191:refnum<vi>)
      n121 = control-ref of="Position.Axis 431::99"() -> (w190:refnum<vi>)
      n122 = control-ref of="Position.Axis 432::99"() -> (w189:refnum<vi>)
      n123 = control-ref of="Position.Axis 433::99"() -> (w188:refnum<vi>)
      n124 = control-ref of="Position.Axis 441::99"() -> (w187:refnum<vi>)
      n125 = control-ref of="Position.Axis 442::99"() -> (w186:refnum<vi>)
      n126 = control-ref of="Position.Axis 443::99"() -> (w185:refnum<vi>)
      n127 = control-ref of="Position.Axis 511::99"() -> (w184:refnum<vi>)
      n128 = control-ref of="Position.Axis 512::99"() -> (w183:refnum<vi>)
      n129 = control-ref of="Position.Axis 513::99"() -> (w182:refnum<vi>)
      n130 = control-ref of="Position.Axis 521::99"() -> (w181:refnum<vi>)
      n131 = control-ref of="Position.Axis 522::99"() -> (w180:refnum<vi>)
      n132 = control-ref of="Position.Axis 523::99"() -> (w179:refnum<vi>)
      n133 = control-ref of="Position.Axis 531::99"() -> (w178:refnum<vi>)
      n134 = control-ref of="Position.Axis 532::99"() -> (w177:refnum<vi>)
      n135 = control-ref of="Position.Axis 533::99"() -> (w176:refnum<vi>)
      n136 = control-ref of="Position.Axis 541::99"() -> (w175:refnum<vi>)
      n137 = control-ref of="Position.Axis 542::99"() -> (w174:refnum<vi>)
      n138 = control-ref of="Position.Axis 543::99"() -> (w173:refnum<vi>)
      n139 = Build Array(w41, w42, w43, w44, w45, w46, w47, w48, w49, w50, w51, w52, w53, w54, w55, w56, w57, w58, w59, w60, w61, w62, w63, w64, w65, w66, w67, w68, w69, w70, w71, w72, w73, w74, w75, w76, w77, w78, w79, w80, w81, w82, w83, w84, w85, w86, w87, w88, w89, w90, w91, w92, w93, w94, w95, w96, w97, w98, w99, w100) -> (w38:refnum<vi>[])
      n140 = Build Array(w232, w231, w230, w229, w228, w227, w226, w225, w224, w223, w222, w221, w220, w219, w218, w217, w216, w215, w214, w213, w212, w211, w210, w209, w208, w207, w206, w205, w204, w203, w202, w201, w200, w199, w198, w197, w196, w195, w194, w193, w192, w191, w190, w189, w188, w187, w186, w185, w184, w183, w182, w181, w180, w179, w178, w177, w176, w175, w174, w173) -> (w37:refnum<vi>[])
      n141 = Build Array (concatenate)(w37, w38) -> (→"motor refs":refnum<vi>[])
      n142 = call "getMotorNames.vi"("DeviceName"="GUIdevice 99") -> ("elements"=w35:string[])  [unwired: 10 in]
      n143 = call "getMotorNames.vi"("DeviceName"="GUIdevice 98") -> ("elements"=w34:string[])  [unwired: 10 in]
      n144 = Build Array (concatenate)(w35, w34) -> (w39:string[])
      "Names" <- w39
      n145 = property on="Motor CCD 1" class="Ring (strict)"("Strings []"=w39) -> ()  [unwired: 2 in, 2 out]
      n146 = property on="Motor CCD 2" class="Ring (strict)"("Strings []"=w39) -> ()  [unwired: 2 in, 2 out]
      n147 = property on="Motor CCD 3" class="Ring (strict)"("Strings []"=w39) -> ()  [unwired: 2 in, 2 out]
      n148 = property on="Motor CCD 4" class="Ring (strict)"("Strings []"=w39) -> ()  [unwired: 2 in, 2 out]
      n149 = property on="Motor CCD 5" class="Ring (strict)"("Strings []"=w39) -> ()  [unwired: 2 in, 2 out]
      n150 = property on="Motor CCD 6" class="Ring (strict)"("Strings []"=w39) -> ()  [unwired: 2 in, 2 out]
      n151 = property on="Motor CCD 7" class="Ring (strict)"("Strings []"=w39) -> ()  [unwired: 2 in, 2 out]
      n152 = property on="Motor CCD 8" class="Ring (strict)"("Strings []"=w39) -> ()  [unwired: 2 in, 2 out]
      n153 = property on="Motor CCD 9" class="Ring (strict)"("Strings []"=w39) -> ()  [unwired: 2 in, 2 out]
      n154 = property on="Motor CCD 10" class="Ring (strict)"("Strings []"=w39) -> ()  [unwired: 2 in, 2 out]
      n155 = property on="Motor CCD 11" class="Ring (strict)"("Strings []"=w39) -> ()  [unwired: 2 in, 2 out]
      n156 = property on="Motor CCD 12" class="Ring (strict)"("Strings []"=w39) -> ()  [unwired: 2 in, 2 out]
      n157 = property on="ActiveMotor 2" class="Ring (strict)"("Strings []"=w34) -> ()  [unwired: 2 in, 2 out]
      n158 = property on="ActiveMotor" class="Ring (strict)"("Strings []"=w35) -> ()  [unwired: 2 in, 2 out]
      n159 = control-ref of="Target.X::1"() -> (w159:refnum<vi>)
      n160 = control-ref of="Target.Y::1"() -> (w158:refnum<vi>)
      n161 = control-ref of="Target.X::2"() -> (w157:refnum<vi>)
      n162 = control-ref of="Target.Y::2"() -> (w156:refnum<vi>)
      n163 = control-ref of="Target.X::3"() -> (w155:refnum<vi>)
      n164 = control-ref of="Target.Y::3"() -> (w154:refnum<vi>)
      n165 = control-ref of="Target.X::4"() -> (w153:refnum<vi>)
      n166 = control-ref of="Target.Y::4"() -> (w152:refnum<vi>)
      n167 = control-ref of="Target.X::5"() -> (w151:refnum<vi>)
      n168 = control-ref of="Target.Y::5"() -> (w150:refnum<vi>)
      n169 = control-ref of="Target.X::6"() -> (w149:refnum<vi>)
      n170 = control-ref of="Target.Y::6"() -> (w148:refnum<vi>)
      n171 = control-ref of="Target.X::7"() -> (w147:refnum<vi>)
      n172 = control-ref of="Target.Y::7"() -> (w146:refnum<vi>)
      n173 = control-ref of="Target.X::8"() -> (w145:refnum<vi>)
      n174 = control-ref of="Target.Y::8"() -> (w144:refnum<vi>)
      n175 = control-ref of="Target.X::9"() -> (w121:refnum<vi>)
      n176 = control-ref of="Target.Y::9"() -> (w120:refnum<vi>)
      n177 = control-ref of="Target.X::10"() -> (w119:refnum<vi>)
      n178 = control-ref of="Target.Y::10"() -> (w118:refnum<vi>)
      n179 = control-ref of="Target.X::11"() -> (w117:refnum<vi>)
      n180 = control-ref of="Target.Y::11"() -> (w116:refnum<vi>)
      n181 = control-ref of="Target.X::12"() -> (w115:refnum<vi>)
      n182 = control-ref of="Target.Y::12"() -> (w114:refnum<vi>)
      n183 = call "IMAQ Create"("Image Name"="GUIdevice 8", "Image Type"=w104) -> ("New Image"=→"image::8":T8)  [unwired: 3 in, 1 out]
      n184 = call "IMAQ Create"("Image Name"="GUIdevice 9", "Image Type"=w104) -> ("New Image"=→"image::9":T8)  [unwired: 3 in, 1 out]
      n185 = call "IMAQ Create"("Image Name"="GUIdevice 10", "Image Type"=w104) -> ("New Image"=→"image::10":T8)  [unwired: 3 in, 1 out]
      n186 = call "IMAQ Create"("Image Name"="GUIdevice 6", "Image Type"=w104) -> ("New Image"=→"image::6":T8)  [unwired: 3 in, 1 out]
      n187 = call "IMAQ Create"("Image Name"="GUIdevice 7", "Image Type"=w104) -> ("New Image"=→"image::7":T8)  [unwired: 3 in, 1 out]
      n188 = call "IMAQ Create"("Image Name"="GUIdevice 11", "Image Type"=w104) -> ("New Image"=→"image::11":T8)  [unwired: 3 in, 1 out]
      n189 = call "IMAQ Create"("Image Name"="GUIdevice 12", "Image Type"=w104) -> ("New Image"=→"image::12":T8)  [unwired: 3 in, 1 out]
      n190 = call "IMAQ Create"("Image Name"="GUIdevice 2") -> ("New Image"=→"image::2":T8)  [unwired: 4 in, 1 out]
      n191 = call "IMAQ Create"("Image Name"="GUIdevice 4", "Image Type"=w104) -> ("New Image"=→"image::4":T8)  [unwired: 3 in, 1 out]
      n192 = call "IMAQ Create"("Image Name"="GUIdevice 1", "Image Type"=w104) -> ("New Image"=→"image::1":T8)  [unwired: 3 in, 1 out]
      n193 = call "IMAQ Create"("Image Name"="GUIdevice 3", "Image Type"=w104) -> ("New Image"=→"image::3":T8)  [unwired: 3 in, 1 out]
      n194 = call "IMAQ Create"("Image Name"="GUIdevice 5", "Image Type"=w104) -> ("New Image"=→"image::5":T8)  [unwired: 3 in, 1 out]
      n195 = Build Array("GUIdevice 1", "GUIdevice 2", "GUIdevice 3", "GUIdevice 4", "GUIdevice 5", "GUIdevice 6", "GUIdevice 7", "GUIdevice 8", "GUIdevice 9", "GUIdevice 10", "GUIdevice 11", "GUIdevice 12") -> (w133:string[])
      "CCDs" <- w133
      n196 = property on="image::8" class="ImageControl"("Caption.Text"="GUIdevice 8") -> ()  [unwired: 2 in, 2 out]
      n197 = property on="image::10" class="ImageControl"("Caption.Text"="GUIdevice 10") -> ()  [unwired: 2 in, 2 out]
      n198 = property on="image::9" class="ImageControl"("Caption.Text"="GUIdevice 9") -> ()  [unwired: 2 in, 2 out]
      n199 = property on="image::1" class="ImageControl"("Caption.Text"="GUIdevice 1") -> ()  [unwired: 2 in, 2 out]
      n200 = property on="image::2" class="ImageControl"("Caption.Text"="GUIdevice 2") -> ()  [unwired: 2 in, 2 out]
      n201 = property on="image::3" class="ImageControl"("Caption.Text"="GUIdevice 3") -> ()  [unwired: 2 in, 2 out]
      n202 = property on="image::4" class="ImageControl"("Caption.Text"="GUIdevice 4") -> ()  [unwired: 2 in, 2 out]
      n203 = property on="image::5" class="ImageControl"("Caption.Text"="GUIdevice 5") -> ()  [unwired: 2 in, 2 out]
      n204 = property on="image::6" class="ImageControl"("Caption.Text"="GUIdevice 6") -> ()  [unwired: 2 in, 2 out]
      n205 = property on="image::7" class="ImageControl"("Caption.Text"="GUIdevice 7") -> ()  [unwired: 2 in, 2 out]
      n206 = property on="image::11" class="ImageControl"("Caption.Text"="GUIdevice 11") -> ()  [unwired: 2 in, 2 out]
      n207 = property on="image::12" class="ImageControl"("Caption.Text"="GUIdevice 12") -> ()  [unwired: 2 in, 2 out]
      n208 = Array To Cluster(array=w133) -> (cluster=→"Cameras":T20)
      n209 = Bundle("Target.X::1"=w159, "Target.Y::1"=w158) -> (w143:T21)  [unwired: 1 in]
      n210 = Bundle("Target.X::2"=w157, "Target.Y::2"=w156) -> (w142:T22)  [unwired: 1 in]
      n211 = Bundle("Target.X::3"=w155, "Target.Y::3"=w154) -> (w141:T23)  [unwired: 1 in]
      n212 = Bundle("Target.X::4"=w153, "Target.Y::4"=w152) -> (w134:T24)  [unwired: 1 in]
      n213 = Bundle("Target.X::5"=w151, "Target.Y::5"=w150) -> (w140:T25)  [unwired: 1 in]
      n214 = Bundle("Target.X::6"=w149, "Target.Y::6"=w148) -> (w139:T26)  [unwired: 1 in]
      n215 = Bundle("Target.X::7"=w147, "Target.Y::7"=w146) -> (w138:T27)  [unwired: 1 in]
      n216 = Bundle("Target.X::8"=w145, "Target.Y::8"=w144) -> (w137:T28)  [unwired: 1 in]
      n217 = Bundle("Target.X::12"=w115, "Target.Y::12"=w114) -> (w110:T29)  [unwired: 1 in]
      n218 = Bundle("Target.X::9"=w121, "Target.Y::9"=w120) -> (w113:T30)  [unwired: 1 in]
      n219 = Bundle("Target.X::10"=w119, "Target.Y::10"=w118) -> (w112:T31)  [unwired: 1 in]
      n220 = Bundle("Target.X::11"=w117, "Target.Y::11"=w116) -> (w111:T32)  [unwired: 1 in]
      n221 = property on="CCDs" class="Ring (strict)"("Strings []"=w133) -> ()  [unwired: 2 in, 2 out]
      n222 = Build Array(w143, w142, w141, w134, w140, w139, w138, w137, w113, w112, w111, w110) -> (w136:T33)
      n223 = Tick Count (ms)() -> (millisecond timer value=→"millisecond timer value":u32)
      n224 = property on="Feedback Global" class="Bool (strict)"("Value"=FALSE ("Feedback Global")) -> ()  [unwired: 2 in, 2 out]
      n225 = Get Date/Time In Seconds() -> (seconds since 1Jan1904=w123:timestamp)
      n226 = Format Date/Time String(time format string (%c)="%Y%m%d%H%M", seconds (now)=w123) -> (date/time string=w122:string)  [unwired: 1 in]
      n227 = Concatenate Strings(w122, "Beampointing_Pico.tdms" ("string")) -> (w126:string)
      n228 = String To Path(string=w126) -> (path=w125:path)
      n229 = Build Path(base path=path "W:/BP_DATA", name or relative path=w125) -> (appended path=w128:path)
      n230 = call <vilib>:"Add State(s) to Queue__jki_lib_state_machine.vi"("State(s) in (\"\")"="Macro: Initialize") -> ("States Out"=w234:string)  [unwired: 14 in]
      n231 = Create User Event(user event datatype=T13 {"EventEnum"=enum."new data", "Device name"="Device name"} ("New Event")) -> (user event=w242:refnum<user-event>, error out=w244:errorcluster)  [unwired: 1 in]
      "tcp data event" <- w242
      n232 = while "JKI - String-Based Queued State Machine (Basic) v1.0" {
        shift-right: [w271] -> w132
        shift-left: _ -> [w259]
        shift-right: [w274] -> w160
        shift-left: _ -> [w270]
        shift-right: [w273] -> _
        shift-left: w234 -> [w275]
        tunnel: w136 -> [w268]
        tunnel: w133 -> [w266]
        tunnel: [w266] -> w161
        tunnel: w136 -> [w267]
        tunnel: w128 -> [w257]
        stop <- w272 stop-if-true
        n233 = Unbundle By Name(w259) -> ("active cams"=w258:string[])
        n234 = call <vilib>:"Parse State Queue__jki_lib_state_machine.vi"("State Queue"=w275, "Error In (no error)"=w270) -> ("Remaining States"=w277:string, "Current State"=w278:string, "Arguments"=w276:string)  [unwired: 11 in]
        "Current State" <- w278
        n235 = case shown="\"detected\"" w278 {
          selector: w278 -> [_ _ w565 _ _ _ _ _ _ _ _ _ _ _ _ _ _ _ _ _ _ _ _ _ _ _ _ _ _ _ _ _ _ _ _ _ _ _ _]
          tunnel: w277 -> [w309 w564 w569 w587 w593 w598 w602 w634 w642 w646 w650 w656 w667 w691 w696 w706 w710 w726 w804 w843 w856 w865 w893 w914 w918 w920 w1063 w1173 w1259 w1325 w1363 w1383 w1398 w1472 w1524 w1534 w1554 w1574 w1601]
          tunnel: w276 -> [_ _ _ _ _ _ _ _ _ _ _ w651 w662 _ _ _ _ _ _ _ w853 _ _ _ _ w922 _ w1148 w1234 _ _ _ _ _ _ _ _ _ _]
          tunnel: w259 -> [w307 w561 w567 w577 w590 w596 w599 _ w638 w643 w648 w654 w661 w688 w693 w698 w707 w719 w785 w841 w848 w861 w885 w907 w915 w946 w1078 w1166 w1252 w1322 w1334 w1380 w1395 w1470 w1521 w1531 w1538 w1571 w1592]
          tunnel: [w306 w562 w571 w585 errorcluster {"status"=FALSE, "code"=0, "source"=""} ("error out") w595 w600 w606 w635 w644 w647 w652 w664 w689 w694 w704 w708 w711 w749 w832 w854 w863 w891 w912 w916 w925 w1090 w1171 w1257 w1323 w1361 w1381 w1396 w1460 w1522 w1532 w1542 w1572 w1599] -> w274
          tunnel: w270 -> [w305 w562 w570 w585 w589 w595 w600 w607 w640 w644 w647 w653 w665 w689 w694 w704 w708 w711 w748 w833 w854 w863 w891 w912 w916 w925 w1090 w1171 w1257 w1323 w1361 w1381 w1396 w1465 w1522 w1532 w1536 w1572 w1599]
          tunnel: [w308 w563 w568 w586 w592 w597 w601 w633 w641 w645 w649 w655 w666 w690 w695 w705 w709 w725 w803 w842 w855 w864 w892 w913 w917 w935 w1091 w1172 w1258 w1324 w1362 w1382 w1397 w1471 w1523 w1533 w1553 w1573 w1600] -> w273
          tunnel: [_ _ _ _ _ TRUE _ _ _ _ _ _ _ _ _ _ _ _ _ _ _ _ _ _ _ _ _ _ _ _ _ _ _ _ _ _ _ _ _] -> w272
          tunnel: [w302 w561 w567 w576 w590 w596 w599 w628 w638 w643 w648 w654 w661 w688 w693 w698 w707 w712 w784 w841 w847 w860 w884 w906 w915 w963 w1078 w1166 w1252 w1321 w1334 w1380 w1395 w1470 w1520 w1531 w1539 w1571 w1591] -> w271
          tunnel: "update speed [ms]" -> [w304 _ _ _ _ _ _ _ _ _ _ _ _ _ _ _ _ _ _ _ _ _ _ _ _ _ _ _ _ _ _ _ _ _ _ _ _ _ _]
          tunnel: w268 -> [w301 _ _ _ _ _ _ _ _ _ _ _ _ _ _ _ _ _ _ _ _ _ _ _ _ w959 _ _ _ _ _ _ _ _ _ _ _ w1555 _]
          tunnel: w266 -> [w303 _ _ _ _ _ _ _ _ _ _ _ _ _ _ _ _ w724 w783 _ w849 _ _ _ _ w929 _ w1170 w1256 _ w1335 _ w1384 w1468 _ _ _ _ _]
          tunnel: w257 -> [_ _ _ _ _ _ _ w603 _ _ _ _ _ _ _ _ _ _ _ _ _ _ _ _ _ _ _ _ _ _ _ _ _ _ _ _ _ _ _]
          frame "", "Idle" {
            # "executes when the state queue is empty"
            n236 = event shown="[0] Timeout" {
              selector: _ -> [_ _ _ _ _ _ _ _ _ _ _ _ _ _ _ _ _]
              dyn-events: _ -> [_ _ _ _ _ _ _ _ _ _ _ _ _ _ _ _ _]
              timeout: w304 -> [_ _ _ _ _ _ _ _ _ _ _ _ _ _ _ _ _]
              tunnel: w309 -> [w343 w450 w465 w484 w489 w494 w499 w505 w512 w519 w524 w529 w534 w543 w548 w554 w560]
              tunnel: [w318 w449 w464 w483 w488 w493 w498 w504 w511 w518 w523 w528 w533 w542 w547 w553 w559] -> w308
              tunnel: w307 -> [w328 w447 w461 w480 w486 w491 w496 w502 w509 w516 w521 w526 w531 w536 w545 w551 w557]
              tunnel: [w310 w448 w463 w482 w487 w492 w497 w503 w510 w517 w522 w527 w532 w541 w546 w552 w558] -> w306
              tunnel: w305 -> [w313 w448 w463 w482 w487 w492 w497 w503 w510 w517 w522 w527 w532 w541 w546 w552 w558]
              tunnel: [w316 w447 w461 w479 w486 w491 w496 w502 w509 w516 w521 w526 w531 w536 w545 w551 w557] -> w302
              tunnel: w303 -> [w339 _ w457 _ _ _ _ _ _ _ _ _ _ _ _ _ _]
              tunnel: w301 -> [_ _ w459 _ _ _ _ _ _ _ _ _ _ _ _ _ _]
              event Timeout {
                n237 = event-data() -> ()  [unwired: 1 in, 1 out]
                n238 = Unbundle By Name(w328) -> ("Centroid X"=w336:dbl[][], "Centroid Y"=w350:dbl[][], "Size"=w342:dbl[][], "detection para"=w338:T2[], "active cams"=w331:string[], "thresholds"=w326:cluster{"Lower value":sgl, "Upper value":sgl}[])
                n239 = call <userlib>:"Tick Count (ms)__ogtk.vi"("error in (no error)"=w313) -> ("error out"=w312:errorcluster, "millisecond timer value"=→"millisecond timer 2":u32)  [unwired: 9 in]
                n240 = for {
                  tunnel: w331 -> [w388] mode=indexing
                  tunnel: [w402] -> w349 mode=indexing
                  tunnel: [w399] -> w351 mode=indexing
                  tunnel: [w405] -> w348 mode=indexing
                  tunnel: w336 -> [w385]
                  tunnel: w350 -> [w383]
                  tunnel: w342 -> [w380]
                  tunnel: [w398] -> w341 mode=indexing
                  tunnel: w339 -> [w395]
                  tunnel: w338 -> [w393]
                  tunnel: [w391] -> w314 mode=indexing
                  tunnel: [w390] -> w337 mode=indexing
                  tunnel: [w387] -> w332 mode=indexing
                  tunnel: [w378] -> w329 mode=indexing
                  tunnel: "autodetect" -> [w377]
                  tunnel: w326 -> [w376] mode=indexing
                  tunnel: w312 -> [w396]
                  tunnel: [w397] -> w340
                  i -> [w381]
                  w401 = dbl[] [] ("Array 4")
                  n241 = Index Array(array=w380, index (row)=w381) -> (element=w379:dbl[])  [unwired: 1 in]
                  n242 = Index Array(array=w383, index (row)=w381) -> (element=w382:dbl[])  [unwired: 1 in]
                  n243 = call-poly <userlib>:"Filter 1D Array__ogtk.vi"("items to filter"=w388, "array"=w395) -> ("filtered item indices"=w394:i32[])  [unwired: 4 in, 1 out]
                  n244 = Index Array(array=w385, index (row)=w381) -> (element=w384:dbl[])  [unwired: 1 in]
                  n245 = Index Array(array=w394) -> (element=w386:i32)  [unwired: 1 in]
                  n246 = Index Array(array=w393, index=w386) -> (element=w389:T2)
                  n247 = call "CENTRIOD DETECTION.vi"("Refnum in"=w388, "auto threshold"=w377, "Threshold Range In"=w376, "beam detection para"=w389, "error in (no error)"=w396) -> ("Bounding Rect"=w387:T34, "Particle Reports (Pixels)"=w390:T35, "Threshold Range Out"=w378:cluster{"Lower value":sgl, "Upper value":sgl}, "Centriod"=w410:cluster{"X":dbl, "Y":dbl}, "error out"=w397:errorcluster)  [unwired: 7 in, 3 out]
                  n248 = Unbundle By Name(w410) -> ("X"=w407:dbl, "Y"=w406:dbl)
                  n249 = Empty Array?(array=w390) -> (empty?=w392:bool)
                  n250 = Not Equal To 0?(x=w406) -> (x != 0?=w408:bool)
                  n251 = Not Equal To 0?(x=w407) -> (x != 0?=w409:bool)
                  n252 = Not(x=w392) -> (.not. x?=w391:bool)
                  n253 = And(x=w409, y=w408) -> (x .and. y?=w404:bool)
                  n254 = case shown="True" w404 {
                    tunnel: w407 -> [_ w443]
                    tunnel: w406 -> [_ w442]
                    tunnel: w384 -> [w429 w445]
                    tunnel: w382 -> [w428 w444]
                    tunnel: [w429 w441] -> w403
                    tunnel: [w428 w440] -> w400
                    tunnel: w387 -> [_ w439]
                    tunnel: w379 -> [w427 w432]
                    tunnel: [w427 w430] -> w398
                    frame False {
                    }
                    frame True {
                      n255 = Unbundle By Name(w439) -> ("Right"=w438:dbl, "Left"=w437:dbl, "Bottom"=w436:dbl, "Top"=w435:dbl)
                      n256 = Subtract(x=w438, y=w437) -> (x-y=w433:dbl)
                      n257 = Subtract(x=w436, y=w435) -> (x-y=w434:dbl)
                      n258 = Build Array (concatenate)(w445, w443) -> (w441:dbl[])
                      n259 = Multiply(x=w433, y=w434) -> (x*y=w431:dbl)
                      n260 = Build Array (concatenate)(w444, w442) -> (w440:dbl[])
                      n261 = Build Array (concatenate)(w432, w431) -> (w430:dbl[])
                    }
                  }
                  n262 = for {
                    tunnel: w403 -> [w420] mode=indexing
                    shift-right: [w419] -> w402
                    shift-left: w401 -> [w421]
                    n263 = Not Equal To 0?(x=w420) -> (x != 0?=w422:bool)
                    n264 = case shown="True" w422 {
                      tunnel: w421 -> [w423 w426]
                      tunnel: w420 -> [_ w425]
                      tunnel: [w423 w424] -> w419
                      frame False {
                      }
                      frame True {
                        n265 = Build Array (concatenate)(w426, w425) -> (w424:dbl[])
                      }
                    }
                  }
                  n266 = for {
                    tunnel: w400 -> [w412] mode=indexing
                    shift-right: [w411] -> w399
                    shift-left: w401 -> [w413]
                    n267 = Not Equal To 0?(x=w412) -> (x != 0?=w414:bool)
                    n268 = case shown="True" w414 {
                      tunnel: w413 -> [w415 w418]
                      tunnel: w412 -> [_ w417]
                      tunnel: [w415 w416] -> w411
                      frame False {
                      }
                      frame True {
                        n269 = Build Array (concatenate)(w418, w417) -> (w416:dbl[])
                      }
                    }
                  }
                  n270 = Array Size(array=w399) -> (size(s)=w405:i32)
                }
                "detected" <- w314
                "Particle Reports (Pixels)" <- w337
                "Box" <- w332
                n271 = Bundle(0, 1, "Centroid X"=w336) -> (→"Status":cluster{i32, i32, "Centroid X":dbl[][]})  [unwired: 1 in]
                n272 = call <vilib>:"Clear Errors.vi"("error in (no error)"=w340) -> ("error out"=w310:errorcluster)  [unwired: 6 in]
                n273 = local read "img to avg"() -> (w320:i32)
                n274 = local read "Numeric"() -> (w323:dbl)
                n275 = Bundle By Name(cluster=w328, "thresholds"=w329) -> (w327:T36)
                n276 = Increment(x=w320) -> (x+1=w319:i32)
                n277 = Greater Or Equal?(x=w323, y=w319) -> (x >= y?=w315:bool)
                n278 = Increment(x=w323) -> (x+1=w322:dbl)
                n279 = Select(t=0.0, s=w315, f=w322) -> (s? t:f=w321:dbl)
                n280 = local write "Numeric"(w321) -> ()
                n281 = for {
                  tunnel: w348 -> [w368] mode=indexing
                  tunnel: w331 -> [w375] mode=indexing
                  shift-right: [w370] -> w344
                  shift-left: "" ("GUIdevice 7") -> [w373]
                  tunnel: [w363] -> w346 mode=indexing
                  tunnel: "Detection Rate" -> [w367]
                  tunnel: w321 -> [w365]
                  n282 = local read "img to avg"() -> (w369:i32)
                  n283 = Greater Or Equal?(x=w368, y=w369) -> (x >= y?=w364:bool)
                  n284 = Multiply(x=w367, y=w365) -> (x*y=w366:dbl)
                  n285 = Greater Or Equal?(x=w368, y=w366) -> (x >= y?=w362:bool)
                  n286 = And(x=w364, y=w362) -> (x .and. y?=w363:bool)
                  n287 = Select(t=w375, s=w363, f="") -> (s? t:f=w371:string)
                  n288 = Concatenate Strings(w373, "\t", w371) -> (w370:string)
                }
                n289 = Bundle By Name(cluster=w327, "Centroid X"=w349, "Centroid Y"=w351, "Size"=w341) -> (w317:T36)
                n290 = Or Array Elements(Boolean array=w346) -> (logical OR=w345:bool)
                n291 = case shown="True" w315 {
                  tunnel: w317 -> [w352 w355]
                  tunnel: [w352 w354] -> w316
                  frame False {
                  }
                  frame True {
                    n292 = local read "Centroid X"() -> (w353:dbl[][])
                    n293 = Bundle By Name(cluster=w355, "Centroid X"=w353, "Centroid Y"=w353, "Size"=w353) -> (w354:T36)
                  }
                }
                n294 = case shown="True" w345 {
                  tunnel: w344 -> [_ w360]
                  tunnel: w343 -> [w356 w358]
                  tunnel: [w356 w357] -> w318
                  frame False {
                  }
                  frame True {
                    n295 = call <vilib>:"Build State String with Arguments__jki_lib_state_machine.vi"("Arguments (\"\")"=w360, "State"="detected") -> ("State with Arguments"=w359:string)  [unwired: 4 in]
                    n296 = call <vilib>:"Add State(s) to Queue__jki_lib_state_machine.vi"("State(s) in (\"\")"=w358, "State(s) at Back (\"\")"=w359) -> ("States Out"=w357:string)  [unwired: 13 in]
                  }
                }
              }
              event "stop": Value Change {
                # "Exit Button Value Change (pressed) Event\n(this executes Macro: Exit to terminate the VI)"
                n297 = event-data() -> ()  [unwired: 1 in, 6 out]
                n298 = call <vilib>:"Add State(s) to Queue__jki_lib_state_machine.vi"("State(s) in Front (\"\")"="Macro: Exit", "State(s) in (\"\")"=w450) -> ("States Out"=w449:string)  [unwired: 13 in]
              }
              event Value Change {
                n299 = event-data() -> ()  [unwired: 1 in, 6 out]
                n300 = property on="Set Centriod Target" class="Bool (strict)"("Value"=FALSE) -> ()  [unwired: 2 in, 2 out]
                n301 = Unbundle By Name(w461) -> ("active ccd"=w453:i32, "Centroid X"=w452:dbl[][], "Centroid Y"=w451:dbl[][])
                n302 = Index Array(array=w457, index=w453) -> (element=w456:string)
                n303 = Concatenate Strings("Do want to update the target of " ("message"), w456, "?" ("string")) -> (w454:string)
                n304 = Two Button Dialog(message=w454) -> (T button?=w460:bool)  [unwired: 2 in]
                n305 = case shown="True" w460 {
                  tunnel: w459 -> [_ w472]
                  tunnel: w453 -> [_ w471]
                  tunnel: w452 -> [_ w478]
                  tunnel: w451 -> [_ w473]
                  frame False {
                  }
                  frame True {
                    n306 = Index Array(array=w478, index (row)=w471) -> (element=w477:dbl[])  [unwired: 1 in]
                    n307 = Index Array(array=w473, index (row)=w471) -> (element=w474:dbl[])  [unwired: 1 in]
                    n308 = Index Array(array=w472, index=w471) -> (element=w470:T29)
                    n309 = Unbundle By Name(w470) -> ("Target.X::12"=w469:refnum<vi>, "Target.Y::12"=w467:refnum<vi>)
                    n310 = Reverse 1D Array(array=w477) -> (reversed array=w476:dbl[])
                    n311 = Reverse 1D Array(array=w474) -> (reversed array=w475:dbl[])
                    n312 = Index Array(array=w476) -> (element=w468:dbl)  [unwired: 1 in]
                    n313 = Index Array(array=w475) -> (element=w466:dbl)  [unwired: 1 in]
                    n314 = property class="DigNum (strict)"(reference=w469, "Val(Sgnl)"=w468) -> ()  [unwired: 1 in, 2 out]
                    n315 = property class="DigNum (strict)"(reference=w467, "Val(Sgnl)"=w466) -> ()  [unwired: 1 in, 2 out]
                  }
                }
                n316 = call <vilib>:"Add State(s) to Queue__jki_lib_state_machine.vi"("State(s) in (\"\")"=w465) -> ("States Out"=w464:string)  [unwired: 14 in]
              }
              event "Feedback Global": Value Change {
                # "Exit Button Value Change (pressed) Event\n(this executes Macro: Exit to terminate the VI)"
                n317 = event-data() -> ("NewVal"=w481:bool)  [unwired: 1 in, 5 out]
                n318 = call <vilib>:"Add State(s) to Queue__jki_lib_state_machine.vi"("State(s) in (\"\")"=w484) -> ("States Out"=w483:string)  [unwired: 14 in]
                n319 = Bundle By Name(cluster=w480, "Feedback global"=w481) -> (w479:T36)
              }
              event Value Change {
                n320 = event-data() -> ()  [unwired: 1 in, 6 out]
                n321 = call <vilib>:"Add State(s) to Queue__jki_lib_state_machine.vi"("State(s) in Front (\"\")"="Move Config", "State(s) in (\"\")"=w489) -> ("States Out"=w488:string)  [unwired: 13 in]
              }
              event Value Change {
                n322 = event-data() -> ()  [unwired: 1 in, 6 out]
                n323 = call <vilib>:"Add State(s) to Queue__jki_lib_state_machine.vi"("State(s) in Front (\"\")"="Detection Config", "State(s) in (\"\")"=w494) -> ("States Out"=w493:string)  [unwired: 13 in]
              }
              event "associated motors": Value Change {
                n324 = event-data() -> ()  [unwired: 1 in, 6 out]
                n325 = call <vilib>:"Add State(s) to Queue__jki_lib_state_machine.vi"("State(s) in (\"\")"=w499, "State(s) at Back (\"\")"="Motor Config" ("State(s) at Back (\"\")")) -> ("States Out"=w498:string)  [unwired: 13 in]
              }
              event "Reset History": Value Change {
                n326 = event-data() -> ()  [unwired: 1 in, 6 out]
                n327 = call <vilib>:"Add State(s) to Queue__jki_lib_state_machine.vi"("State(s) in (\"\")"=w505, "State(s) at Back (\"\")"="Reset History" ("State(s) at Back (\"\")")) -> ("States Out"=w504:string)  [unwired: 13 in]
                n328 = property on="Reset History" class="Bool (strict)"("Value"=FALSE ("Reset History")) -> ()  [unwired: 2 in, 2 out]
              }
              event "ActiveMotor": Value Change {
                n329 = event-data() -> ("NewVal"=w507:u16)  [unwired: 1 in, 5 out]
                n330 = property on="ActiveMotor" class="Ring (strict)"() -> ("Strings []"=w508:string[])  [unwired: 2 in, 2 out]
                n331 = Index Array(array=w508, index=w507) -> (element=w506:string)
                n332 = property on="ActiveMotorName::99" class="Str"("Val(Sgnl)"=w506) -> ()  [unwired: 2 in, 2 out]
                n333 = call <vilib>:"Add State(s) to Queue__jki_lib_state_machine.vi"("State(s) in (\"\")"=w512) -> ("States Out"=w511:string)  [unwired: 14 in]
              }
              event "ActiveMotor 2": Value Change {
                n334 = event-data() -> ("NewVal"=w515:u16)  [unwired: 1 in, 5 out]
                n335 = property on="ActiveMotor 2" class="Ring (strict)"() -> ("Strings []"=w513:string[])  [unwired: 2 in, 2 out]
                n336 = Index Array(array=w513, index=w515) -> (element=w514:string)
                n337 = property on="ActiveMotorName::98" class="Str"("Val(Sgnl)"=w514) -> ()  [unwired: 2 in, 2 out]
                n338 = call <vilib>:"Add State(s) to Queue__jki_lib_state_machine.vi"("State(s) in (\"\")"=w519) -> ("States Out"=w518:string)  [unwired: 14 in]
              }
              event "Save Config": Value Change {
                n339 = event-data() -> ()  [unwired: 1 in, 6 out]
                n340 = call <vilib>:"Add State(s) to Queue__jki_lib_state_machine.vi"("State(s) in (\"\")"=w524, "State(s) at Back (\"\")"="Save Config" ("State(s) at Back (\"\")")) -> ("States Out"=w523:string)  [unwired: 13 in]
              }
              event "Load Config": Value Change {
                n341 = event-data() -> ()  [unwired: 1 in, 6 out]
                n342 = call <vilib>:"Add State(s) to Queue__jki_lib_state_machine.vi"("State(s) in (\"\")"=w529, "State(s) at Back (\"\")"="Load Config" ("State(s) at Back (\"\")")) -> ("States Out"=w528:string)  [unwired: 13 in]
              }
              event "Save Stats": Value Change {
                n343 = event-data() -> ()  [unwired: 1 in, 6 out]
                n344 = call <vilib>:"Add State(s) to Queue__jki_lib_state_machine.vi"("State(s) in (\"\")"=w534, "State(s) at Back (\"\")"="Save Stats" ("State(s) at Back (\"\")")) -> ("States Out"=w533:string)  [unwired: 13 in]
              }
              event "active CCDs": Value Change {
                n345 = event-data() -> ("NewVal"=w540:i32)  [unwired: 1 in, 5 out]
                n346 = Unbundle By Name(w536) -> ("active cams"=w535:string[])
                n347 = Index Array(array=w535, index=w540) -> (element=w538:string)
                n348 = call <vilib>:"Build State String with Arguments__jki_lib_state_machine.vi"("Arguments (\"\")"=w538, "State"="active" ("State(s) at Back (\"\")")) -> ("State with Arguments"=w537:string)  [unwired: 4 in]
                n349 = call <vilib>:"Add State(s) to Queue__jki_lib_state_machine.vi"("State(s) in (\"\")"=w543, "State(s) at Back (\"\")"=w537) -> ("States Out"=w542:string)  [unwired: 13 in]
              }
              event "Center": Value Change {
                n350 = event-data() -> ()  [unwired: 1 in, 6 out]
                n351 = call <vilib>:"Add State(s) to Queue__jki_lib_state_machine.vi"("State(s) in (\"\")"=w548, "State(s) at Back (\"\")"="Center" ("State(s) at Back (\"\")")) -> ("States Out"=w547:string)  [unwired: 13 in]
              }
              event "new tdms": Value Change {
                n352 = event-data() -> ()  [unwired: 1 in, 6 out]
                n353 = property on="new tdms" class="Bool (strict)"("Value"=FALSE ("new tdms")) -> ()  [unwired: 2 in, 2 out]
                n354 = call <vilib>:"Add State(s) to Queue__jki_lib_state_machine.vi"("State(s) in (\"\")"=w554, "State(s) at Back (\"\")"="newtdms" ("State(s) at Back (\"\")")) -> ("States Out"=w553:string)  [unwired: 13 in]
              }
              event Panel Close? {
                # "Discard the event because we'll close the front panel ourselves in Macro: Exit"
                # "Close Panel button (pressed) Event\n(this executes Macro: Exit to terminate the VI)"
                n355 = event-data() -> ()  [unwired: 1 in, 1 out]
                n356 = call <vilib>:"Add State(s) to Queue__jki_lib_state_machine.vi"("State(s) in Front (\"\")"="Macro: Exit", "State(s) in (\"\")"=w560) -> ("States Out"=w559:string)  [unwired: 13 in]
                n357 = event-data("Discard?"=TRUE) -> ()  [unwired: 1 in, 1 out]
              }
            }
          }
          frame "---------- Core ----------" {
            # "Do not put any code in this frame.\n(it is a separator no-op)"
            n358 = call <vilib>:"Add State(s) to Queue__jki_lib_state_machine.vi"("State(s) in (\"\")"=w564) -> ("States Out"=w563:string)  [unwired: 14 in]
          }
          frame Default {
            w574 = 42 items=["No error", "Argument error", "Memory is full", "Out of zone", "End of file", "File already open", "Generic file I/O error", "File not found", "File permission error", "Disk is full", "Duplicate path", "Too many files open", "System feature not enabled", "Resource file not found", "Cannot add resource", "Resource not found", "Image not found", "Image memory error", "Pen does not exist", "Config type invalid", "Config token not found", "Config parse error", "Config memory error", "Bad external code format", "Bad external code offset", "External code not present", "Null window", "Destroy window error", "Null menu", "Print aborted", "Bad print record", "Print driver error", "Windows error during printing", "Memory error during printing", "Print dialog error", "Generic print error", "Invalid device refnum", "Device not found", "Device parameter error", "Device unit error", "Cannot open device", "Device call aborted", "Generic error", "Cancelled by user", "Object ID too low", "Object ID too high", "Object not in heap", "Unknown heap", "Unknown object (invalid DefProc)", "Unknown object (DefProc not in table)", "Message out of range", "Invalid (null) method", "Unknown message", "Manager call not supported", "Bad address", "Network operation in progress", "Network operation timed out", "Connection is busy", "Network attribute not supported", "Network error", "Address in use", "System out of memory", "Connection aborted", "Connection refused", "Not connected", "Already connected", "Connection closed", "Initialization error (interapplication manager)", "Bad occurrence", "Wait on unbound occurrence handler", "Occurrence queue overflow", "Datalog type conflict", "Unused", "Unrecognized type (interapplication manager)", "Memory corrupt", "Failed to make temporary DLL", "Old CIN version", "Drag socket not found", "Failed to load drop-object", "Failed to register OLE object", "Failed to release OLE object", "Format specifier type mismatch", "Unknown format specifier", "Too few format specifiers", "Too many format specifiers", "Scan failed", "Newer CIN version", "Error converting to variant", "Runtime menu error", "Password tampered", "Variant attribute not found", "Incompatible variant data type", "Event data is not available", "Event Store is not present", "Occurrence is not found", "Event Queue is not created", "Event info is not available", "Refnum passed is NULL", "Error retrieving Class GUID", "Error retrieving CoClass GUID", "Error retrieving TypeLib GUID.", "Bad built application magic bytes.", "Specific driver is different from the specific driver associated with the Logical Name.", "There is no session opened to the class driver.", "Max Error", "MAX - Error with config objects", "MAX - Error loading configuration", "MAX - Group not supported"]
            # "Current State"
            # "Do not delete, rename, or modify this frame.\n(this is used to capture unhandled states and typos)"
            # "Handle mistyped state name (developer tool)"
            n359 = Format Into String(format string="Software Exception: Unhandled State \"%s\"." ("message"), error in=w570, w565) -> (resulting string=w573:string, error out=w572:errorcluster)  [unwired: 1 in]
            n360 = call <vilib>:"Error Cluster From Error Code.vi"("show call chain? (False)"=TRUE, "error in (no error)"=w572, "error message (\"\")"=w573, "error code (0)"=w574) -> ("error out"=w571:errorcluster)  [unwired: 5 in]
            n361 = call <vilib>:"Add State(s) to Queue__jki_lib_state_machine.vi"("State(s) in (\"\")"=w569) -> ("States Out"=w568:string)  [unwired: 14 in]
          }
          frame "Initialize Core Data" {
            # "Do not delete, rename, or modify this frame.\n(this is used to determine panel behavior on exit)"
            # "originally closed?"
            # "exe?"
            # "If panel starts closed or is an EXE, then close it when we exit"
            n362 = property class="VI"() -> ("Front Panel.Open"=w584:bool)  [unwired: 2 in, 2 out]
            n363 = property class="App"() -> ("App.Kind"=w583:T15)  [unwired: 2 in, 2 out]
            n364 = control-ref of="Current VI Reference"() -> (w578:refnum<vi>)
            n365 = Not(x=w584) -> (.not. x?=w581:bool)
            n366 = Equal?(x=w583, y=T15."Run Time System" ("Application:Kind")) -> (x = y?=w580:bool)
            n367 = Or(x=w581, y=w580) -> (x .or. y?=w579:bool)
            n368 = Bundle By Name(cluster=w577, "Core.Current VI Reference"=w578, "Core.Close Panel on Exit?"=w579) -> (w576:T36)
            n369 = call <vilib>:"Add State(s) to Queue__jki_lib_state_machine.vi"("State(s) in (\"\")"=w587) -> ("States Out"=w586:string)  [unwired: 14 in]
          }
          frame "Error Handler" {
            # "Unhandled Error -- Display it"
            # "Handle any errors here.\nYou can also output any states to clean-up after errors occur"
            # "Clear error"
            n370 = call <vilib>:"General Error Handler.vi"("error in (no error)"=w589) -> ()  [unwired: 10 in, 5 out]
            n371 = call <vilib>:"Add State(s) to Queue__jki_lib_state_machine.vi"("State(s) in Front (\"\")"="/* Post Error States", "State(s) in (\"\")"=w593) -> ("States Out"=w592:string)  [unwired: 13 in]
          }
          frame "Exit" {
            # "Do not put any code in this frame.\n(No errors that occur here will be handled.)"
            n372 = call <vilib>:"Add State(s) to Queue__jki_lib_state_machine.vi"("State(s) in (\"\")"=w598) -> ("States Out"=w597:string)  [unwired: 14 in]
          }
          frame "---------- Data ----------" {
            # "Do not put any code in this frame.\n(It is a separator no-op. You can make a copy of this frame to create a new Data frame)"
            n373 = call <vilib>:"Add State(s) to Queue__jki_lib_state_machine.vi"("State(s) in (\"\")"=w602) -> ("States Out"=w601:string)  [unwired: 14 in]
          }
          frame "Data: Initialize" {
            w604 = cluster{"Lower value":sgl, "Upper value":sgl}[] [{"Lower value"=93.0, "Upper value"=255.0}, {"Lower value"=105.0, "Upper value"=255.0}, {"Lower value"=0.0, "Upper value"=255.0}, {"Lower value"=127.0, "Upper value"=255.0}, {"Lower value"=0.0, "Upper value"=255.0}, {"Lower value"=0.0, "Upper value"=255.0}, {"Lower value"=0.0, "Upper value"=255.0}, {"Lower value"=0.0, "Upper value"=255.0}, {"Lower value"=0.0, "Upper value"=255.0}, {"Lower value"=0.0, "Upper value"=255.0}, {"Lower value"=0.0, "Upper value"=255.0}, {"Lower value"=0.0, "Upper value"=255.0}]  # thresholds
            w617 = FALSE  # Feedback global
            w619 = 0  # active ccd
            w631 = 20  # img to avg
            w632 = T37 {"Current VI Reference"=refnum, "Close Panel on Exit?"=FALSE}  # Core
            # "Initialize the shift-register data, here.\n(data names are defined by what you wire into the bundle function)"
            n374 = TDMS Open(6:FALSE ("disable buffering (T)"), 7:enum16{"1.0", "2.0"}."1.0" ("file format version (2.0)"), 8:w607, 10:T16."create or replace" ("operation"), 11:w603) -> (0:w606:errorcluster, 3:w605:refnum<k34>)  [unwired: 1 in]
            n375 = Bundle("Core"=w632, "detection para"="detection para", "thresholds"=w604, "Centroid X"="Centroid X", "Centroid Y"="Centroid Y", "img to avg"=w631, "Mean Centroid X"="Mean Centroid X", "Mean Centroid Y"="Mean Centroid Y", "Offset X"="Offset X", "Offset Y"="Offset Y", "Offset X stats"="Offset X stats", "Offset Y stats"="Offset Y stats", "Size"="Size", "Mean Size"="Mean Size", "Time"="Time", "move properties"="move properties", "active axis refs 2"="active axis refs 2", "active ccd"=w619, "Feedback global"=w617, "Motor X"="Motor X", "Motor Y"="Motor Y", "active cams"="active cams", "tdms file out"=w605) -> (w628:T36)  [unwired: 1 in]
            n376 = call <vilib>:"Add State(s) to Queue__jki_lib_state_machine.vi"("State(s) in (\"\")"=w634) -> ("States Out"=w633:string)  [unwired: 14 in]
          }
          frame "Data: Cleanup" {
            # "Cleanup any data and references, here.\n(this is called automatically, by the Macro: Exit)"
            n377 = Unbundle By Name(w638) -> ("Core.Current VI Reference"=w639:refnum<vi>)
            n378 = Close Reference(reference=w639, error in (no error)=w640) -> (error out=w636:errorcluster)
            n379 = Unbundle By Name(w638) -> ("tdms file out"=w637:refnum<k34>)
            n380 = TDMS Close(8:w636, 11:w637) -> (0:w635:errorcluster)  [unwired: 1 out]
            n381 = call <vilib>:"Add State(s) to Queue__jki_lib_state_machine.vi"("State(s) in (\"\")"=w642) -> ("States Out"=w641:string)  [unwired: 14 in]
          }
          frame "---------- UI ----------" {
            # "Do not put any code in this frame.\n(It is a separator no-op. You can make a copy of this frame to create a new UI frame)"
            n382 = call <vilib>:"Add State(s) to Queue__jki_lib_state_machine.vi"("State(s) in (\"\")"=w646) -> ("States Out"=w645:string)  [unwired: 14 in]
          }
          frame "UI: Initialize" {
            # "Initialize the User Interface, here.\n(this is called automatically, by the Macro: Init)"
            n383 = call <vilib>:"Add State(s) to Queue__jki_lib_state_machine.vi"("State(s) in (\"\")"=w650) -> ("States Out"=w649:string)  [unwired: 14 in]
          }
          frame "UI: Cursor Set" {
            # "Argument"
            # "Set and Unset Cursor Busy.\n(Usage: \"UI: Cursor Set >> Busy|Idle\")"
            n384 = case shown="\"Idle\", Default" w651 {
              tunnel: w653 -> [w658 w660]
              tunnel: [w657 w659] -> w652
              frame "Idle", Default {
                n385 = call <vilib>:"Unset Busy.vi"("error in (no error)"=w658) -> ("error out"=w657:errorcluster)  [unwired: 10 in]
              }
              frame "Busy" {
                n386 = call <vilib>:"Set Busy.vi"("error in (no error)"=w660) -> ("error out"=w659:errorcluster)  [unwired: 9 in, 1 out]
              }
            }
            n387 = call <vilib>:"Add State(s) to Queue__jki_lib_state_machine.vi"("State(s) in (\"\")"=w656) -> ("States Out"=w655:string)  [unwired: 14 in]
          }
          frame "UI: Front Panel State" {
            # "Argument"
            # "Set Front Panel Open or Closed\n(Usage: \"UI: Front Panel State >> Open|Close\")"
            n388 = Unbundle By Name(w661) -> ("Core.Current VI Reference"=w663:refnum<vi>)
            n389 = case shown="\"Open\", Default" w662 {
              tunnel: w665 -> [w671 w682]
              tunnel: [w672 w683] -> w664
              tunnel: w663 -> [_ _]
              frame "Open", Default {
                n390 = property class="VI"(error in=w671) -> (reference out=w669:refnum<vi>, error out=w670:errorcluster, "Front Panel.Open"=w668:bool)  [unwired: 1 in]
                n391 = case shown="False" w668 {
                  tunnel: [w675 w678] -> w672
                  tunnel: w670 -> [w674 w678]
                  tunnel: w669 -> [w673 _]
                  frame False {
                    n392 = invoke class="VI" method="FP.Open"(reference=w673, error in=w674, "Activate"=TRUE, "State"=T17."Standard") -> (error out=w675:errorcluster)  [unwired: 1 in, 4 out]
                  }
                  frame True {
                  }
                }
              }
              frame "Close" {
                n393 = property class="VI"(error in=w682) -> (reference out=w680:refnum<vi>, error out=w681:errorcluster, "Front Panel.Open"=w679:bool)  [unwired: 1 in]
                n394 = case shown="True" w679 {
                  tunnel: [w684 w687] -> w683
                  tunnel: w681 -> [w684 w686]
                  tunnel: w680 -> [_ w685]
                  frame False {
                  }
                  frame True {
                    n395 = invoke class="VI" method="FP.Close"(reference=w685, error in=w686) -> (error out=w687:errorcluster)  [unwired: 1 in, 2 out]
                  }
                }
              }
            }
            n396 = call <vilib>:"Add State(s) to Queue__jki_lib_state_machine.vi"("State(s) in (\"\")"=w667) -> ("States Out"=w666:string)  [unwired: 14 in]
          }
          frame "---------- Macro ----------" {
            # "Do not put any code in this frame.\n(It is a separator no-op. You can make a copy of this frame to create a new Macro frame)"
            n397 = call <vilib>:"Add State(s) to Queue__jki_lib_state_machine.vi"("State(s) in (\"\")"=w691) -> ("States Out"=w690:string)  [unwired: 14 in]
          }
          frame "Macro: Initialize" {
            w692 = "Data: Initialize\nInitialize Core Data\nUI: Initialize\nUI: Front Panel State >> Open\nDevice Ini\nMotor Config\nMove Config\nDetection Config\nCenter"  # Data: Initialize Initialize Core Data UI: Initialize UI: Front Panel State >> Open Device Ini Motor Config Move Config Detection Config Center
            # "Initialization Macro\n(This is called once, when the VI starts)"
            n398 = call <vilib>:"Add State(s) to Queue__jki_lib_state_machine.vi"("State(s) in Front (\"\")"=w692, "State(s) in (\"\")"=w696) -> ("States Out"=w695:string)  [unwired: 13 in]
          }
          frame "Macro: Exit" {
            # "Exit Macro\n(This is called once, when the VI exits)"
            n399 = Unbundle By Name(w698) -> ("Core.Close Panel on Exit?"=w697:bool)
            n400 = Select(t="UI: Front Panel State >> Close", s=w697, f="") -> (s? t:f=w701:string)
            n401 = call <vilib>:"Add State(s) to Queue__jki_lib_state_machine.vi"("State(s) in (\"\")"=w701, "State(s) at Back (\"\")"="Data: Cleanup\nExit") -> ("States Out"=w699:string)  [unwired: 13 in]
            n402 = call <vilib>:"Add State(s) to Queue__jki_lib_state_machine.vi"("State(s) in Front (\"\")"=w699, "State(s) in (\"\")"=w706) -> ("States Out"=w705:string)  [unwired: 13 in]
          }
          frame "---------- Ini and Configure ----------" {
            # "Template Separator\n(You can make a copy of, or modify, this frame)"
            n403 = call <vilib>:"Add State(s) to Queue__jki_lib_state_machine.vi"("State(s) in (\"\")"=w710) -> ("States Out"=w709:string)  [unwired: 14 in]
          }
          frame "Device Ini" {
            # "Your code here.\n(You can make a copy of, or modify, this frame)"
            n404 = flat-sequence {
              tunnel: w724 -> [w734]
              tunnel: [w734] -> w723
              tunnel: w723 -> [w737]
              tunnel: [w735] -> w718
              frame #0 {
                n405 = Wait (ms)(milliseconds to wait=u32 3000) -> ()  [unwired: 1 out]
              }
              frame #1 {
                n406 = for {
                  tunnel: w737 -> [w738] mode=indexing
                  shift-right: [w739] -> w735
                  shift-left: string[] [] -> [w740]
                  n407 = call "send command.vi"("Device Name"=w738) -> ("status"=w741:bool)  [unwired: 4 in]
                  n408 = case shown="True" w741 {
                    tunnel: w740 -> [w742 w745]
                    tunnel: [w742 w744] -> w739
                    tunnel: w738 -> [_ w743]
                    frame False {
                    }
                    frame True {
                      n409 = Build Array (concatenate)(w745, w743) -> (w744:string[])
                    }
                  }
                }
              }
            }
            n410 = for {
              N: 1 -> [_]
              shift-right: [w727] -> w717
              shift-left: timestamp[][] [] ("Time") -> [w729]
              n411 = for {
                N: 12 -> [_]
                tunnel: w729 -> [w732] mode=indexing
                tunnel: [w730] -> w727 mode=indexing
                n412 = Get Date/Time In Seconds() -> (seconds since 1Jan1904=w731:timestamp)
                n413 = Build Array (concatenate)(w732, w731) -> (w730:timestamp[])
              }
            }
            n414 = property on="Time" class="Arr (strict)"("Value"=w717) -> ()  [unwired: 2 in, 2 out]
            n415 = call <vilib>:"Add State(s) to Queue__jki_lib_state_machine.vi"("State(s) in (\"\")"=w726) -> ("States Out"=w725:string)  [unwired: 14 in]
            n416 = Bundle By Name(cluster=w719, "active cams"=w718) -> (w713:T36)
            n417 = property on="active CCDs" class="LstBox (strict)"("Item Names"=w718) -> ()  [unwired: 2 in, 2 out]
            n418 = Array Size(array=w718) -> (size(s)=w721:i32)
            n419 = Initialize Array(0.0 ("element"), w721, 0 ("dimension size")) -> (w714:dbl[][])
            n420 = Bundle By Name(cluster=w713, "Offset X stats"=w714, "Offset Y stats"=w714, "Centroid X"=w714, "Centroid Y"=w714, "Mean Centroid X"=w714, "Mean Centroid Y"=w714, "Offset X"=w714, "Offset Y"=w714, "Size"=w714, "Mean Size"=w714, "Motor X"=w714, "Motor Y"=w714) -> (w712:T36)
            "name array" <- w718
          }
          frame "Load Config" {
            # "Your code here.\n(You can make a copy of, or modify, this frame)"
            n421 = Unbundle By Name(w785) -> ("detection para"=w791:T2[], "move properties"=w788:T1[], "thresholds"=w780:cluster{"Lower value":sgl, "Upper value":sgl}[])
            n422 = call "File Dialog2"("error in"=w748, "pattern (all files)"="*.cfg", "pattern label"="config") -> ("selected path"=w795:path, "error out"=w747:errorcluster)  [unwired: 9 in, 2 out]
            n423 = property on="Load Config" class="Bool (strict)"("Value"=FALSE ("Load Config")) -> ()  [unwired: 2 in, 2 out]
            n424 = Open/Create/Replace File(file path (use dialog)=w795, error in=w747, operation (0:open)=T18."open or create") -> (refnum out=w799:refnum<file>, error out=w800:errorcluster)  [unwired: 3 in, 1 out]
            n425 = Read from Binary File(5:"output cluster 2", 8:w800, 11:w799) -> (0:w801:errorcluster, 2:w793:T4, 3:w802:refnum<file>)  [unwired: 3 in, 1 out]
            n426 = Close File(refnum=w802, error in=w801) -> (error out=w750:errorcluster)  [unwired: 1 out]
            n427 = Unbundle By Name(w793) -> ("Value"=w777:T6, "CCDs"=w792:string[], "detection para"=w790:T2[], "move properties"=w789:T1[], "thresholds"=w781:cluster{"Lower value":sgl, "Upper value":sgl}[])
            n428 = Cluster To Array(cluster=w777) -> (array=w778:u16[])
            n429 = call <vilib>:"Add State(s) to Queue__jki_lib_state_machine.vi"("State(s) in (\"\")"=w804, "State(s) at Back (\"\")"="Motor Config" ("State(s) at Back (\"\")")) -> ("States Out"=w803:string)  [unwired: 13 in]
            n430 = for {
              tunnel: w792 -> [w820]
              tunnel: w790 -> [w822]
              tunnel: w789 -> [w821]
              shift-right: [w814] -> w787
              shift-left: w791 -> [w819]
              shift-right: [w812] -> w786
              shift-left: w788 -> [w818]
              tunnel: w783 -> [w817] mode=indexing
              tunnel: w781 -> [w813]
              shift-right: [w809] -> w779
              shift-left: w780 -> [w811]
              tunnel: w778 -> [w808]
              tunnel: [w805] -> w776 mode=indexing
              i -> [w806]
              n431 = call-poly <userlib>:"Filter 1D Array__ogtk.vi"("items to filter"=w817, "array"=w820) -> ("filtered item indices"=w823:i32[])  [unwired: 4 in, 1 out]
              n432 = Index Array(array=w823) -> (element=w807:i32)  [unwired: 1 in]
              n433 = Index Array(array=w808, index=w807) -> (element=w805:u16)
              n434 = Index Array(array=w822, index=w807) -> (element=w816:T2)
              n435 = Index Array(array=w821, index=w807) -> (element=w815:T1)
              n436 = Index Array(array=w813, index=w807) -> (element=w810:cluster{"Lower value":sgl, "Upper value":sgl})
              n437 = Replace Array Subset(array=w819, new element=w816, index=w806) -> (w814:T2[])
              n438 = Replace Array Subset(array=w818, new element=w815, index=w806) -> (w812:T1[])
              n439 = Replace Array Subset(array=w811, new element=w810, index=w806) -> (w809:cluster{"Lower value":sgl, "Upper value":sgl}[])
            }
            n440 = Index Array(array=w776, index #1=0 ("index (row)"), index #2=1 ("index (row)"), index #3=2 ("index (row)"), index #4=3 ("index (row)"), index #5=4 ("index (row)"), index #6=5 ("index (row)"), index #7=6 ("index (row)"), index #8=7 ("index (row)"), index #9=8 ("index (row)"), index #10=9 ("index (row)"), index #11=10 ("index (row)"), index #12=11 ("index (row)")) -> (element #1=w763:u16, element #2=w762:u16, element #3=w761:u16, element #4=w760:u16, element #5=w759:u16, element #6=w758:u16, element #7=w757:u16, element #8=w756:u16, element #9=w755:u16, element #10=w754:u16, element #11=w753:u16, element #12=w752:u16)
            n441 = Bundle By Name(cluster=w777, "Motor CCD 1"=w763, "Motor CCD 2"=w762, "Motor CCD 3"=w761, "Motor CCD 4"=w760, "Motor CCD 5"=w759, "Motor CCD 6"=w758, "Motor CCD 7"=w757, "Motor CCD 8"=w756, "Motor CCD 9"=w755, "Motor CCD 10"=w754, "Motor CCD 11"=w753, "Motor CCD 12"=w752) -> (w751:T6)
            n442 = Bundle By Name(cluster=w785, "detection para"=w787, "move properties"=w786, "thresholds"=w779) -> (w784:T36)
            n443 = property on="associated motors" class="Clust (strict)"(error in=w750, "Val(Sgnl)"=w751) -> (error out=w749:errorcluster)  [unwired: 1 in, 1 out]
          }
          frame "Save Config" {
            # "Your code here.\n(You can make a copy of, or modify, this frame)"
            n444 = Unbundle By Name(w841) -> ("move properties"=w827:T1[], "detection para"=w836:T2[], "thresholds"=w824:cluster{"Lower value":sgl, "Upper value":sgl}[])
            n445 = property on="associated motors" class="Clust (strict)"() -> ("Value"=w835:T6)  [unwired: 2 in, 2 out]
            n446 = property on="Save Config" class="Bool (strict)"("Value"=FALSE ("Save Config")) -> ()  [unwired: 2 in, 2 out]
            n447 = local read "CCDs"() -> (w825:string[])
            n448 = call "File Dialog"("pattern (all files)"="*.cfg", "pattern label"="config") -> ("selected path"=w829:path)  [unwired: 10 in, 3 out]
            n449 = Bundle("CCDs"=w825, "move properties"=w827, "detection para"=w836, "thresholds"=w824, "Value"=w835) -> (w828:T4)  [unwired: 1 in]
            n450 = Open/Create/Replace File(file path (use dialog)=w829, error in=w833, operation (0:open)=T18."replace or create with confirmation") -> (refnum out=w837:refnum<file>, error out=w838:errorcluster)  [unwired: 3 in, 1 out]
            n451 = Write to Binary File(file (use dialog)=w837, data=w828, error in=w838) -> (refnum out=w840:refnum<file>, error out=w839:errorcluster)  [unwired: 3 in, 1 out]
            n452 = Close File(refnum=w840, error in=w839) -> (error out=w832:errorcluster)  [unwired: 1 out]
            n453 = call <vilib>:"Add State(s) to Queue__jki_lib_state_machine.vi"("State(s) in (\"\")"=w843) -> ("States Out"=w842:string)  [unwired: 14 in]
          }
          frame "active" {
            # "Your code here.\n(You can make a copy of, or modify, this frame)"
            n454 = call-poly <userlib>:"Filter 1D Array__ogtk.vi"("items to filter"=w853, "array"=w849) -> ("filtered item indices"=w852:i32[])  [unwired: 4 in, 1 out]
            n455 = Unbundle By Name(w848) -> ("move properties"=w851:T1[], "detection para"=w846:T2[])  [unwired: 1 out]
            n456 = Index Array(array=w852) -> (element=w844:i32)  [unwired: 1 in]
            n457 = Index Array(array=w851, index=w844) -> (element=w850:T1)
            n458 = Index Array(array=w846, index=w844) -> (element=w845:T2)
            n459 = property on="move config" class="Clust (strict)"("Value"=w850) -> ()  [unwired: 2 in, 2 out]
            n460 = property on="beam detection para" class="Clust (strict)"("Value"=w845) -> ()  [unwired: 2 in, 2 out]
            n461 = Bundle By Name(cluster=w848, "active ccd"=w844) -> (w847:T36)
            n462 = call <vilib>:"Add State(s) to Queue__jki_lib_state_machine.vi"("State(s) in (\"\")"=w856) -> ("States Out"=w855:string)  [unwired: 14 in]
          }
          frame "Detection Config" {
            # "Your code here.\n(You can make a copy of, or modify, this frame)"
            n463 = Unbundle By Name(w861) -> ("detection para"=w857:T2[], "active ccd"=w862:i32)
            n464 = Replace Array Subset(array=w857, new element="beam detection para", index=w862) -> (w858:T2[])
            n465 = Bundle By Name(cluster=w861, "detection para"=w858) -> (w860:T36)
            n466 = call <vilib>:"Add State(s) to Queue__jki_lib_state_machine.vi"("State(s) in (\"\")"=w865) -> ("States Out"=w864:string)  [unwired: 14 in]
          }
          frame "Motor Config" {
            # "Your code here.\n(You can make a copy of, or modify, this frame)"
            n467 = Unbundle By Name("associated motors") -> ("Motor CCD 1"=w888:u16, "Motor CCD 2"=w889:u16, "Motor CCD 3"=w890:u16, "Motor CCD 4"=w883:u16, "Motor CCD 5"=w882:u16, "Motor CCD 6"=w881:u16, "Motor CCD 7"=w880:u16, "Motor CCD 8"=w879:u16, "Motor CCD 9"=w878:u16, "Motor CCD 10"=w877:u16, "Motor CCD 11"=w876:u16, "Motor CCD 12"=w875:u16)
            n468 = local read "motor refs"() -> (w886:refnum<vi>[])
            n469 = property on="ActiveMotor 2" class="Ring (strict)"() -> ("Value"=w866:u16)  [unwired: 2 in, 2 out]
            n470 = property on="ActiveMotor" class="Ring (strict)"() -> ("Value"=w869:u16)  [unwired: 2 in, 2 out]
            n471 = property on="ActiveMotor" class="Ring (strict)"() -> ("Strings []"=w871:string[])  [unwired: 2 in, 2 out]
            n472 = Build Array(w888, w889, w890, w883, w882, w881, w880, w879, w878, w877, w876, w875) -> (w874:u16[])
            n473 = Increment(x=w874) -> (x+1=w873:u16[])
            n474 = Index Array(array=w871, index=w869) -> (element=w870:string)
            n475 = property on="ActiveMotor 2" class="Ring (strict)"() -> ("Strings []"=w867:string[])  [unwired: 2 in, 2 out]
            n476 = for {
              tunnel: w873 -> [w905] mode=indexing
              tunnel: w886 -> [w900]
              tunnel: [w894] -> w872 mode=indexing
              n477 = Multiply(x=w905, y=u16 3) -> (x*y=w901:u16)
              n478 = Subtract(x=w901, y=u16 3) -> (x-y=w899:u16)
              n479 = Subtract(x=w901, y=u16 2) -> (x-y=w898:u16)
              n480 = Index Array(array=w900, index=w899) -> (element=w897:refnum<vi>)
              n481 = Index Array(array=w900, index=w898) -> (element=w896:refnum<vi>)
              n482 = Bundle By Name(cluster="active Axis ref", "Ref X"=w897, "Ref Y"=w896) -> (w894:cluster{"Ref X":refnum<vi>, "Ref Y":refnum<vi>})
            }
            n483 = property on="ActiveMotorName::99" class="Str"("Val(Sgnl)"=w870) -> ()  [unwired: 2 in, 2 out]
            n484 = Index Array(array=w867, index=w866) -> (element=w868:string)
            n485 = property on="ActiveMotorName::98" class="Str"("Val(Sgnl)"=w868) -> ()  [unwired: 2 in, 2 out]
            n486 = call <vilib>:"Add State(s) to Queue__jki_lib_state_machine.vi"("State(s) in (\"\")"=w893) -> ("States Out"=w892:string)  [unwired: 14 in]
            n487 = Bundle By Name(cluster=w885, "active axis refs 2"=w872) -> (w884:T36)
          }
          frame "Move Config" {
            # "Your code here.\n(You can make a copy of, or modify, this frame)"
            n488 = Unbundle By Name(w907) -> ("move properties"=w911:T1[], "active ccd"=w910:i32)
            n489 = Replace Array Subset(array=w911, new element="move config", index=w910) -> (w908:T1[])
            n490 = Bundle By Name(cluster=w907, "move properties"=w908) -> (w906:T36)
            n491 = call <vilib>:"Add State(s) to Queue__jki_lib_state_machine.vi"("State(s) in (\"\")"=w914) -> ("States Out"=w913:string)  [unwired: 14 in]
          }
          frame "----------Centroid & Move----------" {
            # "Template Separator\n(You can make a copy of, or modify, this frame)"
            n492 = call <vilib>:"Add State(s) to Queue__jki_lib_state_machine.vi"("State(s) in (\"\")"=w918) -> ("States Out"=w917:string)  [unwired: 14 in]
          }
          frame "detected" {
            n493 = Unbundle By Name(w946) -> ("Offset X"=w958:dbl[][], "Offset Y"=w957:dbl[][], "Size"=w956:dbl[][], "Mean Size"=w955:dbl[][], "Time"=w951:timestamp[][], "Motor X"=w934:dbl[][], "active axis refs 2"=w932:T11, "Motor Y"=w933:dbl[][])
            n494 = Unbundle By Name(w946) -> ("active cams"=w947:string[])
            n495 = Spreadsheet String To Array(format string="%s", spreadsheet string=w922, array type (2D Dbl)=string[] []) -> (array=w928:string[])  [unwired: 1 in]
            "detected 2" <- w928
            n496 = for {
              tunnel: w929 -> [w973]
              tunnel: w928 -> [w972] mode=indexing
              tunnel: [w970] -> w924 mode=indexing
              n497 = call-poly <userlib>:"Filter 1D Array__ogtk.vi"("items to filter"=w972, "array"=w973) -> ("filtered item indices"=w971:i32[])  [unwired: 4 in, 1 out]
              n498 = Index Array(array=w971) -> (element=w970:i32)  [unwired: 1 in]
            }
            n499 = call <vilib>:"Build State String with Arguments__jki_lib_state_machine.vi"("Arguments (\"\")"=w922, "State"="stats") -> ("State with Arguments"=w921:string)  [unwired: 4 in]
            n500 = for {
              tunnel: w928 -> [w1059] mode=indexing
              tunnel: w947 -> [w1058]
              tunnel: [w1057] -> w961 mode=indexing
              n501 = Equal?(x=w1059, y=w1058) -> (x = y?=w1057:bool[])
            }
            n502 = Unbundle By Name(w946) -> ("Mean Centroid X"=w965:dbl[][], "Mean Centroid Y"=w964:dbl[][], "Centroid X"=w967:dbl[][], "Centroid Y"=w966:dbl[][])
            n503 = call <vilib>:"Add State(s) to Queue__jki_lib_state_machine.vi"("State(s) in (\"\")"=w920, "State(s) at Back (\"\")"=w921) -> ("States Out"=w919:string)  [unwired: 13 in]
            n504 = Transpose 2D Array(2D array=w961) -> (transposed array=w960:bool[][])
            n505 = for {
              tunnel: w967 -> [w1005]
              tunnel: w966 -> [w1004]
              tunnel: w965 -> [w1003]
              tunnel: w964 -> [w1002]
              tunnel: [w1001] -> w945 mode=indexing
              tunnel: [w1000] -> w962 mode=indexing
              tunnel: w960 -> [w998] mode=indexing
              tunnel: w959 -> [w997] mode=indexing
              tunnel: w958 -> [w996]
              tunnel: w957 -> [w995]
              tunnel: [w994] -> w926 mode=indexing
              tunnel: [w993] -> w949 mode=indexing
              tunnel: w956 -> [w992]
              tunnel: w955 -> [w991]
              tunnel: [w990] -> w954 mode=indexing
              tunnel: w951 -> [w989]
              tunnel: [w988] -> w950 mode=indexing
              i -> [w999]
              n506 = Or Array Elements(Boolean array=w998) -> (logical OR=w987:bool)
              n507 = case shown="True" w987 {
                tunnel: w1005 -> [_ w1056]
                tunnel: w1004 -> [_ w1055]
                tunnel: w1003 -> [w1020 w1052]
                tunnel: w1002 -> [w1019 w1051]
                tunnel: [w1018 w1048] -> w1001
                tunnel: [w1017 w1047] -> w1000
                tunnel: w999 -> [w1006 w1021]
                tunnel: w997 -> [_ w1046]
                tunnel: w996 -> [w1016 w1043]
                tunnel: w995 -> [w1015 w1042]
                tunnel: [w1014 w1037] -> w994
                tunnel: [w1013 w1036] -> w993
                tunnel: w992 -> [_ w1035]
                tunnel: w991 -> [w1012 w1033]
                tunnel: [w1011 w1030] -> w990
                tunnel: w989 -> [w1010 w1028]
                tunnel: [w1007 w1026] -> w988
                frame False {
                  n508 = Index Array(array=w1010, index (row)=w1006) -> (element=w1008:timestamp[])  [unwired: 1 in]
                  n509 = Index Array(array=w1020, index (row)=w1006) -> (element=w1018:dbl[])  [unwired: 1 in]
                  n510 = Index Array(array=w1019, index (row)=w1006) -> (element=w1017:dbl[])  [unwired: 1 in]
                  n511 = Index Array(array=w1016, index (row)=w1006) -> (element=w1014:dbl[])  [unwired: 1 in]
                  n512 = Index Array(array=w1012, index (row)=w1006) -> (element=w1011:dbl[])  [unwired: 1 in]
                  n513 = Index Array(array=w1015, index (row)=w1006) -> (element=w1013:dbl[])  [unwired: 1 in]
                  n514 = Get Date/Time In Seconds() -> (seconds since 1Jan1904=w1009:timestamp)
                  n515 = Build Array (concatenate)(w1008, w1009) -> (w1007:timestamp[])
                }
                frame True {
                  n516 = Unbundle By Name(w1046) -> ("Target.X::12"=w1025:refnum<vi>, "Target.Y::12"=w1024:refnum<vi>)
                  n517 = Index Array(array=w1052, index (row)=w1021) -> (element=w1049:dbl[])  [unwired: 1 in]
                  n518 = Index Array(array=w1051, index (row)=w1021) -> (element=w1050:dbl[])  [unwired: 1 in]
                  n519 = Index Array(array=w1056, index (row)=w1021) -> (element=w1054:dbl[])  [unwired: 1 in]
                  n520 = Index Array(array=w1055, index (row)=w1021) -> (element=w1053:dbl[])  [unwired: 1 in]
                  n521 = Index Array(array=w1043, index (row)=w1021) -> (element=w1040:dbl[])  [unwired: 1 in]
                  n522 = Index Array(array=w1042, index (row)=w1021) -> (element=w1039:dbl[])  [unwired: 1 in]
                  n523 = Index Array(array=w1035, index (row)=w1021) -> (element=w1034:dbl[])  [unwired: 1 in]
                  n524 = Index Array(array=w1033, index (row)=w1021) -> (element=w1032:dbl[])  [unwired: 1 in]
                  n525 = Index Array(array=w1028, index (row)=w1021) -> (element=w1027:timestamp[])  [unwired: 1 in]
                  n526 = property class="DigNum (strict)"(reference=w1025) -> ("Value"=w1023:dbl)  [unwired: 1 in, 2 out]
                  n527 = property class="DigNum (strict)"(reference=w1024) -> ("Value"=w1022:dbl)  [unwired: 1 in, 2 out]
                  n528 = call <vilib>:"Std Deviation and Variance.vi"("X"=w1054) -> ("mean"=w1045:dbl)  [unwired: 1 in, 2 out]
                  n529 = call <vilib>:"Std Deviation and Variance.vi"("X"=w1053) -> ("mean"=w1044:dbl)  [unwired: 1 in, 2 out]
                  n530 = call <vilib>:"Std Deviation and Variance.vi"("X"=w1034) -> ("mean"=w1031:dbl)  [unwired: 1 in, 2 out]
                  n531 = Get Date/Time In Seconds() -> (seconds since 1Jan1904=w1029:timestamp)
                  n532 = Subtract(x=w1023, y=w1045) -> (x-y=w1041:dbl)
                  n533 = Subtract(x=w1022, y=w1044) -> (x-y=w1038:dbl)
                  n534 = Build Array (concatenate)(w1049, w1045) -> (w1048:dbl[])
                  n535 = Build Array (concatenate)(w1050, w1044) -> (w1047:dbl[])
                  n536 = Build Array (concatenate)(w1032, w1031) -> (w1030:dbl[])
                  n537 = Build Array (concatenate)(w1027, w1029) -> (w1026:timestamp[])
                  n538 = Build Array (concatenate)(w1040, w1041) -> (w1037:dbl[])
                  n539 = Build Array (concatenate)(w1039, w1038) -> (w1036:dbl[])
                }
              }
            }
            n540 = for {
              tunnel: w934 -> [w986]
              tunnel: w933 -> [w985]
              tunnel: w932 -> [w984]
              tunnel: [w983] -> w931 mode=indexing
              tunnel: [w982] -> w930 mode=indexing
              tunnel: w924 -> [_] mode=indexing
              i -> [w974]
              n541 = Index Array(array=w986, index (row)=w974) -> (element=w979:dbl[])  [unwired: 1 in]
              n542 = Index Array(array=w984, index=w974) -> (element=w980:cluster{"Ref X":refnum<vi>, "Ref Y":refnum<vi>})
              n543 = Index Array(array=w985, index (row)=w974) -> (element=w975:dbl[])  [unwired: 1 in]
              n544 = Unbundle By Name(w980) -> ("Ref X"=w981:refnum<vi>, "Ref Y"=w977:refnum<vi>)
              n545 = property class="DigNum (strict)"(reference=w981) -> ("Value"=w978:dbl)  [unwired: 1 in, 2 out]
              n546 = property class="DigNum (strict)"(reference=w977) -> ("Value"=w976:dbl)  [unwired: 1 in, 2 out]
              n547 = Build Array (concatenate)(w975, w976) -> (w982:dbl[])
              n548 = Build Array (concatenate)(w979, w978) -> (w983:dbl[])
            }
            n549 = local write "Numeric"(0.0 ("Numeric")) -> ()
            n550 = Array Size(array=w926) -> (size(s)=w944:i32[])
            n551 = local read "Centroid X"() -> (w948:dbl[][])
            n552 = Index Array(array=w944, index=1) -> (element=w942:i32)
            "History index" <- w942
            n553 = local read "Size"() -> (w953:dbl[][])
            n554 = call <vilib>:"Add State(s) to Queue__jki_lib_state_machine.vi"("State(s) in (\"\")"=w919, "State(s) at Back (\"\")"="Check Move\ntdms" ("State(s) at Back (\"\")")) -> ("States Out"=w936:string)  [unwired: 13 in]
            n555 = Greater?(x=w942, y="History Size") -> (0:w940:bool)
            n556 = Bundle By Name(cluster=w946, "Centroid X"=w948, "Centroid Y"=w948, "Mean Centroid X"=w945, "Mean Centroid Y"=w962, "Offset X"=w926, "Offset Y"=w949, "Mean Size"=w954, "Size"=w953, "Time"=w950, "Motor X"=w931, "Motor Y"=w930) -> (w963:T36)
            n557 = Select(t="history" ("State(s) at Back (\"\")"), s=w940, f="") -> (s? t:f=w937:string)
            n558 = call <vilib>:"Add State(s) to Queue__jki_lib_state_machine.vi"("State(s) in (\"\")"=w936, "State(s) at Back (\"\")"=w937) -> ("States Out"=w935:string)  [unwired: 13 in]
          }
          frame "Check Move" {
            # "Your code here.\n(You can make a copy of, or modify, this frame)"
            n559 = Unbundle By Name(w1078) -> ("move properties"=w1060:T1[], "Mean Size"=w1086:dbl[][], "move properties"=w1089:T1[], "Offset X"=w1088:dbl[][], "Offset Y"=w1087:dbl[][], "active cams"=w1064:string[])
            n560 = for {
              tunnel: w1089 -> [w1145] mode=indexing
              tunnel: w1088 -> [w1147] mode=indexing
              tunnel: w1087 -> [w1146] mode=indexing
              tunnel: w1086 -> [w1144] mode=indexing
              tunnel: [w1120] -> w1085 mode=indexing
              tunnel: [w1116] -> w1084 mode=indexing
              tunnel: w1064 -> [w1141] mode=indexing
              tunnel: [w1143] -> w1083 mode=indexing
              tunnel: [w1142] -> w1080 mode=indexing
              tunnel: w1060 -> [w1140] mode=indexing
              n561 = Unbundle By Name(w1140) -> ("enable feedback"=w1119:bool)
              n562 = Unbundle By Name(w1145) -> ("Tolerance [%]"=w1134:dbl)
              n563 = Reverse 1D Array(array=w1147) -> (reversed array=w1139:dbl[])
              n564 = Reverse 1D Array(array=w1146) -> (reversed array=w1138:dbl[])
              n565 = Reverse 1D Array(array=w1144) -> (reversed array=w1133:dbl[])
              n566 = Index Array(array=w1139) -> (element=w1137:dbl)  [unwired: 1 in]
              n567 = Index Array(array=w1138) -> (element=w1136:dbl)  [unwired: 1 in]
              n568 = Index Array(array=w1133) -> (element=w1132:dbl)  [unwired: 1 in]
              n569 = Absolute Value(x=w1137) -> (abs(x)=w1127:dbl)
              n570 = Absolute Value(x=w1136) -> (abs(x)=w1123:dbl)
              n571 = Square Root(x=w1132) -> (sqrt(x)=w1131:dbl)
              n572 = Divide(x=w1134, y=100.0) -> (x/y=w1130:dbl)
              n573 = Multiply(x=w1131, y=w1130) -> (x*y=w1129:dbl)
              n574 = Not Equal To 0?(x=w1123) -> (x != 0?=w1117:bool)
              n575 = Not Equal To 0?(x=w1127) -> (x != 0?=w1122:bool)
              n576 = Greater Or Equal?(x=w1127, y=w1129) -> (x >= y?=w1121:bool)
              n577 = Greater Or Equal?(x=w1123, y=w1129) -> (x >= y?=w1118:bool)
              n578 = Compound Arithmetic op=AND(w1119, w1122, w1121) -> (w1120:bool)
              n579 = Compound Arithmetic op=AND(w1119, w1118, w1117) -> (w1116:bool)
              n580 = Boolean To (0,1)(Boolean=w1116) -> (0, 1=w1124:i16)
              n581 = Multiply(x=w1124, y=w1123) -> (x*y=w1125:dbl)
              n582 = Boolean To (0,1)(Boolean=w1120) -> (0, 1=w1128:i16)
              n583 = Multiply(x=w1128, y=w1127) -> (x*y=w1126:dbl)
              n584 = Bundle(w1125, "GUIdevice 8"=w1141) -> (w1142:cluster{dbl, "GUIdevice 8":string})  [unwired: 1 in]
              n585 = Bundle(w1126, "GUIdevice 8"=w1141) -> (w1143:cluster{dbl, "GUIdevice 8":string})  [unwired: 1 in]
            }
            "required X" <- w1085
            "required Y" <- w1084
            n586 = Sort 1D Array(array=w1080) -> (sorted array=w1081:cluster{dbl, "GUIdevice 8":string}[])
            n587 = Sort 1D Array(array=w1083) -> (sorted array=w1082:cluster{dbl, "GUIdevice 8":string}[])
            n588 = call <vilib>:"Add State(s) to Queue__jki_lib_state_machine.vi"("State(s) in (\"\")"=w1063) -> ("States Out"=w1062:string)  [unwired: 14 in]
            n589 = Reverse 1D Array(array=w1081) -> (reversed array=w1070:cluster{dbl, "GUIdevice 8":string}[])
            n590 = Reverse 1D Array(array=w1082) -> (reversed array=w1076:cluster{dbl, "GUIdevice 8":string}[])
            n591 = Empty Array?(array=w1076) -> (empty?=w1073:bool)
            n592 = Empty Array?(array=w1070) -> (empty?=w1068:bool)
            n593 = Unbundle By Name(w1078) -> ("Feedback global"=w1077:bool)
            n594 = Index Array(array=w1076) -> (element=w1066:cluster{dbl, "GUIdevice 8":string})  [unwired: 1 in]
            n595 = Index Array(array=w1070) -> (element=w1065:cluster{dbl, "GUIdevice 8":string})  [unwired: 1 in]
            n596 = Unbundle(w1066) -> (w1075:dbl)  [unwired: 1 out]
            n597 = Unbundle(w1065) -> (w1071:dbl)  [unwired: 1 out]
            n598 = Equal To 0?(x=w1075) -> (x = 0?=w1074:bool)
            n599 = Equal To 0?(x=w1071) -> (x = 0?=w1069:bool)
            n600 = property on="autodetect" class="Bool (strict)"("Value"=FALSE ("autodetect")) -> ()  [unwired: 2 in, 2 out]
            n601 = Or(x=w1074, y=w1073) -> (x .or. y?=w1072:bool)
            n602 = Or(x=w1069, y=w1068) -> (x .or. y?=w1067:bool)
            n603 = case shown="True" w1077 {
              tunnel: w1072 -> [_ w1099]
              tunnel: w1076 -> [_ w1098]
              tunnel: w1067 -> [_ w1096]
              tunnel: w1070 -> [_ w1095]
              tunnel: w1062 -> [w1092 w1094]
              tunnel: [w1092 w1093] -> w1079
              frame False {
              }
              frame True {
                n604 = case shown="False" w1099 {
                  tunnel: w1098 -> [w1114 _]
                  tunnel: w1094 -> [w1110 w1115]
                  tunnel: [w1108 w1115] -> w1097
                  frame False {
                    n605 = Index Array(array=w1114) -> (element=w1113:cluster{dbl, "GUIdevice 8":string})  [unwired: 1 in]
                    n606 = Unbundle By Name(w1113) -> ("GUIdevice 8"=w1112:string)
                    n607 = call <vilib>:"Build State String with Arguments__jki_lib_state_machine.vi"("Arguments (\"\")"=w1112, "State"="Move X") -> ("State with Arguments"=w1109:string)  [unwired: 4 in]
                    n608 = call <vilib>:"Add State(s) to Queue__jki_lib_state_machine.vi"("State(s) in (\"\")"=w1110, "State(s) at Back (\"\")"=w1109) -> ("States Out"=w1108:string)  [unwired: 13 in]
                  }
                  frame True {
                  }
                }
                n609 = case shown="False" w1096 {
                  tunnel: w1095 -> [w1106 _]
                  tunnel: w1097 -> [w1102 w1107]
                  tunnel: [w1100 w1107] -> w1093
                  frame False {
                    n610 = Index Array(array=w1106) -> (element=w1105:cluster{dbl, "GUIdevice 8":string})  [unwired: 1 in]
                    n611 = Unbundle By Name(w1105) -> ("GUIdevice 8"=w1104:string)
                    n612 = call <vilib>:"Build State String with Arguments__jki_lib_state_machine.vi"("Arguments (\"\")"=w1104, "State"="Move Y") -> ("State with Arguments"=w1101:string)  [unwired: 4 in]
                    n613 = call <vilib>:"Add State(s) to Queue__jki_lib_state_machine.vi"("State(s) in (\"\")"=w1102, "State(s) at Back (\"\")"=w1101) -> ("States Out"=w1100:string)  [unwired: 13 in]
                  }
                  frame True {
                  }
                }
              }
            }
            n614 = call <vilib>:"Add State(s) to Queue__jki_lib_state_machine.vi"("State(s) in (\"\")"=w1062, "State(s) at Back (\"\")"=w1079) -> ("States Out"=w1091:string)  [unwired: 13 in]
          }
          frame "Move X" {
            # "Your code here.\n(You can make a copy of, or modify, this frame)"
            n615 = Unbundle By Name(w1166) -> ("Offset X"=w1165:dbl[][])
            n616 = call-poly <userlib>:"Filter 1D Array__ogtk.vi"("items to filter"=w1148, "array"=w1170) -> ("filtered item indices"=w1153:i32[])  [unwired: 4 in, 1 out]
            n617 = Unbundle By Name(w1166) -> ("active axis refs 2"=w1169:T11, "move properties"=w1152:T1[])
            n618 = for {
              tunnel: w1153 -> [w1175] mode=indexing
              tunnel: w1152 -> [w1179]
              shift-right: [w1174] -> w1150
              shift-left: i32[] [] ("filtered item indices") -> [w1177]
              n619 = Index Array(array=w1179, index=w1175) -> (element=w1178:T1)
              n620 = Unbundle By Name(w1178) -> ("enable feedback"=w1176:bool)
              n621 = case shown="True" w1176 {
                tunnel: w1177 -> [w1180 w1183]
                tunnel: w1175 -> [_ w1182]
                tunnel: [w1180 w1181] -> w1174
                frame False {
                }
                frame True {
                  n622 = Build Array (concatenate)(w1183, w1182) -> (w1181:i32[])
                }
              }
            }
            n623 = Index Array(array=w1150) -> (element=w1149:i32)  [unwired: 1 in]
            n624 = Index Array(array=w1165, index (row)=w1149) -> (element=w1164:dbl[])  [unwired: 1 in]
            n625 = Reverse 1D Array(array=w1164) -> (reversed array=w1163:dbl[])
            n626 = Index Array(array=w1169, index=w1149) -> (element=w1168:cluster{"Ref X":refnum<vi>, "Ref Y":refnum<vi>})
            n627 = Index Array(array=w1163) -> (element=w1161:dbl)  [unwired: 1 in]
            n628 = Index Array(array=w1152, index=w1149) -> (element=w1167:T1)
            n629 = Unbundle By Name(w1168) -> ("Ref X"=w1157:refnum<vi>, "Ref Y"=w1156:refnum<vi>)
            n630 = Unbundle By Name(w1167) -> ("Invert Direction X"=w1158:bool, "Invert Axis"=w1162:bool, "Stepsize"=w1159:dbl, "enable feedback"=w1155:bool)
            n631 = Greater Or Equal To 0?(x=w1161) -> (x >= 0?=w1160:bool)
            n632 = call <vilib>:"Add State(s) to Queue__jki_lib_state_machine.vi"("State(s) in Front (\"\")"="Wait" ("State(s) in Front (\"\")"), "State(s) in (\"\")"=w1173) -> ("States Out"=w1172:string)  [unwired: 13 in]
            n633 = case shown="True" w1155 {
              tunnel: w1162 -> [_ w1189]
              tunnel: w1160 -> [_ w1188]
              tunnel: w1159 -> [_ w1187]
              tunnel: w1158 -> [_ w1186]
              tunnel: w1157 -> [_ w1185]
              tunnel: w1156 -> [_ w1184]
              frame False {
              }
              frame True {
                n634 = case shown="False" w1188 {
                  tunnel: w1186 -> [w1197 w1219]
                  tunnel: w1187 -> [w1195 w1217]
                  tunnel: w1189 -> [w1194 w1216]
                  tunnel: w1189 -> [w1193 w1215]
                  tunnel: w1185 -> [w1191 w1213]
                  tunnel: w1184 -> [w1190 w1212]
                  frame True {
                    n635 = case shown="False" w1194 {
                      tunnel: [w1208 w1210] -> w1196
                      tunnel: w1191 -> [w1209 _]
                      tunnel: w1190 -> [_ w1211]
                      frame False {
                        n636 = property class="DigNum (strict)"(reference=w1209) -> ("Value"=w1208:dbl)  [unwired: 1 in, 2 out]
                      }
                      frame True {
                        n637 = property class="DigNum (strict)"(reference=w1211) -> ("Value"=w1210:dbl)  [unwired: 1 in, 2 out]
                      }
                    }
                    n638 = case shown="False" w1197 {
                      tunnel: w1196 -> [w1204 w1207]
                      tunnel: w1195 -> [w1203 w1206]
                      tunnel: [w1202 w1205] -> w1192
                      frame False {
                        n639 = Add(x=w1204, y=w1203) -> (x+y=w1202:dbl)
                      }
                      frame True {
                        n640 = Subtract(x=w1207, y=w1206) -> (x-y=w1205:dbl)
                      }
                    }
                    n641 = case shown="False" w1193 {
                      tunnel: w1192 -> [w1198 w1200]
                      tunnel: w1191 -> [w1199 _]
                      tunnel: w1190 -> [_ w1201]
                      frame False {
                        n642 = property class="DigNum (strict)"(reference=w1199, "Val(Sgnl)"=w1198) -> ()  [unwired: 1 in, 2 out]
                      }
                      frame True {
                        n643 = property class="DigNum (strict)"(reference=w1201, "Val(Sgnl)"=w1200) -> ()  [unwired: 1 in, 2 out]
                      }
                    }
                  }
                  frame False {
                    n644 = case shown="False" w1216 {
                      tunnel: [w1230 w1232] -> w1218
                      tunnel: w1213 -> [w1231 _]
                      tunnel: w1212 -> [_ w1233]
                      frame False {
                        n645 = property class="DigNum (strict)"(reference=w1231) -> ("Value"=w1230:dbl)  [unwired: 1 in, 2 out]
                      }
                      frame True {
                        n646 = property class="DigNum (strict)"(reference=w1233) -> ("Value"=w1232:dbl)  [unwired: 1 in, 2 out]
                      }
                    }
                    n647 = case shown="False" w1219 {
                      tunnel: w1218 -> [w1226 w1229]
                      tunnel: w1217 -> [w1225 w1228]
                      tunnel: [w1224 w1227] -> w1214
                      frame False {
                        n648 = Subtract(x=w1226, y=w1225) -> (x-y=w1224:dbl)
                      }
                      frame True {
                        n649 = Add(x=w1229, y=w1228) -> (x+y=w1227:dbl)
                      }
                    }
                    n650 = case shown="False" w1215 {
                      tunnel: w1214 -> [w1220 w1222]
                      tunnel: w1213 -> [w1221 _]
                      tunnel: w1212 -> [_ w1223]
                      frame False {
                        n651 = property class="DigNum (strict)"(reference=w1221, "Val(Sgnl)"=w1220) -> ()  [unwired: 1 in, 2 out]
                      }
                      frame True {
                        n652 = property class="DigNum (strict)"(reference=w1223, "Val(Sgnl)"=w1222) -> ()  [unwired: 1 in, 2 out]
                      }
                    }
                  }
                }
              }
            }
            "Arguments X" <- w1148
            "Moving X" <- w1148
          }
          frame "Move Y" {
            # "Your code here.\n(You can make a copy of, or modify, this frame)"
            n653 = Unbundle By Name(w1252) -> ("Offset Y"=w1251:dbl[][])
            n654 = call-poly <userlib>:"Filter 1D Array__ogtk.vi"("items to filter"=w1234, "array"=w1256) -> ("filtered item indices"=w1240:i32[])  [unwired: 4 in, 1 out]
            n655 = Unbundle By Name(w1252) -> ("active axis refs 2"=w1255:T11, "move properties"=w1238:T1[])
            n656 = for {
              tunnel: w1240 -> [w1261] mode=indexing
              tunnel: w1238 -> [w1265]
              shift-right: [w1260] -> w1239
              shift-left: i32[] [] ("filtered item indices") -> [w1263]
              n657 = Index Array(array=w1265, index=w1261) -> (element=w1264:T1)
              n658 = Unbundle By Name(w1264) -> ("enable feedback"=w1262:bool)
              n659 = case shown="True" w1262 {
                tunnel: w1263 -> [w1266 w1269]
                tunnel: w1261 -> [_ w1268]
                tunnel: [w1266 w1267] -> w1260
                frame False {
                }
                frame True {
                  n660 = Build Array (concatenate)(w1269, w1268) -> (w1267:i32[])
                }
              }
            }
            n661 = Index Array(array=w1239) -> (element=w1236:i32)  [unwired: 1 in]
            n662 = Index Array(array=w1251, index (row)=w1236) -> (element=w1250:dbl[])  [unwired: 1 in]
            n663 = Reverse 1D Array(array=w1250) -> (reversed array=w1249:dbl[])
            n664 = Index Array(array=w1255, index=w1236) -> (element=w1254:cluster{"Ref X":refnum<vi>, "Ref Y":refnum<vi>})
            n665 = Index Array(array=w1249) -> (element=w1247:dbl)  [unwired: 1 in]
            n666 = Index Array(array=w1238, index=w1236) -> (element=w1253:T1)
            n667 = Unbundle By Name(w1254) -> ("Ref Y"=w1243:refnum<vi>, "Ref X"=w1242:refnum<vi>)
            n668 = Unbundle By Name(w1253) -> ("Invert Direction Y"=w1244:bool, "Invert Axis"=w1248:bool, "Stepsize"=w1245:dbl, "enable feedback"=w1241:bool)
            n669 = Greater Or Equal To 0?(x=w1247) -> (x >= 0?=w1246:bool)
            n670 = call <vilib>:"Add State(s) to Queue__jki_lib_state_machine.vi"("State(s) in Front (\"\")"="Wait" ("State(s) in Front (\"\")"), "State(s) in (\"\")"=w1259) -> ("States Out"=w1258:string)  [unwired: 13 in]
            n671 = case shown="True" w1241 {
              tunnel: w1248 -> [_ w1275]
              tunnel: w1246 -> [_ w1274]
              tunnel: w1245 -> [_ w1273]
              tunnel: w1244 -> [_ w1272]
              tunnel: w1243 -> [_ w1271]
              tunnel: w1242 -> [_ w1270]
              frame False {
              }
              frame True {
                n672 = case shown="True" w1274 {
                  tunnel: w1272 -> [w1283 w1305]
                  tunnel: w1273 -> [w1281 w1303]
                  tunnel: w1275 -> [w1280 w1302]
                  tunnel: w1275 -> [w1279 w1301]
                  tunnel: w1271 -> [w1277 w1299]
                  tunnel: w1270 -> [w1276 w1298]
                  frame True {
                    n673 = case shown="False" w1280 {
                      tunnel: [w1294 w1296] -> w1282
                      tunnel: w1277 -> [w1295 _]
                      tunnel: w1276 -> [_ w1297]
                      frame False {
                        n674 = property class="DigNum (strict)"(reference=w1295) -> ("Value"=w1294:dbl)  [unwired: 1 in, 2 out]
                      }
                      frame True {
                        n675 = property class="DigNum (strict)"(reference=w1297) -> ("Value"=w1296:dbl)  [unwired: 1 in, 2 out]
                      }
                    }
                    n676 = case shown="False" w1283 {
                      tunnel: w1282 -> [w1290 w1293]
                      tunnel: w1281 -> [w1289 w1292]
                      tunnel: [w1288 w1291] -> w1278
                      frame False {
                        n677 = Add(x=w1290, y=w1289) -> (x+y=w1288:dbl)
                      }
                      frame True {
                        n678 = Subtract(x=w1293, y=w1292) -> (x-y=w1291:dbl)
                      }
                    }
                    n679 = case shown="False" w1279 {
                      tunnel: w1278 -> [w1284 w1286]
                      tunnel: w1277 -> [w1285 _]
                      tunnel: w1276 -> [_ w1287]
                      frame False {
                        n680 = property class="DigNum (strict)"(reference=w1285, "Val(Sgnl)"=w1284) -> ()  [unwired: 1 in, 2 out]
                      }
                      frame True {
                        n681 = property class="DigNum (strict)"(reference=w1287, "Val(Sgnl)"=w1286) -> ()  [unwired: 1 in, 2 out]
                      }
                    }
                  }
                  frame False {
                    n682 = case shown="False" w1302 {
                      tunnel: [w1316 w1318] -> w1304
                      tunnel: w1299 -> [w1317 _]
                      tunnel: w1298 -> [_ w1319]
                      frame False {
                        n683 = property class="DigNum (strict)"(reference=w1317) -> ("Value"=w1316:dbl)  [unwired: 1 in, 2 out]
                      }
                      frame True {
                        n684 = property class="DigNum (strict)"(reference=w1319) -> ("Value"=w1318:dbl)  [unwired: 1 in, 2 out]
                      }
                    }
                    n685 = case shown="False" w1305 {
                      tunnel: w1304 -> [w1312 w1315]
                      tunnel: w1303 -> [w1311 w1314]
                      tunnel: [w1310 w1313] -> w1300
                      frame False {
                        n686 = Subtract(x=w1312, y=w1311) -> (x-y=w1310:dbl)
                      }
                      frame True {
                        n687 = Add(x=w1315, y=w1314) -> (x+y=w1313:dbl)
                      }
                    }
                    n688 = case shown="False" w1301 {
                      tunnel: w1300 -> [w1306 w1308]
                      tunnel: w1299 -> [w1307 _]
                      tunnel: w1298 -> [_ w1309]
                      frame False {
                        n689 = property class="DigNum (strict)"(reference=w1307, "Val(Sgnl)"=w1306) -> ()  [unwired: 1 in, 2 out]
                      }
                      frame True {
                        n690 = property class="DigNum (strict)"(reference=w1309, "Val(Sgnl)"=w1308) -> ()  [unwired: 1 in, 2 out]
                      }
                    }
                  }
                }
              }
            }
            "Arguments Y" <- w1234
            "Moving Y" <- w1234
          }
          frame "Wait" {
            # "Your code here.\n(You can make a copy of, or modify, this frame)"
            n691 = flat-sequence {
              frame #0 {
                n692 = Wait (ms)(milliseconds to wait=u32 300) -> ()  [unwired: 1 out]
              }
              frame #1 {
                n693 = property on="Moving Y" class="Str"("Value"="") -> ()  [unwired: 2 in, 2 out]
                n694 = property on="Moving X" class="Str"("Value"="") -> ()  [unwired: 2 in, 2 out]
              }
            }
            n695 = call <vilib>:"Add State(s) to Queue__jki_lib_state_machine.vi"("State(s) in (\"\")"=w1325) -> ("States Out"=w1324:string)  [unwired: 14 in]
            n696 = local read "Mean Centroid X"() -> (w1320:dbl[][])
            n697 = Bundle By Name(cluster=w1322, "Mean Centroid X"=w1320, "Mean Centroid Y"=w1320) -> (w1321:T36)
          }
          frame "stats" {
            # "Your code here.\n(You can make a copy of, or modify, this frame)"
            n698 = Unbundle By Name(w1334) -> ("Offset X"=w1333:dbl[][], "Offset Y"=w1332:dbl[][], "Time"=w1331:timestamp[][], "Motor X"=w1330:dbl[][], "Motor Y"=w1329:dbl[][])
            n699 = for {
              tunnel: w1332 -> [w1372]
              tunnel: w1331 -> [w1373]
              tunnel: w1333 -> [w1374]
              tunnel: [w1377] -> w1360 mode=indexing
              tunnel: w1330 -> [w1371]
              tunnel: w1329 -> [w1370]
              tunnel: w1335 -> [_] mode=indexing
              i -> [w1364]
              n700 = Index Array(array=w1372, index (row)=w1364) -> (element=w1368:dbl[])  [unwired: 1 in]
              n701 = Index Array(array=w1371, index (row)=w1364) -> (element=w1366:dbl[])  [unwired: 1 in]
              n702 = Index Array(array=w1370, index (row)=w1364) -> (element=w1365:dbl[])  [unwired: 1 in]
              n703 = Index Array(array=w1374, index (row)=w1364) -> (element=w1369:dbl[])  [unwired: 1 in]
              n704 = Index Array(array=w1373, index (row)=w1364) -> (element=w1367:timestamp[])  [unwired: 1 in]
              n705 = Bundle("Time"=w1367, "Motor X"=w1366) -> (w1376:cluster{"Time":timestamp[], "Motor X":dbl[]})  [unwired: 1 in]
              n706 = Bundle("Time"=w1367, "Motor Y"=w1365) -> (w1375:cluster{"Time":timestamp[], "Motor Y":dbl[]})  [unwired: 1 in]
              n707 = Bundle("Time"=w1367, "Offset X"=w1369) -> (w1378:cluster{"Time":timestamp[], "Offset X":dbl[]})  [unwired: 1 in]
              n708 = Bundle("Time"=w1367, "Offset Y"=w1368) -> (w1379:cluster{"Time":timestamp[], "Offset Y":dbl[]})  [unwired: 1 in]
              n709 = Build Array(w1379, w1378, w1376, w1375) -> (w1377:cluster{"Time":timestamp[], "Motor Y":dbl[]}[])
            }
            n710 = call <vilib>:"Add State(s) to Queue__jki_lib_state_machine.vi"("State(s) in (\"\")"=w1363) -> ("States Out"=w1362:string)  [unwired: 14 in]
            n711 = Index Array(array=w1360, index (row) #1=0 ("index (row)"), index (row) #2=1 ("index (row)"), index (row) #3=2 ("index (row)"), index (row) #4=3 ("index (row)"), index (row) #5=4 ("index (row)"), index (row) #6=5 ("index (row)"), index (row) #7=6 ("index (row)"), index (row) #8=7 ("index (row)"), index (row) #9=8 ("index (row)"), index (row) #10=9 ("index (row)"), index (row) #11=10 ("index (row)"), index (row) #12=11 ("index (row)")) -> (element #1=→"CCD 1":cluster{"Time":timestamp[], "Motor Y":dbl[]}[], element #2=→"CCD 2":cluster{"Time":timestamp[], "Motor Y":dbl[]}[], element #3=→"CCD 3":cluster{"Time":timestamp[], "Motor Y":dbl[]}[], element #4=→"CCD 4":cluster{"Time":timestamp[], "Motor Y":dbl[]}[], element #5=→"CCD 5":cluster{"Time":timestamp[], "Motor Y":dbl[]}[], element #6=→"CCD 6":cluster{"Time":timestamp[], "Motor Y":dbl[]}[], element #7=→"CCD 7":cluster{"Time":timestamp[], "Motor Y":dbl[]}[], element #8=→"CCD 8":cluster{"Time":timestamp[], "Motor Y":dbl[]}[], element #9=→"CCD 9":cluster{"Time":timestamp[], "Motor Y":dbl[]}[], element #10=→"CCD 10":cluster{"Time":timestamp[], "Motor Y":dbl[]}[], element #11=→"CCD 11":cluster{"Time":timestamp[], "Motor Y":dbl[]}[], element #12=→"CCD 12":cluster{"Time":timestamp[], "Motor Y":dbl[]}[])  [unwired: 12 in]
          }
          frame "---------------Statistics--------------" {
            # "Template Separator\n(You can make a copy of, or modify, this frame)"
            n712 = call <vilib>:"Add State(s) to Queue__jki_lib_state_machine.vi"("State(s) in (\"\")"=w1383) -> ("States Out"=w1382:string)  [unwired: 14 in]
          }
          frame "Save Stats" {
            # "Your code here.\n(You can make a copy of, or modify, this frame)"
            n713 = property on="CCD 1" class="XYGraph (strict)"() -> ("Value"=w1393:cluster{timestamp[], dbl[]}[])  [unwired: 2 in, 2 out]
            n714 = property on="CCD 2" class="XYGraph (strict)"() -> ("Value"=w1392:cluster{timestamp[], dbl[]}[])  [unwired: 2 in, 2 out]
            n715 = property on="CCD 3" class="XYGraph (strict)"() -> ("Value"=w1391:cluster{timestamp[], dbl[]}[])  [unwired: 2 in, 2 out]
            n716 = property on="CCD 4" class="XYGraph (strict)"() -> ("Value"=w1390:cluster{timestamp[], dbl[]}[])  [unwired: 2 in, 2 out]
            n717 = property on="CCD 5" class="XYGraph (strict)"() -> ("Value"=w1389:cluster{timestamp[], dbl[]}[])  [unwired: 2 in, 2 out]
            n718 = property on="CCD 6" class="XYGraph (strict)"() -> ("Value"=w1388:cluster{timestamp[], dbl[]}[])  [unwired: 2 in, 2 out]
            n719 = property on="CCD 7" class="XYGraph (strict)"() -> ("Value"=w1387:cluster{timestamp[], dbl[]}[])  [unwired: 2 in, 2 out]
            n720 = property on="CCD 8" class="XYGraph (strict)"() -> ("Value"=w1386:cluster{timestamp[], dbl[]}[])  [unwired: 2 in, 2 out]
            n721 = Build Array(w1393, w1392, w1391, w1390, w1389, w1388, w1387, w1386) -> (w1385:cluster{timestamp[], dbl[]}[][])
            n722 = for {
              tunnel: w1385 -> [w1401] mode=indexing
              tunnel: w1384 -> [w1400] mode=indexing
              n723 = Empty String/Path?(string/path=w1400) -> (empty?=w1399:bool)
              n724 = case shown="False" w1399 {
                tunnel: w1401 -> [w1407 _]
                tunnel: w1400 -> [w1405 _]
                frame False {
                  n725 = Index Array(array=w1407, index #1=0 ("index"), index #2=1 ("index"), index #3=2 ("index"), index #4=3 ("index")) -> (element #1=w1442:cluster{timestamp[], dbl[]}, element #2=w1436:cluster{timestamp[], dbl[]}, element #3=w1435:cluster{timestamp[], dbl[]}, element #4=w1434:cluster{timestamp[], dbl[]})  [unwired: 1 in, 1 out]
                  n726 = Concatenate Strings(w1405, ".dat" ("string")) -> (w1403:string)
                  n727 = Unbundle(w1442) -> (w1441:timestamp[], w1419:dbl[])
                  n728 = Unbundle(w1436) -> (w1410:dbl[])  [unwired: 1 out]
                  n729 = Unbundle(w1435) -> (w1409:dbl[])  [unwired: 1 out]
                  n730 = Unbundle(w1434) -> (w1408:dbl[])  [unwired: 1 out]
                  n731 = Build Path(base path="save path", name or relative path=w1403) -> (appended path=w1402:path)
                  n732 = for {
                    tunnel: w1441 -> [w1444] mode=indexing
                    tunnel: [w1443] -> w1417 mode=indexing
                    n733 = Format Date/Time String(time format string (%c)="%Y%m%d%H%M%S", seconds (now)=w1444) -> (date/time string=w1443:string)  [unwired: 1 in]
                  }
                  n734 = Array Size(array=w1419) -> (size(s)=w1420:i32)
                  n735 = Number To Fractional String(number=w1419) -> (F-format string=w1416:string[])  [unwired: 3 in]
                  n736 = Number To Fractional String(number=w1410) -> (F-format string=w1413:string[])  [unwired: 3 in]
                  n737 = Number To Fractional String(number=w1409) -> (F-format string=w1412:string[])  [unwired: 3 in]
                  n738 = Number To Fractional String(number=w1408) -> (F-format string=w1411:string[])  [unwired: 3 in]
                  n739 = Initialize Array("", w1420, 5 ("dimension size")) -> (w1418:string[][])
                  n740 = Insert Into Array(array=w1418, index (col)=0 ("disabled index (col)"), new element=w1417) -> (w1428:string[][])  [unwired: 1 in]
                  n741 = Insert Into Array(array=w1428, index (col)=1 ("disabled index (col)"), new element=w1416) -> (w1427:string[][])  [unwired: 1 in]
                  n742 = Insert Into Array(array=w1427, index (col)=2 ("disabled index (col)"), new element=w1413) -> (w1431:string[][])  [unwired: 1 in]
                  n743 = Insert Into Array(array=w1431, index (col)=3 ("disabled index (col)"), new element=w1412) -> (w1432:string[][])  [unwired: 1 in]
                  n744 = Insert Into Array(array=w1432, index (col)=4 ("disabled index (col)"), new element=w1411) -> (w1433:string[][])  [unwired: 1 in]
                  n745 = Insert Into Array(array=w1433, index (row)=0, new element=string[] ["time", "Centroid X", "Centroid Y", "Motor Axis 1", "Motor Axis 2"] ("new element/subarray 2")) -> (w1415:string[][])  [unwired: 1 in]
                  n746 = call-poly <vilib>:"Write To Spreadsheet File.vi"("2D data"=w1415, "file path (dialog if empty)"=w1402) -> ()  [unwired: 6 in, 1 out]
                }
                frame True {
                }
              }
            }
            n747 = call <vilib>:"Add State(s) to Queue__jki_lib_state_machine.vi"("State(s) in (\"\")"=w1398) -> ("States Out"=w1397:string)  [unwired: 14 in]
            n748 = property on="Save Stats" class="Bool (strict)"("Value"=FALSE ("Save Stats")) -> ()  [unwired: 2 in, 2 out]
          }
          frame "tdms" {
            w1451 = 5400.0 ("new tdms")
            # "Your code here.\n(You can make a copy of, or modify, this frame)"
            n749 = Unbundle By Name(w1470) -> ("tdms file out"=w1467:refnum<k34>, "Offset X"=w1469:dbl[][], "Offset Y"=w1464:dbl[][], "active axis refs 2"=w1466:T11)
            n750 = for {
              tunnel: w1469 -> [w1515]
              tunnel: w1464 -> [w1514]
              tunnel: w1468 -> [w1478] mode=indexing
              tunnel: w1467 -> [w1479]
              tunnel: w1466 -> [w1500]
              tunnel: w1465 -> [w1484]
              tunnel: [w1482] -> w1463
              i -> [w1501]
              n751 = Index Array(array=w1515, index (row)=w1501) -> (element=w1513:dbl[])  [unwired: 1 in]
              n752 = Index Array(array=w1514, index (row)=w1501) -> (element=w1512:dbl[])  [unwired: 1 in]
              n753 = Index Array(array=w1500, index=w1501) -> (element=w1499:cluster{"Ref X":refnum<vi>, "Ref Y":refnum<vi>})
              n754 = Reverse 1D Array(array=w1512) -> (reversed array=w1510:dbl[])
              n755 = Reverse 1D Array(array=w1513) -> (reversed array=w1511:dbl[])
              n756 = Unbundle By Name(w1499) -> ("Ref X"=w1498:refnum<vi>, "Ref Y"=w1497:refnum<vi>)
              n757 = Index Array(array=w1511) -> (element=w1509:dbl)  [unwired: 1 in]
              n758 = Index Array(array=w1510) -> (element=w1508:dbl)  [unwired: 1 in]
              n759 = property class="DigNum (strict)"(reference=w1498, error in=w1484) -> (error out=w1483:errorcluster, "Value"=w1492:dbl)  [unwired: 1 out]
              n760 = Build Array(w1509) -> (w1481:dbl[])
              n761 = Build Array(w1508) -> (w1503:dbl[])
              n762 = Get Date/Time In Seconds() -> (seconds since 1Jan1904=w1480:timestamp)
              n763 = Build Array(w1480) -> (w1476:timestamp[])
              n764 = property class="DigNum (strict)"(reference=w1497, error in=w1483) -> (error out=w1474:errorcluster, "Value"=w1486:dbl)  [unwired: 1 out]
              n765 = Build Array(w1492) -> (w1491:dbl[])
              n766 = TDMS Write(0:w1479, 5:w1478, 7:"time", 9:w1476, 11:w1474) -> (4:w1475:refnum<k34>, 15:w1473:errorcluster)  [unwired: 1 in, 2 out]
              n767 = Build Array(w1486) -> (w1485:dbl[])
              n768 = TDMS Write(0:w1475, 5:w1478, 7:"centroid X", 9:w1481, 11:w1473) -> (4:w1506:refnum<k34>, 6:w1505:string, 15:w1504:errorcluster)  [unwired: 1 in, 1 out]
              n769 = TDMS Write(0:w1506, 5:w1505, 7:"centroid Y", 9:w1503, 11:w1504) -> (4:w1495:refnum<k34>, 6:w1494:string, 15:w1496:errorcluster)  [unwired: 1 in, 1 out]
              n770 = TDMS Write(0:w1495, 5:w1494, 7:"Motor Axis 1", 9:w1491, 11:w1496) -> (4:w1490:refnum<k34>, 6:w1489:string, 15:w1487:errorcluster)  [unwired: 1 in, 1 out]
              n771 = TDMS Write(0:w1490, 5:w1489, 7:"Motor Axis 2", 9:w1485, 11:w1487) -> (15:w1482:errorcluster)  [unwired: 1 in, 3 out]
            }
            n772 = property on="millisecond timer value" class="DigNum (strict)"() -> ("Value"=w1457:u32)  [unwired: 2 in, 2 out]
            n773 = local read "millisecond timer 2"() -> (w1459:u32)
            n774 = Tick Count (ms)() -> (millisecond timer value=w1458:u32)
            n775 = call <userlib>:"Tick Count (ms)__ogtk.vi"("error in (no error)"=w1463) -> ("error out"=w1460:errorcluster, "millisecond timer value"=w1462:u32)  [unwired: 9 in]
            n776 = Subtract(x=w1458, y=w1457) -> (x-y=w1456:u32)
            n777 = Subtract(x=w1462, y=w1459) -> (x-y=→"Waveform Chart":u32)
            n778 = Divide(x=w1456, y=u32 1000) -> (x/y=w1454:dbl)
            n779 = Quotient & Remainder(x=w1454, y=w1451) -> (x-y*floor(x/y)=w1453:dbl)  [unwired: 1 out]
            n780 = Subtract(x=w1451, y=20.0) -> (x-y=w1449:dbl)
            n781 = Greater?(x=w1453, y=w1449) -> (0:w1452:bool)
            n782 = Select(t="newtdms", s=w1452, f="") -> (s? t:f=w1446:string)
            n783 = call <vilib>:"Add State(s) to Queue__jki_lib_state_machine.vi"("State(s) in (\"\")"=w1472, "State(s) at Back (\"\")"=w1446) -> ("States Out"=w1471:string)  [unwired: 13 in]
          }
          frame "Reset History" {
            # "Your code here.\n(You can make a copy of, or modify, this frame)"
            n784 = for {
              N: 1 -> [_]
              shift-right: [w1525] -> w1517
              shift-left: timestamp[][] [] ("Time") -> [w1527]
              n785 = for {
                N: 12 -> [_]
                tunnel: w1527 -> [w1530] mode=indexing
                tunnel: [w1528] -> w1525 mode=indexing
                n786 = Get Date/Time In Seconds() -> (seconds since 1Jan1904=w1529:timestamp)
                n787 = Build Array (concatenate)(w1530, w1529) -> (w1528:timestamp[])
              }
            }
            n788 = local read "Offset X"() -> (w1516:dbl[][])
            n789 = Bundle By Name(cluster=w1521, "Offset X"=w1516, "Offset Y"=w1516, "Time"=w1517, "Motor X"=w1516) -> (w1520:T36)
            n790 = call <vilib>:"Add State(s) to Queue__jki_lib_state_machine.vi"("State(s) in (\"\")"=w1524) -> ("States Out"=w1523:string)  [unwired: 14 in]
          }
          frame "New Category: 2" {
            # "Your code here.\n(You can make a copy of, or modify, this frame)"
            n791 = call <vilib>:"Add State(s) to Queue__jki_lib_state_machine.vi"("State(s) in (\"\")"=w1534) -> ("States Out"=w1533:string)  [unwired: 14 in]
          }
          frame "newtdms" {
            # "Your code here.\n(You can make a copy of, or modify, this frame)"
            n792 = Unbundle By Name(w1538) -> ("tdms file out"=w1537:refnum<k34>)
            n793 = TDMS Close(8:w1536, 11:w1537) -> (0:w1535:errorcluster)  [unwired: 1 out]
            n794 = Get Date/Time In Seconds() -> (seconds since 1Jan1904=w1551:timestamp)
            n795 = Format Date/Time String(time format string (%c)="%Y%m%d%H%M", seconds (now)=w1551) -> (date/time string=w1541:string)  [unwired: 1 in]
            n796 = Concatenate Strings(w1541, "Beampointing_Pico.tdms" ("string")) -> (w1548:string)
            n797 = String To Path(string=w1548) -> (path=w1549:path)
            n798 = Build Path(base path=path "W:/BP_DATA", name or relative path=w1549) -> (appended path=w1543:path)
            n799 = TDMS Open(6:FALSE ("disable buffering (T)"), 7:enum16{"1.0", "2.0"}."1.0" ("file format version (2.0)"), 8:w1535, 10:T16."create or replace" ("operation"), 11:w1543) -> (0:w1542:errorcluster, 3:w1540:refnum<k34>)  [unwired: 1 in]
            n800 = call <vilib>:"Add State(s) to Queue__jki_lib_state_machine.vi"("State(s) in (\"\")"=w1554) -> ("States Out"=w1553:string)  [unwired: 14 in]
            n801 = Bundle By Name(cluster=w1538, "tdms file out"=w1540) -> (w1539:T36)
          }
          frame "Center" {
            # "Your code here.\n(You can make a copy of, or modify, this frame)"
            n802 = property on="Center" class="Bool (strict)"("Value"=FALSE ("Center")) -> ()  [unwired: 2 in, 2 out]
            n803 = control-ref of="image::1"() -> (w1569:refnum<vi>)
            n804 = control-ref of="image::2"() -> (w1568:refnum<vi>)
            n805 = control-ref of="image::3"() -> (w1567:refnum<vi>)
            n806 = control-ref of="image::4"() -> (w1566:refnum<vi>)
            n807 = control-ref of="image::5"() -> (w1565:refnum<vi>)
            n808 = control-ref of="image::6"() -> (w1564:refnum<vi>)
            n809 = control-ref of="image::7"() -> (w1563:refnum<vi>)
            n810 = control-ref of="image::8"() -> (w1562:refnum<vi>)
            n811 = control-ref of="image::9"() -> (w1561:refnum<vi>)
            n812 = control-ref of="image::10"() -> (w1560:refnum<vi>)
            n813 = control-ref of="image::11"() -> (w1559:refnum<vi>)
            n814 = control-ref of="image::12"() -> (w1558:refnum<vi>)
            n815 = for {
              tunnel: w1555 -> [w1582] mode=indexing
              tunnel: [w1577] -> w1570 mode=indexing
              n816 = Unbundle By Name(w1582) -> ("Target.X::12"=w1581:refnum<vi>, "Target.Y::12"=w1580:refnum<vi>)
              n817 = property class="DigNum (strict)"(reference=w1581) -> ("Value"=w1579:dbl)  [unwired: 1 in, 2 out]
              n818 = property class="DigNum (strict)"(reference=w1580) -> ("Value"=w1578:dbl)  [unwired: 1 in, 2 out]
              n819 = Bundle("Value"=w1579, "Value"=w1578) -> (w1577:cluster{"Value":dbl, "Value":dbl})  [unwired: 1 in]
            }
            n820 = call <vilib>:"Add State(s) to Queue__jki_lib_state_machine.vi"("State(s) in (\"\")"=w1574) -> ("States Out"=w1573:string)  [unwired: 14 in]
            n821 = Build Array(w1569, w1568, w1567, w1566, w1565, w1564, w1563, w1562, w1561, w1560, w1559, w1558) -> (w1557:refnum<vi>[])
            n822 = for {
              tunnel: w1557 -> [w1576] mode=indexing
              tunnel: w1570 -> [w1575] mode=indexing
              n823 = property class="ImageControl"(reference=w1576, "Image Center Position"=w1575) -> ()  [unwired: 1 in, 2 out]
            }
          }
          frame "history" {
            # "Your code here.\n(You can make a copy of, or modify, this frame)"
            n824 = Unbundle By Name(w1592) -> ("Offset X"=w1598:dbl[][], "Offset Y"=w1597:dbl[][], "Mean Centroid X"=w1596:dbl[][], "Mean Centroid Y"=w1595:dbl[][], "Motor X"=w1594:dbl[][], "Motor Y"=w1593:dbl[][], "Time"=w1584:timestamp[][])
            n825 = for {
              tunnel: w1598 -> [w1616] mode=indexing
              tunnel: w1597 -> [w1614] mode=indexing
              tunnel: w1596 -> [w1613] mode=indexing
              tunnel: w1595 -> [w1612] mode=indexing
              tunnel: w1594 -> [w1611] mode=indexing
              tunnel: w1593 -> [w1610] mode=indexing
              tunnel: [w1615] -> w1590 mode=indexing
              tunnel: [w1609] -> w1589 mode=indexing
              tunnel: [w1605] -> w1588 mode=indexing
              tunnel: [w1608] -> w1587 mode=indexing
              tunnel: [w1607] -> w1586 mode=indexing
              tunnel: [w1606] -> w1585 mode=indexing
              tunnel: w1584 -> [w1604] mode=indexing
              tunnel: [w1602] -> w1583 mode=indexing
              w1603 = 0
              n826 = Delete From Array(array=w1611, index=w1603) -> (array with subset deleted=w1607:dbl[])  [unwired: 1 in, 1 out]
              n827 = Delete From Array(array=w1610, index=w1603) -> (array with subset deleted=w1606:dbl[])  [unwired: 1 in, 1 out]
              n828 = Delete From Array(array=w1604, index=w1603) -> (array with subset deleted=w1602:timestamp[])  [unwired: 1 in, 1 out]
              n829 = Delete From Array(array=w1613, index=w1603) -> (array with subset deleted=w1605:dbl[])  [unwired: 1 in, 1 out]
              n830 = Delete From Array(array=w1612, index=w1603) -> (array with subset deleted=w1608:dbl[])  [unwired: 1 in, 1 out]
              n831 = Delete From Array(array=w1614, index=w1603) -> (array with subset deleted=w1609:dbl[])  [unwired: 1 in, 1 out]
              n832 = Delete From Array(array=w1616, index=w1603) -> (array with subset deleted=w1615:dbl[])  [unwired: 1 in, 1 out]
            }
            n833 = call <vilib>:"Add State(s) to Queue__jki_lib_state_machine.vi"("State(s) in (\"\")"=w1601) -> ("States Out"=w1600:string)  [unwired: 14 in]
            n834 = Bundle By Name(cluster=w1592, "Offset X"=w1590, "Offset Y"=w1589, "Mean Centroid X"=w1588, "Mean Centroid Y"=w1587, "Motor X"=w1586, "Motor Y"=w1585, "Time"=w1583) -> (w1591:T36)
          }
        }
        n835 = property on="Box" class="Arr (strict)"() -> ("Value"=w265:T5)  [unwired: 2 in, 2 out]
        n836 = for {
          tunnel: w267 -> [w294]
          tunnel: w266 -> [w295]
          tunnel: w258 -> [w287] mode=indexing
          tunnel: w265 -> [w288] mode=indexing
          n837 = call-poly <userlib>:"Filter 1D Array__ogtk.vi"("items to filter"=w287, "array"=w295) -> ("filtered item indices"=w296:i32[])  [unwired: 4 in, 1 out]
          n838 = Index Array(array=w296) -> (element=w290:i32)  [unwired: 1 in]
          n839 = Index Array(array=w294, index=w290) -> (element=w293:T29)
          n840 = Unbundle By Name(w293) -> ("Target.X::12"=w298:refnum<vi>, "Target.Y::12"=w297:refnum<vi>)
          n841 = property class="DigNum (strict)"(reference=w298) -> ("Value"=w292:dbl)  [unwired: 1 in, 2 out]
          n842 = property class="DigNum (strict)"(reference=w297) -> ("Value"=w291:dbl)  [unwired: 1 in, 2 out]
          n843 = call "draw crosshair imaq.vi"("Color"=u32 16774656, "Target.Y"=w291, "size"=cluster{"xhair size":dbl, "xhair size 2":dbl} {"xhair size"=25.0, "xhair size 2"=25.0}, "Target.X"=w292, "Bounding Rectangle"=T14 {"Left"=0, "Top"=0, "Right"=0, "Bottom"=0}, "image in"=w287) -> ("image out"=w286:T8)  [unwired: 4 in, 1 out]
          n844 = call "draw box imaq.vi"("Color"=u32 1244928, "Rectangle"=w288, "image in"=w286) -> ()  [unwired: 8 in, 1 out]
        }
        n845 = property on="ActiveMotor" class="Ring (strict)"() -> ("Strings []"=w260:string[])  [unwired: 2 in, 2 out]
        n846 = Index Array(array=w260, index="ActiveMotor") -> (element=w261:string)
        n847 = Not Equal?(x="ActiveMotorName::99", y=w261) -> (x != y?=w262:bool)
        n848 = case shown="True" w262 {
          tunnel: w260 -> [_ w284]
          tunnel: "ActiveMotorName::99" -> [_ w283]
          frame False {
          }
          frame True {
            n849 = Search 1D Array(1D array=w284, element=w283) -> (index of element=w282:i32)  [unwired: 1 in]
            n850 = property on="ActiveMotor" class="Ring (strict)"("Value"=w282) -> ()  [unwired: 2 in, 2 out]
          }
        }
        n851 = property on="ActiveMotor 2" class="Ring (strict)"() -> ("Strings []"=w253:string[])  [unwired: 2 in, 2 out]
        n852 = Index Array(array=w253, index="ActiveMotor 2") -> (element=w256:string)
        n853 = Not Equal?(x="ActiveMotorName::98", y=w256) -> (x != y?=w255:bool)
        n854 = case shown="True" w255 {
          tunnel: w253 -> [_ w281]
          tunnel: "ActiveMotorName::98" -> [_ w280]
          frame False {
          }
          frame True {
            n855 = Search 1D Array(1D array=w281, element=w280) -> (index of element=w279:i32)  [unwired: 1 in]
            n856 = property on="ActiveMotor 2" class="Ring (strict)"("Value"=w279) -> ()  [unwired: 2 in, 2 out]
          }
        }
      }
      n857 = control-ref of="This Application"() -> (w243:refnum<vi>)
      n858 = control-ref of="This VI"() -> (w247:refnum<vi>)
      n859 = Current VI's Menubar() -> (w246:refnum<k9>)
      n860 = call "GUI_Master_subvi_reentrant_queues.vi"("This Application"=w243, "error in (no error)"=w244, "tcp data event"=w242, "Caller menu reference"=w246, "Caller VI ref"=w247) -> ("error out"=→"error IO 2":errorcluster)  [unwired: 6 in]
      n861 = Unbundle By Name(w132) -> ("tdms file out"=w131:refnum<k34>)
      n862 = for {
        tunnel: w161 -> [w251] mode=indexing
        tunnel: w160 -> [w250]
        tunnel: [w249] -> w130
        n863 = call "IMAQ Dispose"("Image"=w251, "error in (no error)"=w250) -> ("error out"=w249:errorcluster)  [unwired: 4 in]
      }
      n864 = TDMS Close(8:w130, 11:w131) -> (0:→"error out 2":errorcluster)  [unwired: 1 out]
    }
  }
